vi "CPT Control 12.1.vi"() -> ()   [LabVIEW 2015]
uses:
  <vilib>/Analysis/baseanly.llb/Mean (DBL).vi
  <vilib>/Analysis/baseanly.llb/Normalize Vector.vi
  <vilib>/Utility/file.llb/Read From Spreadsheet File (string).vi
  <vilib>/Utility/file.llb/Write To Spreadsheet File (string).vi
  <vilib>/Utility/file.llb/Write To Spreadsheet File (DBL).vi
  <vilib>/Analysis/2dsp.llb/1D Cross Correlation (DBL).vi
  <vilib>/Utility/file.llb/Read Delimited Spreadsheet (DBL).vi
  <vilib>/Analysis/NI_AALBase.lvlib
  <vilib>/Analysis/NI_AALPro.lvlib
panel:
  in  "Set volume change threshold":bool
  out "size(s) 2":i32
  out "size(s)":i32
  in  "fre3":dbl
  out "Pore Offset:":dbl
  out "Side Offset:":dbl
  out "Axial Offset:":dbl
  in  "SET Pump Offsets":bool
  in  "Pore Offset SOLL":dbl
  in  "Side Offset Soll":dbl
  in  "Axial Offset Soll":dbl
  out "Stop Distance IS":dbl min=0.0 max=20.0 format="%#_f mm"
  in  "Stop Distance":dbl=20.0 min=0.0 max=20.0 format="%#_g mm"
  out "reset_flag":bool
  out "Time Loop":u32 format="%.0f ms"
  out "Pre-shearing output":dbl
  out "ms Offset":u32
  out "Test Flag":bool
  out "Date/Time:":string
  in  "Notaus":bool
  in  "Settings Tab":T1(tab)
  out "Axial Pressure":T2(graph)
  out "Side Pressure":T2(graph)
  out "Pore Pressure":T2(graph)
  in  "Visualize data":bool
  in  "SET Pump Pressures":bool
  out "Porepressure":dbl format="%#_4f kPa"
  out "Axialpressure":dbl format="%#_4f kPa"
  out "Sidepressure":dbl format="%#_4f kPa"
  in  "Soll Pore Pressure":dbl min=-200.0 max=4900.0 format="%#_3f kPa"
  in  "Soll Axial Pressure":dbl min=-200.0 max=4000.0 format="%#_3f kPa"
  in  "Soll Side Pressure":dbl min=-200.0 max=4000.0 format="%#_3f kPa"
  in  "Activate Manuel Control":bool
  in  "Schieberegler":dbl(slide) min=-1.0 max=1.0 scale=1.0..-1.0
  out "Position Piston":dbl(slide)
  in  "Move":bool
  out "Contact?":bool
  out "Force Sensor":dbl format="%#_4g N"
  in  "Go - Seitendruck":bool
  in  "Go - Axialdruck":bool
  in  "Velocity Linear":dbl=200.0 format="%#_g kPa/Min"
  in  "Up_Lower":bool
  in  "Delta Pore":dbl format="%#_g kPa"
  in  "GO All Pressure":bool
  in  "Delta Seiten":dbl format="%#_g kPa"
  in  "Delta Axial":dbl format="%#_g kPa"
  in  "Go - Porendruck":bool
  out "Velocity deviation":T3(graph)
  out "Acceleration":T3(graph)
  in  "Enable static penetration":bool
  in  "Finish test":bool
  in  "Set file":bool
  in  "Static peneration test":path
  in  "Vibro test 3":path
  in  "Vibro test 1":path
  in  "Static penetration Depth(mm) - 4":dbl
  in  "Time delay - 4":dbl
  in  "Enable Vibro Mode 2":bool
  in  "Enable Vibro Mode 3":bool
  in  "Depth(mm)3":dbl
  in  "Background velocity-3":dbl
  in  "Amplitdue-3":dbl
  in  "freq-3 ( Hz) 2":dbl
  in  "Time delay-3":dbl
  in  "Depth(mm)2":dbl
  in  "Background velocity-2":dbl
  in  "Amplitdue-2":dbl
  in  "freq-2 ( Hz)":dbl
  in  "Switch Vibro Mode":bool
  in  "Control start":bool
  in  "Control Stop":bool
  in  "Activate":bool
  out "Velocity vs Controller output":cluster{dbl[], dbl[]}[](graph)
  out "Correlation curve":dbl[](graph)
  out "time shift steps":sgl format="%.2f"
  in  "Visualize data":bool
  in  "Start Correlation":bool
  out "Intercept b":dbl
  out "Slope m":dbl
  in  "Time delay-2":dbl
  in  "Enable Vibro Mode 1":bool
  in  "Vibration frequency - 1  (Hz)":dbl
  in  "background velocity -1 (mm/s)":dbl
  in  "Amplitude - 1 (mm)":dbl
  in  "Vibro test 2":path
  in  "SET P/I Value":bool
  in  "Set auto file name":bool
  in  "SET Vibro Settings":bool
  out "Vibro Test IS":bool
  out "Frequency IS":dbl min=0.0 max=40.0 format="%#_g Hz"
  out "Amplitude IS":dbl=1.0 min=0.0 max=40.0 format="%#_g mm"
  out "Feeding IS":dbl min=0.0 max=20.0 format="%#_f mm/s"
  in  "New Path":string
  out "Path Logging":path
  in  "Set New Path":bool
  in  "VibroTest":bool=TRUE
  in  "Frequency SOLL":dbl=5.0 min=0.0 max=40.0 format="%#_g Hz"
  in  "Amplitude SOLL":dbl=3.0 min=0.0 max=40.0 format="%#_g mm"
  in  "Vorschub SOLL":dbl=20.0 min=0.0 max=20.0 format="%#_g mm/s"
  in  "Record Data":bool
  out "Record Flag":bool
  in  "start penetration":bool
  out "Boolean":bool
  in  "Soll I-Value":i32 min=-200 max=4000
  in  "Soll P-Value":i32 min=-200 max=4900
  out "IS I-Value":i32
  out "IS P-Value":i32
  out "Axial Pressure okay:":bool
  out "Side Pressure okay:":bool
  out "Pore Pressure okay:":bool
  in  "Circumference Control":bool
  in  "Turn off BC5":bool
  in  "SET Pre-Shearing":bool
  in  "Number of Cycles SOLL":dbl format="%#_f"
  in  "Duration of Cycle SOLL":i32
  in  "Amplitude Cycle SOLL":i32
  in  "Start Pre-Shearing":bool
  out "Pre-Shearing Ended Successful:":bool
  in  "Sollwert Porenwasser":dbl
  in  "Sollwert Seitendruck":dbl
  in  "Huang Su Calibration File":path
  out "IS Parameter 1":dbl=-163.9 format="%#_g x^6 +"
  out "IS Parameter 2":dbl=-163.9 format="%#_g x^5 +"
  out "IS Parameter 3":dbl=-163.9 format="%#_g x^4 +"
  out "IS Parameter 4":dbl=-163.9 format="%#_g x^3 +"
  out "IS Parameter 5":dbl=-163.9 format="%#_g x^2 +"
  out "IS Parameter 6":dbl=-163.9 format="%#_g x     +"
  out "IS Parameter 7":dbl=-163.9
  in  "SET Huang Su":bool
  in  "SOLL Parameter 1":dbl=-163.9 format="%#_g x^6 +"
  in  "SOLL Paramter 2":dbl=-163.9 format="%#_g x^5 +"
  in  "SOLL Parameter 3":dbl=-163.9 format="%#_g x^4 +"
  in  "SOLL Parameter 4":dbl=-163.9 format="%#_g x^3 +"
  in  "SOLL Parameter 5":dbl=-163.9 format="%#_g x^2 +"
  in  "SOLL Parameter 6":dbl=-163.9 format="%#_g x     +"
  in  "SOLL Parameter 7":dbl=-163.9
  out "Piston Position (mm)":dbl[](graph)
  out "Linear calibration":cluster{"array":dbl[], "array":dbl[]}(graph)
  in  "Calibration start":bool
  in  "Soll Slope-Strain":dbl
  in  "Soll Intercept-strain":dbl
  in  "Set button":bool
  out "IS-ADWIN":dbl
  out "IS- ADWIN":dbl
  in  "Initial cone position (mm)":dbl
  in  "Starting penetration depth (mm)  2":dbl
  in  "initial radius r0":dbl
  out "Timer Leackage":dbl format="%#_g s"
  out "Axial Leackage":dbl format="%.2f ml/m"
  out "Side Leackage":dbl format="%.2f ml/m"
  out "Pore Leackage":dbl format="%.2f ml/m"
  in  "Reset Leackage":bool
  out "Axial Kp:":dbl=40.0
  out "Axial Ki:":dbl format="%.2f"
  out "Side Kp:":dbl=40.0
  out "Side Ki:":dbl format="%.2f"
  out "Pore Kp:":dbl=40.0
  out "Pore Ki:":dbl format="%.2f"
  in  "SET Pump Controls":bool
  out "Modus":i32
  in  "Kpa":dbl=40.0
  in  "Kia":dbl=0.2 format="%.1f"
  in  "Kps":dbl=40.0
  in  "Kis":dbl=0.2 format="%.1f"
  in  "Kpp":dbl=40.0
  in  "Kip":dbl=0.2 format="%.1f"
  in  "Set":bool
  out "Side Offset: 2":dbl
  out "Axial Offset: 2":dbl
  out "Pore Offset: 2":dbl
  in  "Axial Offset Soll 2":dbl
  in  "Side Offset Soll 2":dbl
  in  "Pore Offset SOLL 2":dbl
  out "ms Offset Pre-Shearing":u32
  out "Seitendruck save":dbl format="%#.0f"
  out "Axialdruck save":dbl format="%#.0f"
  out "Porendruck save":dbl format="%#.0f"
  in  "View Tab":T4(tab)
  in  "Reset_left_graph":bool
  out "Recording":bool
  out "LVDT 3":dbl format="%0.3f mm"
  out "LVDT 2":dbl format="%0.3f mm"
  out "ml Pore Linear":dbl(slide) scale=0.0..1015.0
  out "ml Side Linear":dbl(slide) scale=0.0..1009.0
  out "ml Axial Linear":dbl(slide) scale=0.0..1014.5
  out "Pore":dbl format="%#_4g ml"
  out "Side":dbl format="%#_4g ml"
  out "Axial":dbl format="%#_4g ml"
  out "Addional Side Pressure":dbl format="%.2f kPa"
  out "Max Expansion":dbl format="%.2f mm"
  out "LVDT 1":dbl format="%0.3f mm"
  in  "Regelung Akiv Axial":bool
  in  "Regelung Akiv Sidepressure":bool
  in  "Regelung Akiv Porepress":bool
  out "Axial Pressure  [KPa]":dbl format="%#.2f kPa"
  out "Side Pressure  [KPa]":dbl format="%#.2f kPa"
  out "Pore Pressure [KPa]":dbl format="%#.2f kPa"
  out "ml Fontpanel":cluster{"mean":dbl, "mean":dbl, "mean":dbl}(graph)
  out "LVDT Frontpannel":cluster{"mean":dbl, "mean":dbl, "mean":dbl}(graph)
  out "Interner Kraftsensor [MPa]":cluster{"Y":dbl[], "Y":dbl[]}[](graph) caption="XY-Graph"
  out "Notaus Activ":bool
  out "Linear Control On":bool
  out "Test Started":bool
  out "Ready":bool
  out "Manuel Control":bool
  out "Pump Control On":bool
  out "Hold Position":bool
  out "Test ended":bool
  out "Penetration ongoing":bool
  out "Cone Tip Resistance":dbl format="%0.2f"
  out "Pore Pressure":dbl format="%0.2f"
  in  "Activate Pumps/Piston Controls":bool
  out "Cone Pressure":cluster{dbl, "mean":dbl}(graph)
  out "Distance Graph":T2(graph)
  out "Linear regression":cluster{dbl[], dbl[]}[](graph)
  out "Controller Output":T2(graph)
  out "Displacement control error (mm)":dbl[](graph)
  out "Regelung Out":dbl(graph)
  out "Valve Is":dbl(graph)
  out "SOLL IS Distance":cluster{dbl, dbl}(graph)
  in  "Stop/Start":bool
  out "Axialdruck [Pa] 4":dbl(graph)
  out "Seitendruck [Pa] 3":dbl(graph)
  out "Porendruck [Pa] 2":dbl(graph)
  in  "Reset Alarm":bool
  out "Side Alarm":bool
  in  "Erlaubte Max Abweichung Side":dbl
  in  "Erlaubte  Max Abweichung Pore":dbl
  in  "Erlaubte Max Abweichung Axial":dbl
  out "Sollvorgabe":T5(graph)
  out "S":u32
  out "Total Elapsed Seconds":dbl
  out "Alarm Triggered":bool
  out "Abweichung Side":dbl format="%#_4g"
  out "Pore Alarm":bool
  out "Axial Alarm":bool
  out "Abweichung Pore":dbl format="%#_4g"
  out "Abweichung Axial":dbl format="%#_5g"
  in  "volumetric strain":dbl
  in  "Display":bool
  out "Side volume - Effective lateral Stress":cluster{"Y":dbl[], "Y":dbl[]}[](graph)
  in  "LCT control finish":bool
  out "LCT test finish":bool
  out "Strain curve based on side volume change":sgl(graph)
  in  "LCT strain-based control activate":bool
  out "Change of side volume (ml)/ actual volumetric strain":sgl format="%.2f"
  in  "maximum acceptable \nside volume change (ml)":dbl
  in  "Trigger condition\n of Stop loading":T6(ring)=enum."Set volume change threshold"
  # "Activate Manuel Piston Control"
  # "Velocity Piston"
  # "Up"
  # "Down"
  # "IS-ADwin:"
  # "Set Value:"
  # "Pore Pressure:"
  # "Side Pressure"
  # "Axial Pressure"
  # "Linear Pressure Control"
  # "Decreasing"
  # "Increasing"
  # "Delta Pore"
  # "Delta Side"
  # "Delta Axial"
  # "Vibro Settings"
  # "IS-ADwin:"
  # "Set Value:"
  # "Feeding:"
  # "Vibro Test ON:"
  # "Amplitude:"
  # "Frequency:"
  # "Controller Settings"
  # "IS-ADwin:"
  # "Set Value:"
  # "Kp:"
  # "Ki:"
  # "End of Test"
  # "IS-ADwin:"
  # "Set Value:"
  # "IS-ADwin:"
  # "Set Value:"
  # "Leackage Indicator"
  # "IS-ADwin:"
  # "Set Value:"
  # "Control"
  # "Pressure"
  # "reset"
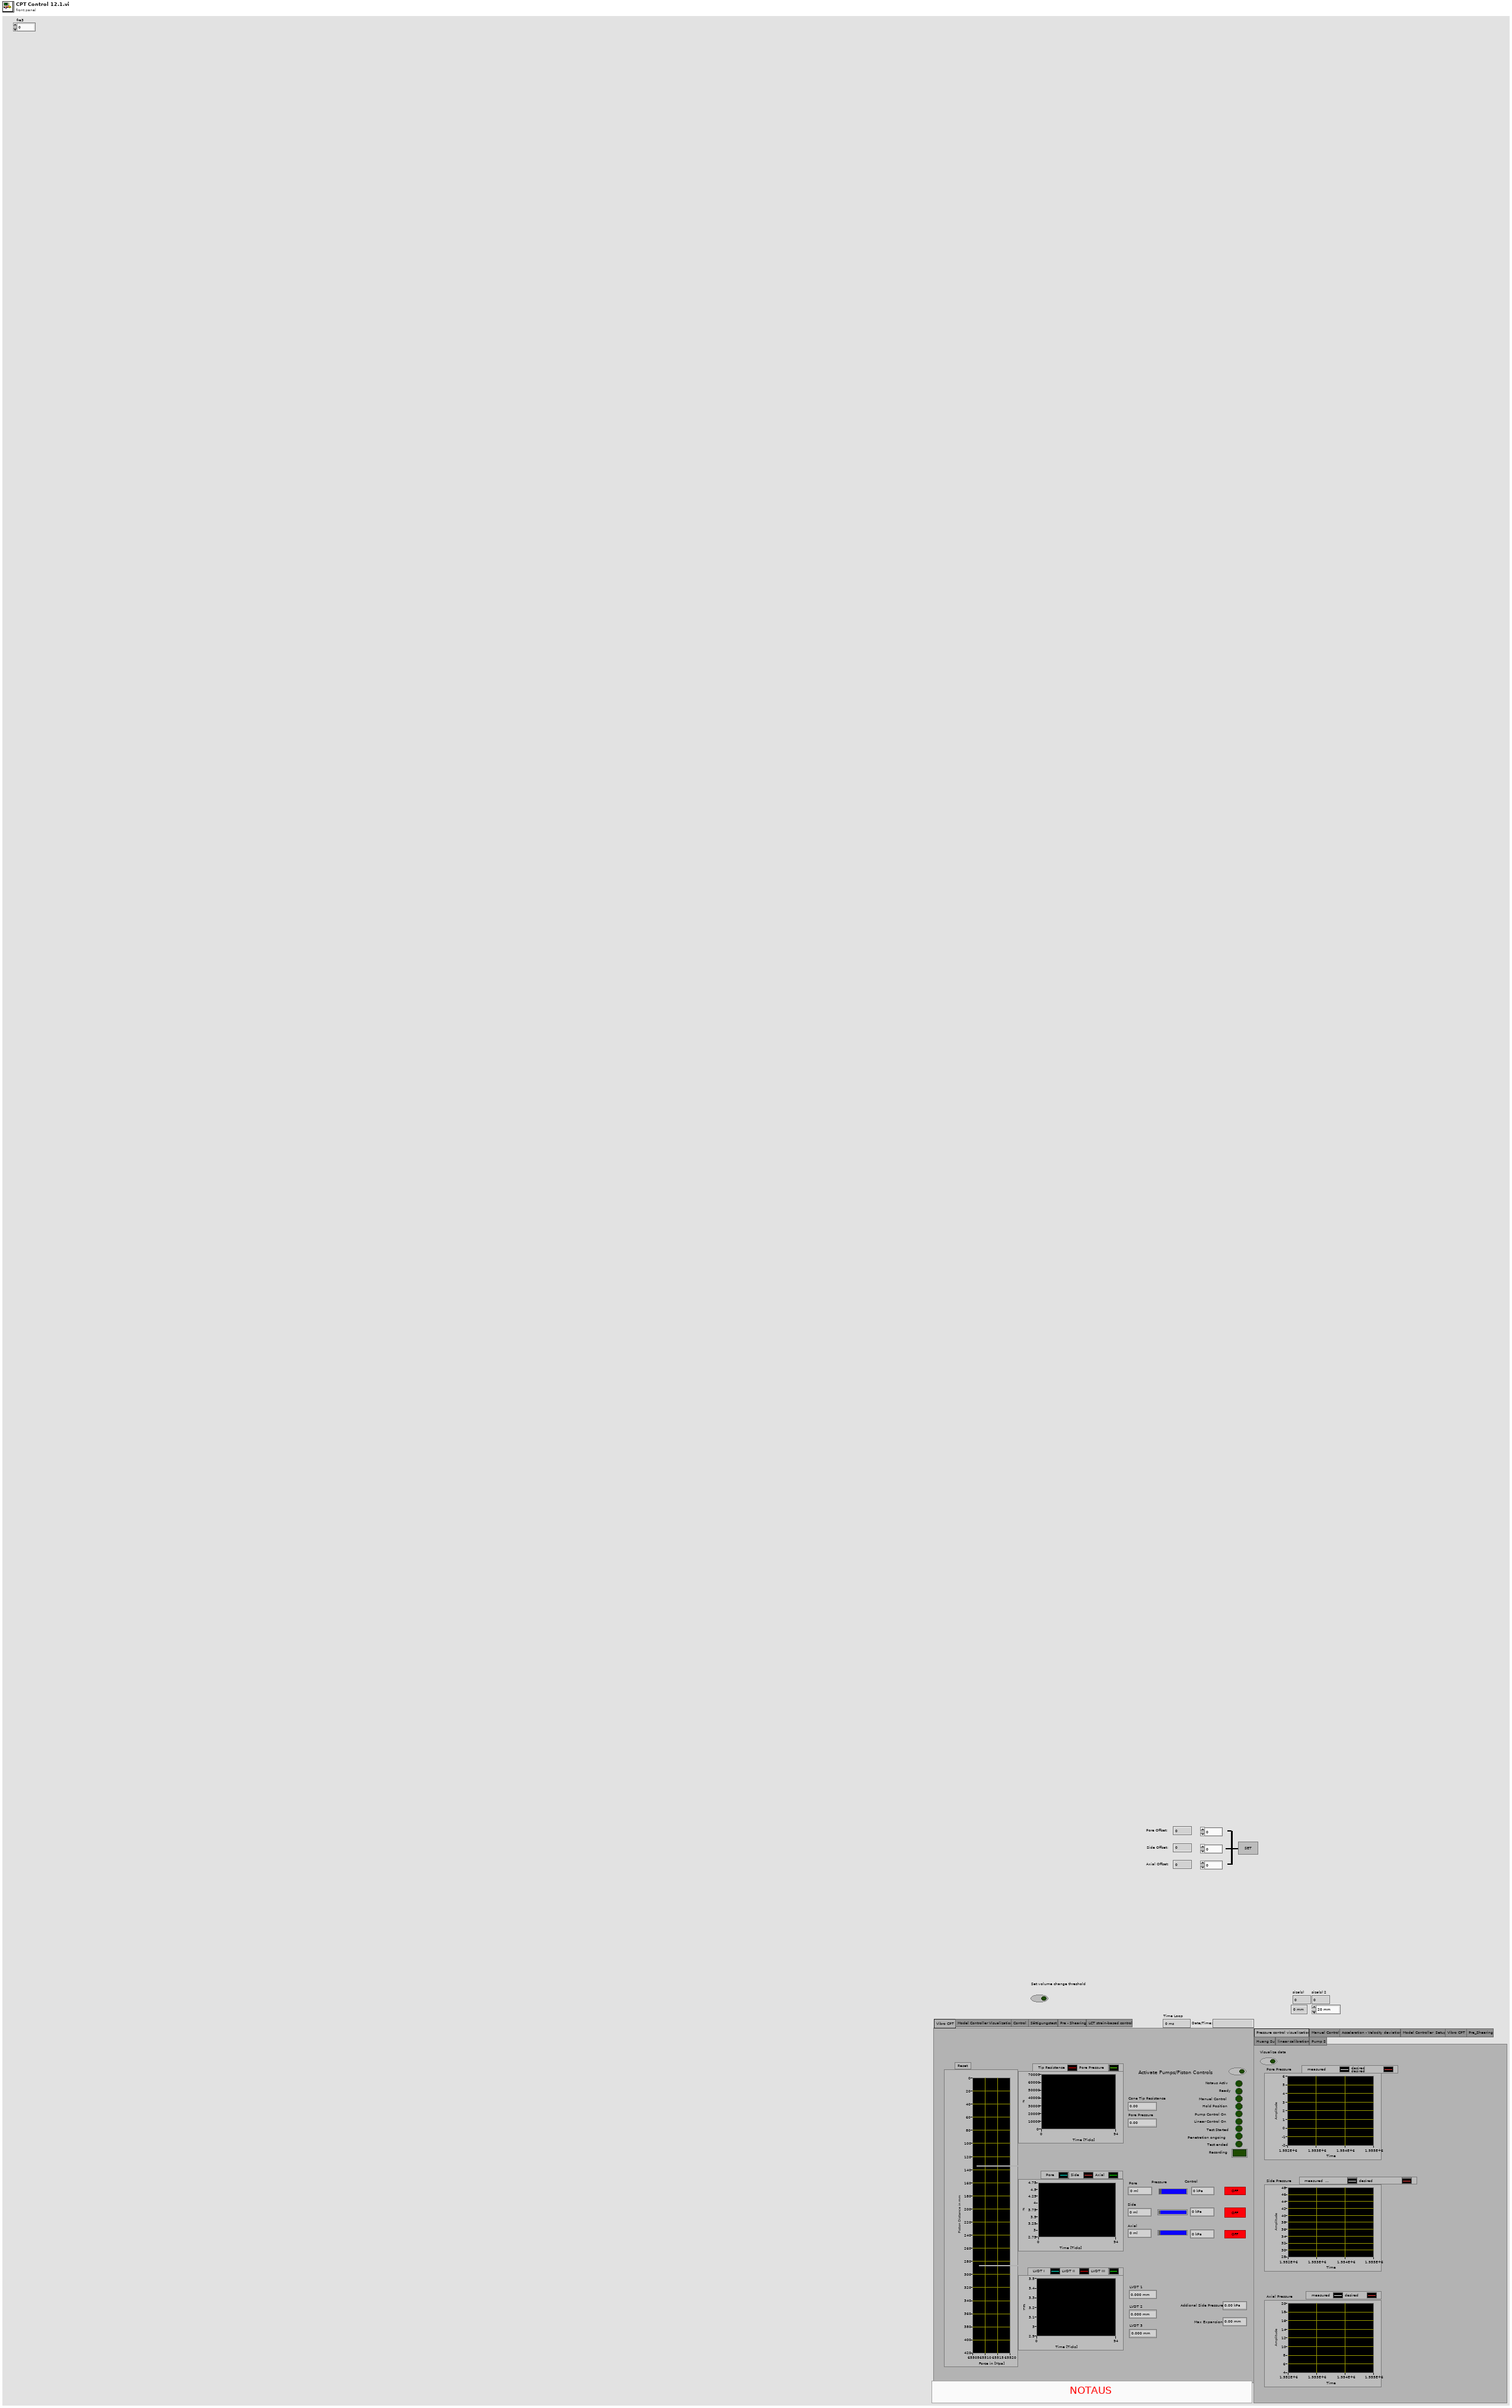
[diagram p1: front panel]
types:
  T1 = enum32{"Pressure control visualization", "Manuel Control", "Acceleration - Velocity deviation", "Model Controller  Setup", "Vibro CPT", "Pre_Shearing", "Huang Su", "linear calibration", "Pump S"}
  T2 = cluster{"Output Array":dbl[], "Output Array":dbl[]}[]
  T3 = cluster{"Output Array":dbl[], "Output Array 2":dbl[]}
  T4 = enum32{"Vibro CPT", "Model Controller Visualization", "Control", "Sättigungstest", "Pre - Shearing", "LCT strain-based control"}
  T5 = cluster{"Axial Pressure  [KPa]":dbl, "Pre-shearing output":dbl}
  T6 = enum16{"set strain for pore\n volume tric strain", "Set volume change threshold"}
  T7 = enum8{"Enabled", "Disabled", "Disabled and Grayed Out"}
  T8 = enum16{"Program Counter", "Force ", "Position Induktiv", "Position Laser", "Laser 01", "Axial Stellwert", "LVDT 1", "LVDT 2", "LVDT 3", "Pore Pressure", "Side Pressure ", "Axial Pressure", "Pore Volumen", "Side Volumen ", "Axial Volumen ", "NaN", "LVDT Max", "Side Addtional Pressure", "Stellwert Regler", "Cone  Pore Pressure ", "Cone  Side Pressure ", "Valve Kolbenposition", "Regelanweichung", "Regelabweichung Summe ", ""}
  T9 = enum16{"Program Counter", "Force ", "Position Induktiv", "PorePress_regout", "SidePress_regout", "AxialPress_regout", "LVDT 1", "LVDT 2", "LVDT 3", "Pore Pressure", "Side Pressure ", "Axial Pressure", "Pore Volumen", "Side Volumen ", "Axial Volumen ", "Soll_Porepress", "Soll_Sidepress", "Soll_axialpress", "LVDT_max", "desired distance", "predict distance", "fitted velocity", "Valve IST", "Tip resistance", "Pore pressure", "Distance_Regout", "velocity data", "estimated_Distance_Regout", "normalize vel", "normalize Distance_regout", "strain", "additional side pressure", "initial_depth", "Distance_digital", "initial volume", "actual volume", "actual side volume"}
  T10 = enum16{"NaN", "WegInd_Digits", "Valve_IST", "KraftHTM_Digits", "WegInd_Delta", "WegLaser_Digits", "Laser_O1", "Laser_M3", "LVDT_2", "LVDT_3", "LVDT_1", "PorePress_Digits", "AxialPress_Digits", "SidePress_Digits", "SpindelA_Digits", "SpindelB_Digits", "SpindelC_Digits", "FPAR_17", "Slope_calibration", "Intercept_calibration", "PorePressOffset", "AxialPressOffset", "SidePressOffset", "FPAR_23", "FPAR_24", "Vorschub", "Sinusfrequenz_Vibro", "Amplitude_Vibro", "PreShearingOutput", "FPAR_29", "FPAR_30", "FPAR_31", "FPAR_32", "FPAR_33", "FPAR_34", "FPAR_35", "FPAR_36", "FPAR_37", "FPAR_38", "FPAR_39", "Kp_Porepress", "Ki_Porepress", "Kp_Sidepress", "Ki_Sidepress", "Kp_Axialpress", "Ki_Axialpress", "FPAR_46", "FPAR_47", "FPAR_48", "FPAR_49", "FPAR_50", "PaProMin", "FPAR_52", "FPAR_53", "FPAR_54", "Huang_Su_par_1", "Huang_Su_par_2", "Huang_Su_par_3", "Huang_Su_par_4", "Huang_Su_par_5", "FPAR_60", "FPAR_61", "Huang_Su_par_6", "Huang_Su_par_7", "FPAR_64", "FPAR_65", "FPAR_66", "Model_PreShearing", "Model_Vibro", "FPAR_69", "FPAR_70", "FPAR_71", "Set_Soll_PorePressure", "Set_Soll_AxialPressure", "Set_Soll_SidePressure", "Soll_PorePressure", "Soll_AxialPressure", "Soll_SidePressure", "Taktzeit", "Abtastfrequenz", "Clock"}
  T11 = enum16{"NaN", "WegInd_Digits", "Valve_IST", "KraftHTM_Digits", "WegInd_Delta", "WegLaser_Digits", "Laser_O1", "Laser_M3", "LVDT_2", "LVDT_3", "LVDT_1", "PorePress_Digits", "AxialPress_Digits", "SidePress_Digits", "SpindelA_Digits", "SpindelB_Digits", "SpindelC_Digits", "FPAR_17", "FPAR_18", "FPAR_19", "PorePressOffset", "AxialPressOffset", "SidePressOffset", "FPAR_23", "FPAR_24", "Vorschub", "Sinusfrequenz_Vibro", "Amplitude_Vibro", "PreShearingOutput", "FPAR_29", "FPAR_30", "FPAR_31", "FPAR_32", "FPAR_33", "FPAR_34", "FPAR_35", "FPAR_36", "FPAR_37", "FPAR_38", "FPAR_39", "Kp_Porepress", "Ki_Porepress", "Kp_Sidepress", "Ki_Sidepress", "Kp_Axialpress", "Ki_Axialpress", "FPAR_46", "FPAR_47", "FPAR_48", "FPAR_49", "FPAR_50", "PaProMin", "FPAR_52", "FPAR_53", "FPAR_54", "Huang_Su_par_1", "Huang_Su_par_2", "Huang_Su_par_3", "Huang_Su_par_4", "Huang_Su_par_5", "FPAR_60", "FPAR_61", "Huang_Su_par_6", "Huang_Su_par_7", "FPAR_64", "FPAR_65", "FPAR_66", "Model_PreShearing", "Model_Vibro", "FPAR_69", "FPAR_70", "FPAR_71", "Set_Soll_PorePressure", "Set_Soll_AxialPressure", "Set_Soll_SidePressure", "Soll_PorePressure", "Soll_AxialPressure", "Soll_SidePressure", "Taktzeit", "Abtastfrequenz", "Clock"}
  T12 = enum16{"NaN", "WegInd_Digits", "Valve_IST", "KraftHTM_Digits", "WegInd_Delta", "WegLaser_Digits", "Laser_O1", "Laser_M3", "LVDT_2", "LVDT_3", "LVDT_1", "PorePress_Digits", "AxialPress_Digits", "SidePress_Digits", "SpindelA_Digits", "SpindelB_Digits", "SpindelC_Digits", "FPAR_17", "FPAR_18", "FPAR_19", "PorePressOffset", "AxialPressOffset", "SidePressOffset", "FPAR_23", "FPAR_24", "Vorschub", "Sinusfrequenz_Vibro", "Amplitude_Vibro", "PreShearingOutput", "FPAR_29", "FPAR_30", "FPAR_31", "volume change/ pore volumetric strain ", "actual side volume change / actual pore volumetric strain ", "FPAR_34", "FPAR_35", "FPAR_36", "FPAR_37", "FPAR_38", "FPAR_39", "Kp_Porepress", "Ki_Porepress", "Kp_Sidepress", "Ki_Sidepress", "Kp_Axialpress", "Ki_Axialpress", "FPAR_46", "FPAR_47", "FPAR_48", "FPAR_49", "FPAR_50", "PaProMin", "FPAR_52", "FPAR_53", "FPAR_54", "Huang_Su_par_1", "Huang_Su_par_2", "Huang_Su_par_3", "Huang_Su_par_4", "Huang_Su_par_5", "FPAR_60", "FPAR_61", "Huang_Su_par_6", "Huang_Su_par_7", "FPAR_64", "FPAR_65", "FPAR_66", "Model_PreShearing", "Model_Vibro", "FPAR_69", "FPAR_70", "FPAR_71", "Set_Soll_PorePressure", "Set_Soll_AxialPressure", "Set_Soll_SidePressure", "Soll_PorePressure", "Soll_AxialPressure", "Soll_SidePressure", "Taktzeit", "Abtastfrequenz", "Clock"}
  T13 = cluster{"Output Array":dbl[], "Output Array":dbl[]}
  T14 = cluster{"Output Array":dbl[], "normalized waveform":waveform(dbl)}
  T15 = cluster{"Output Array":dbl[], "normalized waveform":waveform(dbl)}[]
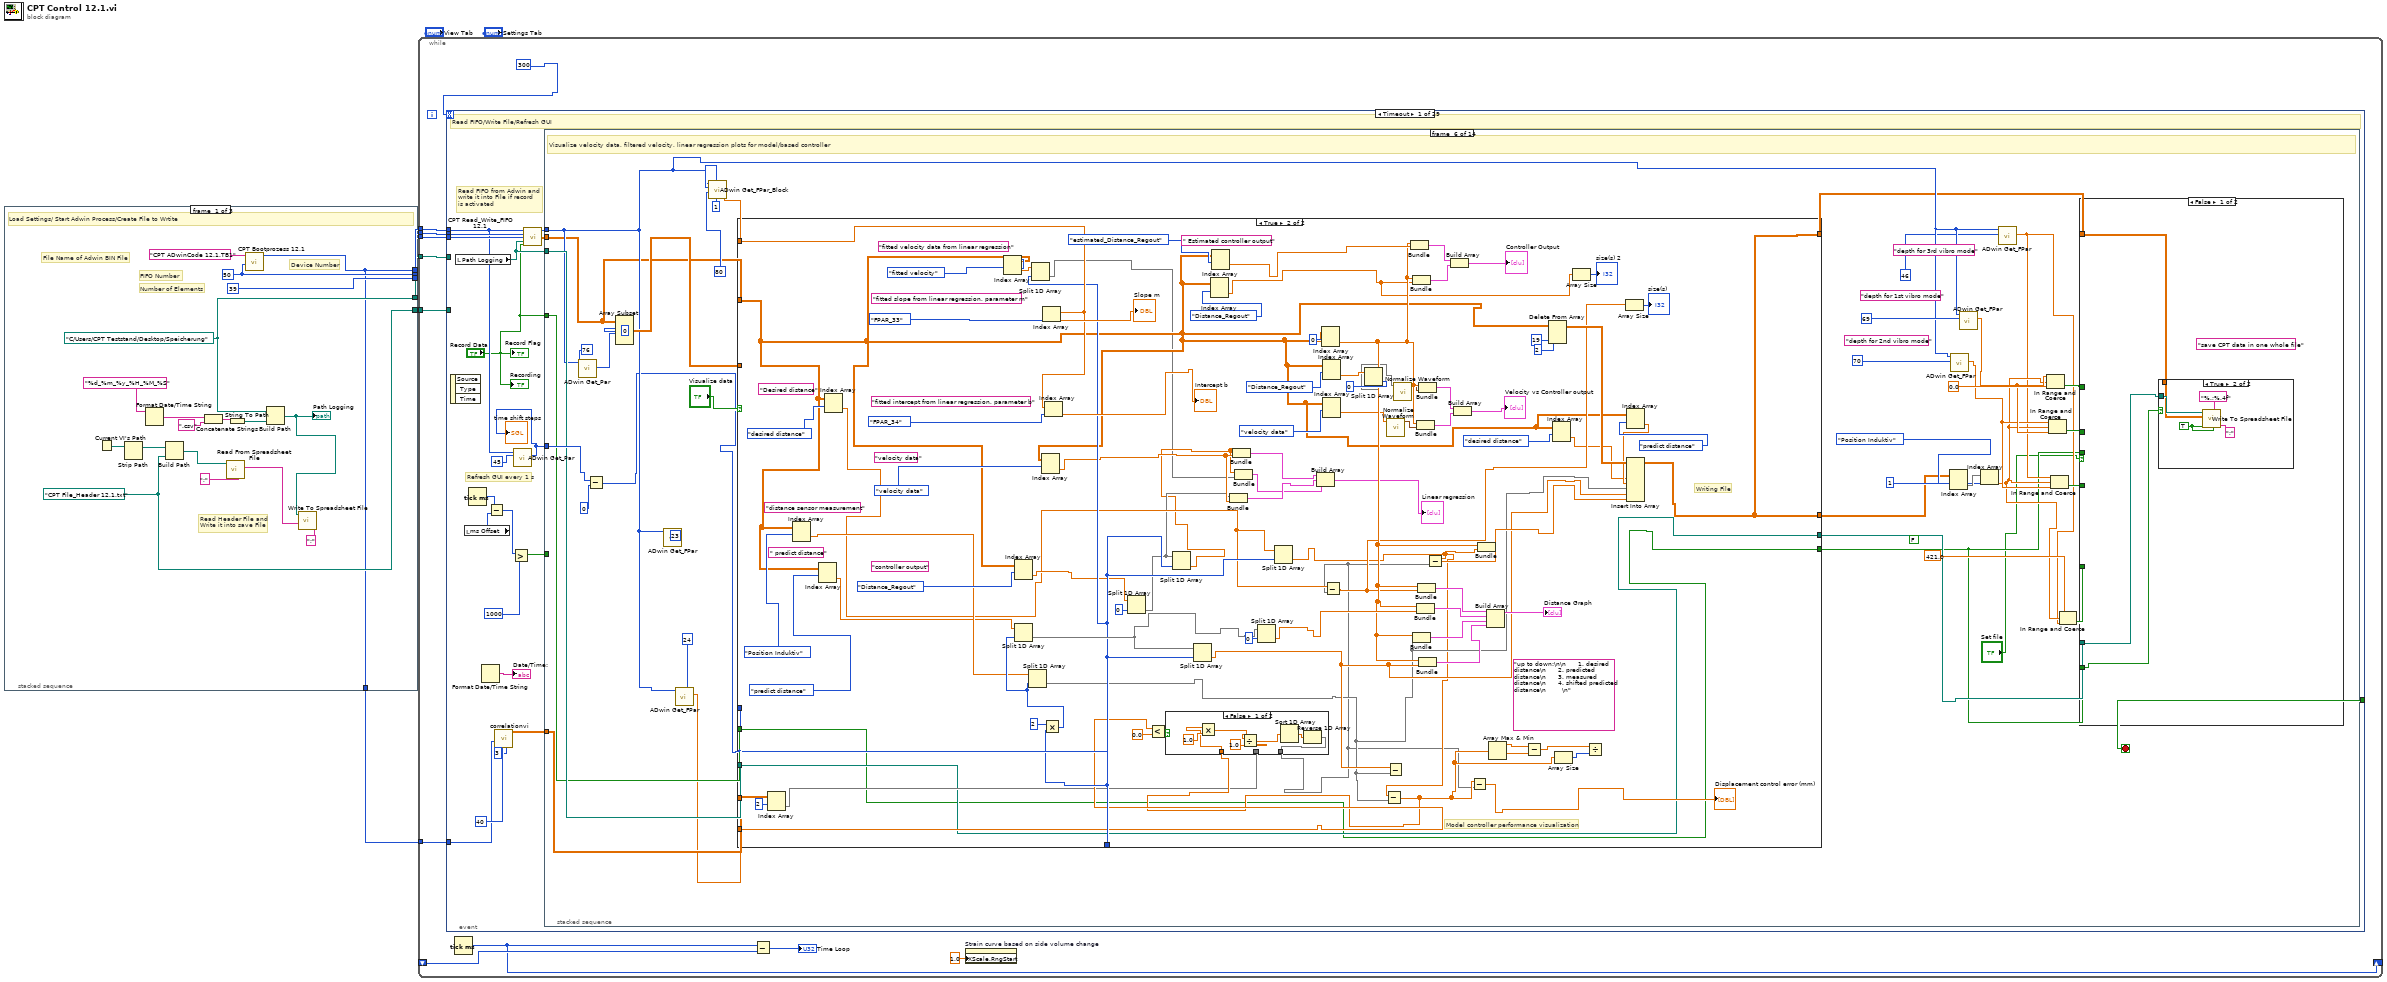
[diagram p0: block diagram]
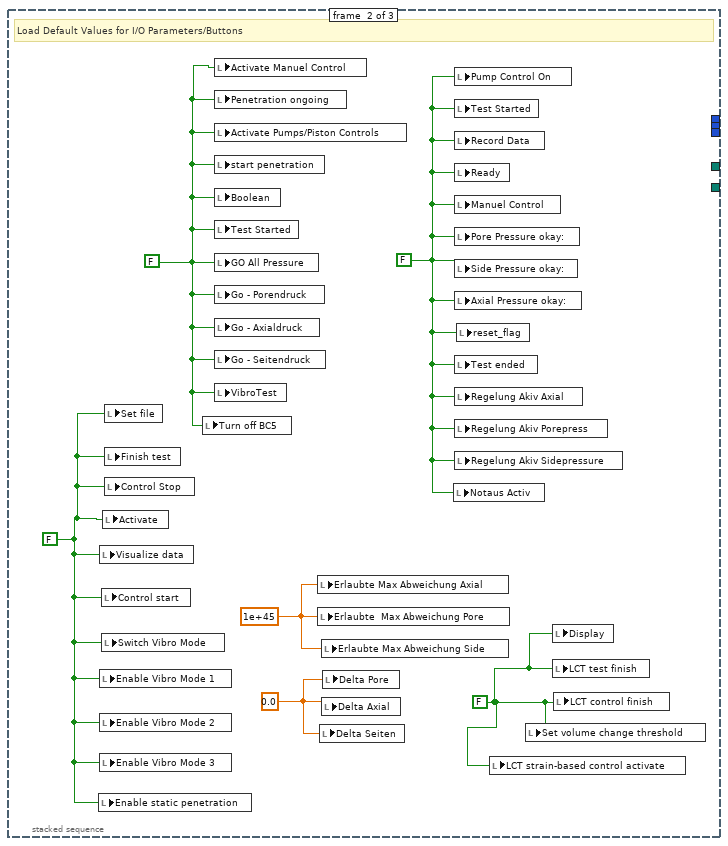
[diagram p2: hidden frame]
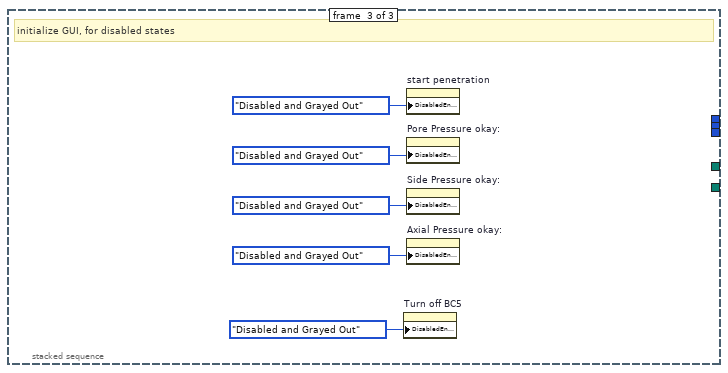
[diagram p3: hidden frame]
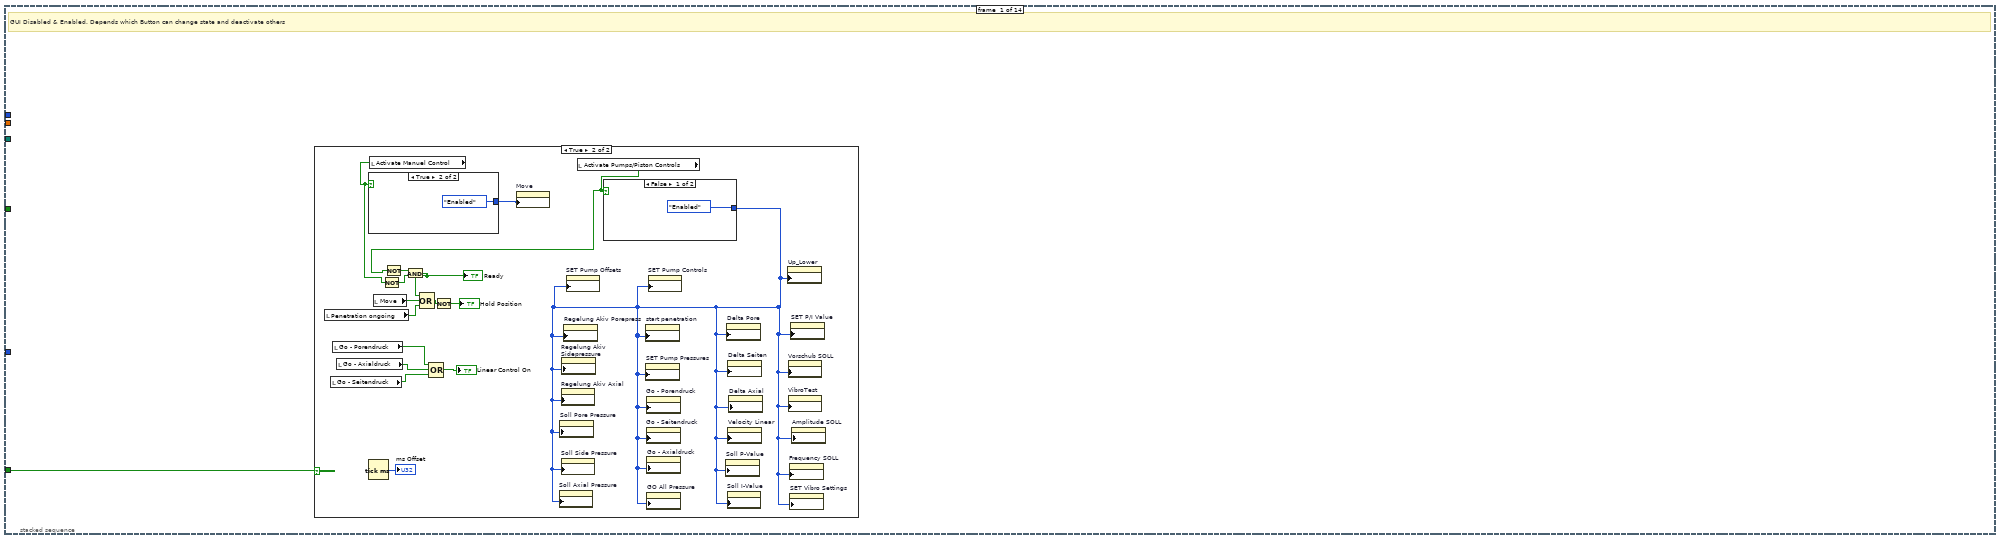
[diagram p4: hidden frame]
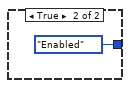
[diagram p6: hidden frame]
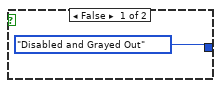
[diagram p7: hidden frame]
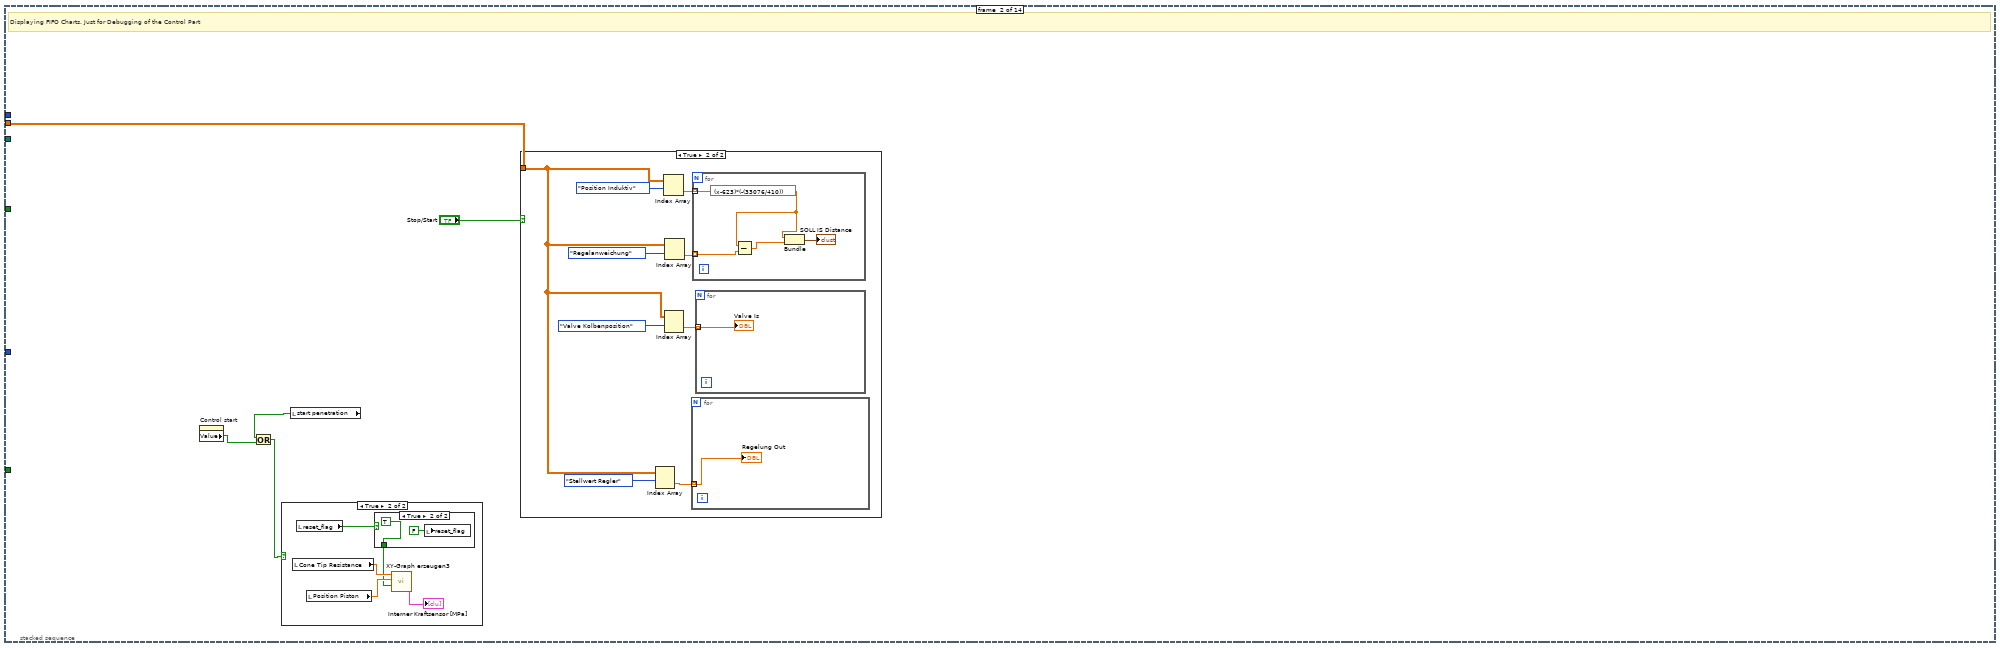
[diagram p8: hidden frame]
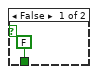
[diagram p10: hidden frame]
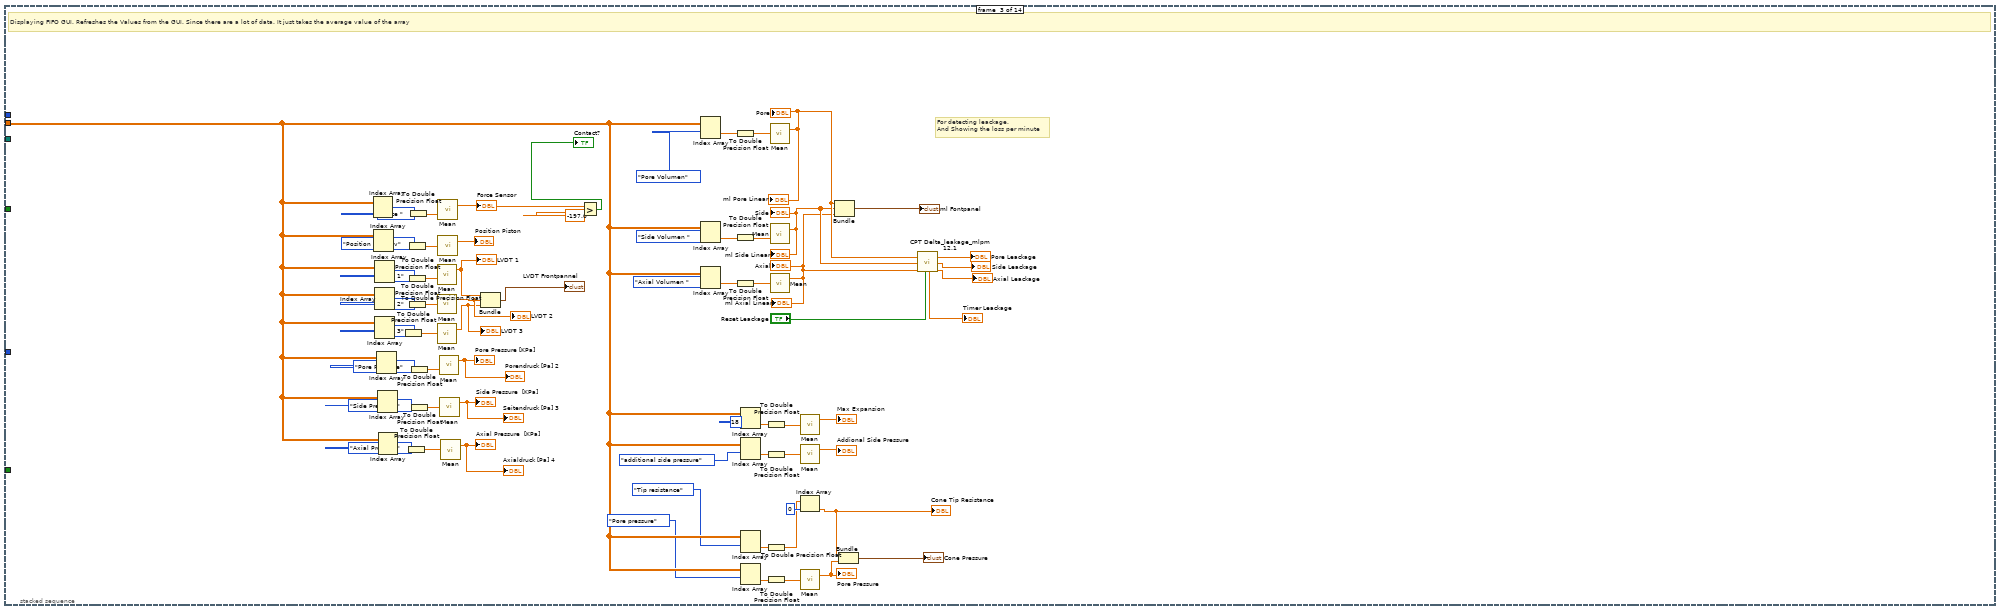
[diagram p12: hidden frame]
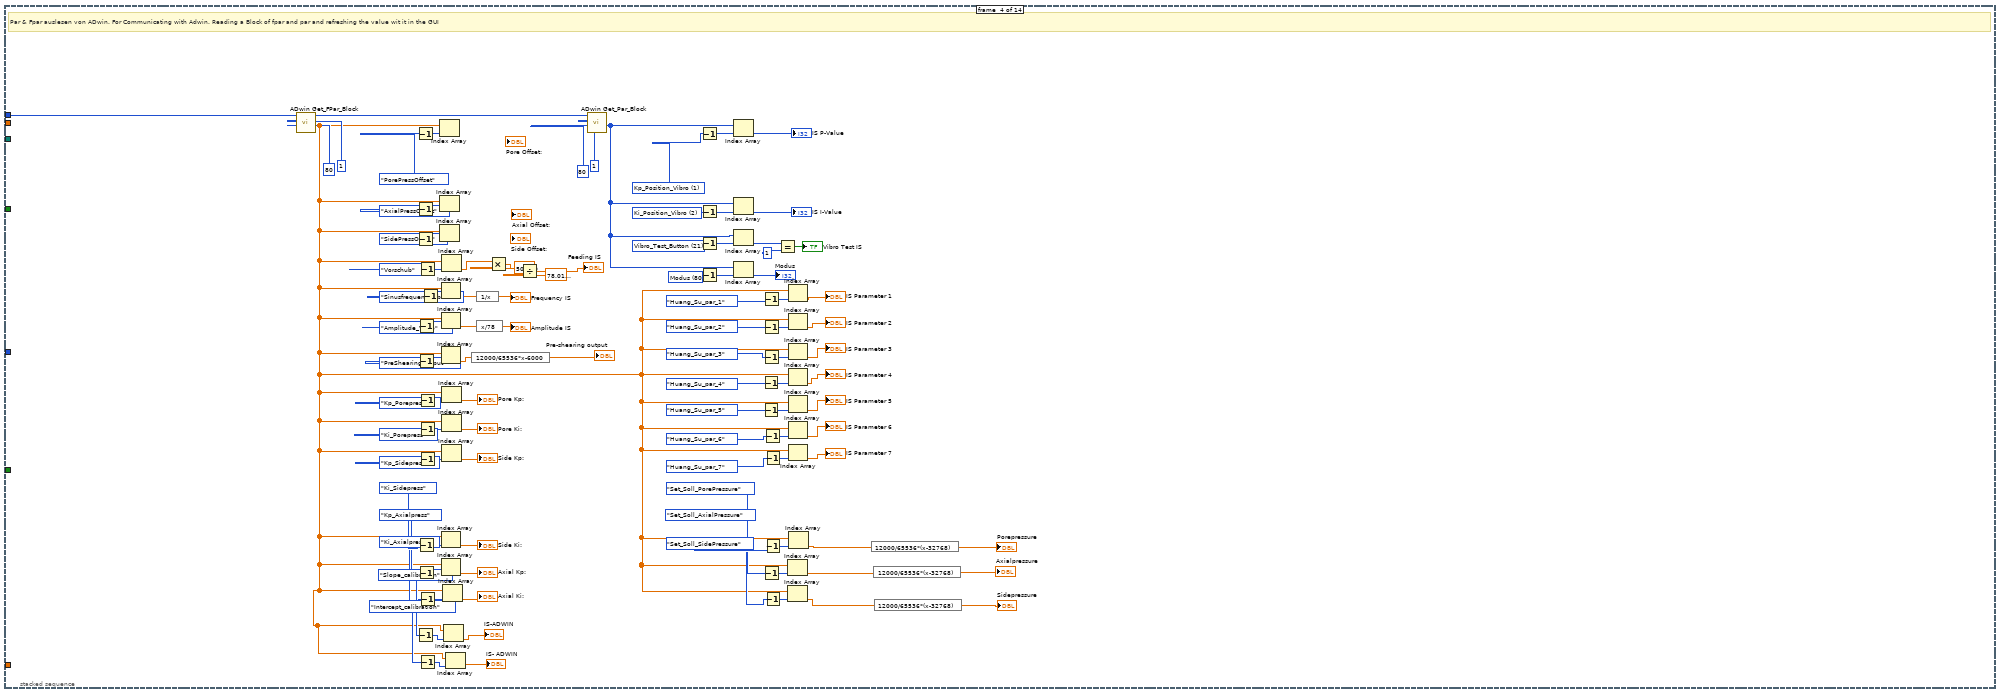
[diagram p13: hidden frame]
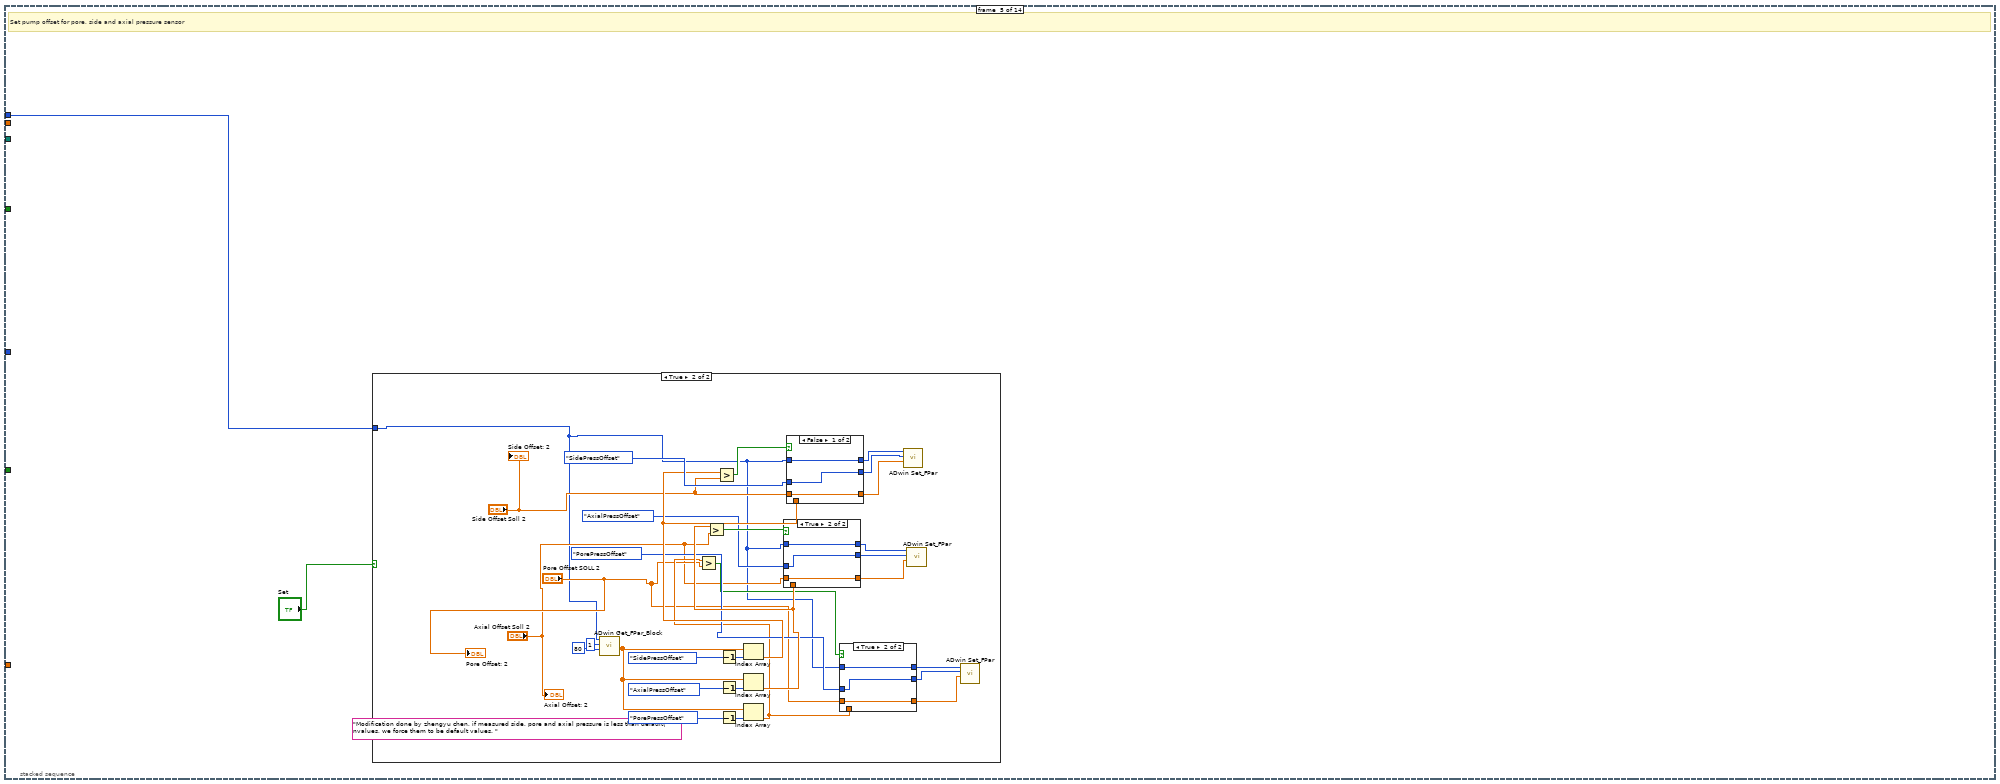
[diagram p14: hidden frame]
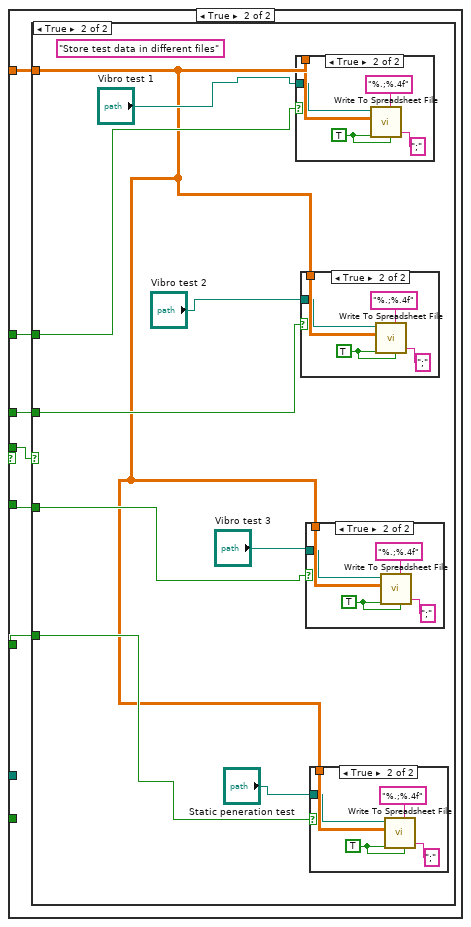
[diagram p20: hidden frame]
diagram:
  n1 = stacked-sequence {
    tunnel: [w7 _ _] -> w6
    tunnel: [w24 _ _] -> w5
    tunnel: [39 ("dimension size") _ _] -> w4
    tunnel: [w11 _ _] -> w3
    tunnel: [w9 _ _] -> w2
    tunnel: [w7 _ _] -> w1
    frame #0 {
      w9 = path "CPT File_Header 12.1.txt" ("Grundpfad")
      w24 = u16 50 ("FifoNo")
      w11 = path "C:/Users/CPT Teststand/Desktop/Speicherung" ("Grundpfad")
      # "Read Header File and \nWrite it into save File"
      # "File Name of Adwin BIN File"
      # "Device Number"
      # "Number of Elements"
      # "FIFO Number"
      # "Load Settings/ Start Adwin Process/Create File to Wrtite"
      n2 = Current VI's Path() -> (path=w14:path)
      n3 = Strip Path(path=w14) -> (stripped path=w13:path)  [unwired: 1 out]
      n4 = Format Date/Time String(time format string (%c)="%d_%m_%y_%H_%M_%S") -> (date/time string=w18:string)  [unwired: 2 in]
      n5 = Build Path(base path=w13, name or relative path=w9) -> (appended path=w15:path)
      n6 = Concatenate Strings(w18, ".csv" ("String")) -> (w21:string)
      n7 = call-poly <vilib>:"Read From Spreadsheet File.vi"("delimiter (\\t)"=";" ("delimiter (\\t)"), "file path (dialog if empty)"=w15) -> ("first row"=w16:string[])  [unwired: 5 in, 4 out]
      n8 = String To Path(string=w21) -> (path=w20:path)
      n9 = call "CPT Bootprozess 12.1.vi"("FifoNo"=w24, "Boot File Relative Referenz"="CPT ADwinCode 12.1.TB1" ("Filename")) -> ("Device No. out"=w7:u16)  [unwired: 8 in, 1 out]
      n10 = Build Path(base path=w11, name or relative path=w20) -> (appended path=w8:path)
      "Path Logging" <- w8
      n11 = call-poly <vilib>:"Write To Spreadsheet File.vi"("delimiter (\\t)"=";" ("delimiter (\\t)"), "1D data"=w16, "file path (dialog if empty)"=w8) -> ()  [unwired: 5 in, 1 out]
    }
    frame #1 {
      w26 = FALSE ("Freeze")
      w25 = FALSE ("Freeze")
      w28 = 1e+45 ("Abweichung Solll  - Ist")
      w29 = 0.0 ("Delta Pore")
      w30 = FALSE ("Boolean")
      w27 = FALSE ("Freeze")
      # "Load Default Values for I/O Parameters/Buttons"
      n12 = local write "Enable static penetration"(w25) -> ()
      n13 = local write "Visualize data"(w25) -> ()
      n14 = local write "Enable Vibro Mode 1"(w25) -> ()
      n15 = local write "Enable Vibro Mode 2"(w25) -> ()
      n16 = local write "Enable Vibro Mode 3"(w25) -> ()
      n17 = local write "Control start"(w25) -> ()
      n18 = local write "Switch Vibro Mode"(w25) -> ()
      n19 = local write "Activate"(w25) -> ()
      n20 = local write "Set file"(w25) -> ()
      n21 = local write "Finish test"(w25) -> ()
      n22 = local write "Control Stop"(w25) -> ()
      n23 = local write "Turn off BC5"(w30) -> ()
      n24 = local write "Activate Manuel Control"(w30) -> ()
      n25 = local write "Penetration ongoing"(w30) -> ()
      n26 = local write "Activate Pumps/Piston Controls"(w30) -> ()
      n27 = local write "start penetration"(w30) -> ()
      n28 = local write "Boolean"(w30) -> ()
      n29 = local write "Test Started"(w30) -> ()
      n30 = local write "GO All Pressure"(w30) -> ()
      n31 = local write "Go - Porendruck"(w30) -> ()
      n32 = local write "Go - Axialdruck"(w30) -> ()
      n33 = local write "Go - Seitendruck"(w30) -> ()
      n34 = local write "VibroTest"(w30) -> ()
      n35 = local write "Erlaubte Max Abweichung Axial"(w28) -> ()
      n36 = local write "Erlaubte  Max Abweichung Pore"(w28) -> ()
      n37 = local write "Delta Seiten"(w29) -> ()
      n38 = local write "Erlaubte Max Abweichung Side"(w28) -> ()
      n39 = local write "Delta Axial"(w29) -> ()
      n40 = local write "Delta Pore"(w29) -> ()
      n41 = local write "Notaus Activ"(w27) -> ()
      n42 = local write "Pump Control On"(w27) -> ()
      n43 = local write "Test Started"(w27) -> ()
      n44 = local write "Record Data"(w27) -> ()
      n45 = local write "Ready"(w27) -> ()
      n46 = local write "Manuel Control"(w27) -> ()
      n47 = local write "Pore Pressure okay:"(w27) -> ()
      n48 = local write "Side Pressure okay:"(w27) -> ()
      n49 = local write "Axial Pressure okay:"(w27) -> ()
      n50 = local write "Test ended"(w27) -> ()
      n51 = local write "Regelung Akiv Axial"(w27) -> ()
      n52 = local write "Regelung Akiv Porepress"(w27) -> ()
      n53 = local write "Regelung Akiv Sidepressure"(w27) -> ()
      n54 = local write "reset_flag"(w27) -> ()
      n55 = local write "LCT strain-based control activate"(w26) -> ()
      n56 = local write "Set volume change threshold"(w26) -> ()
      n57 = local write "Display"(w26) -> ()
      n58 = local write "LCT test finish"(w26) -> ()
      n59 = local write "LCT control finish"(w26) -> ()
    }
    frame #2 {
      # "initialize GUI, for disabled states"
      n60 = property on="Turn off BC5" class="Bool (strict)"("DisabledEnum"=T7."Disabled and Grayed Out" ("Disabled")) -> ()  [unwired: 2 in, 2 out]
      n61 = property on="start penetration" class="Bool (strict)"("DisabledEnum"=T7."Disabled and Grayed Out" ("Disabled")) -> ()  [unwired: 2 in, 2 out]
      n62 = property on="Pore Pressure okay:" class="Bool (strict)"("DisabledEnum"=T7."Disabled and Grayed Out" ("Disabled")) -> ()  [unwired: 2 in, 2 out]
      n63 = property on="Side Pressure okay:" class="Bool (strict)"("DisabledEnum"=T7."Disabled and Grayed Out" ("Disabled")) -> ()  [unwired: 2 in, 2 out]
      n64 = property on="Axial Pressure okay:" class="Bool (strict)"("DisabledEnum"=T7."Disabled and Grayed Out" ("Disabled")) -> ()  [unwired: 2 in, 2 out]
    }
  }
  n65 = while {
    tunnel: w6 -> [w38]
    shift-right: [w45] -> _
    shift-left: _ -> [w47]
    tunnel: w5 -> [w44]
    tunnel: w4 -> [w43]
    tunnel: w3 -> [w42]
    tunnel: w2 -> [w40]
    tunnel: w1 -> [w39]
    stop <- w41 stop-if-true
    n66 = event shown="[0] Timeout" {
      selector: _ -> [_ _ _ _ _ _ _ _ _ _ _ _ _ _ _ _ _ _ _ _ _ _ _ _ _ _ _ _ _]
      dyn-events: _ -> [_ _ _ _ _ _ _ _ _ _ _ _ _ _ _ _ _ _ _ _ _ _ _ _ _ _ _ _ _]
      timeout: 300 -> [_ _ _ _ _ _ _ _ _ _ _ _ _ _ _ _ _ _ _ _ _ _ _ _ _ _ _ _ _]
      tunnel: w38 -> [w55 _ _ w1003 w1009 w1061 w1074 w1079 w1088 w1095 _ w1148 w1184 w1195 _ w1269 _ w1296 w1304 w1318 w1322 w1332 w1342 w1350 w1367 w1407 w1430 w1440 w1485]
      tunnel: w44 -> [w66 _ _ _ _ _ _ _ _ _ _ _ _ _ _ _ _ _ _ _ _ _ _ _ _ _ _ _ _]
      tunnel: w43 -> [w65 _ _ _ _ _ _ _ _ _ _ _ _ _ _ _ _ _ _ _ _ _ _ _ _ _ _ _ _]
      tunnel: w42 -> [_ _ _ _ _ _ _ _ _ _ _ _ _ _ w1239 _ w1278 _ _ _ _ _ _ _ _ _ _ _ _]
      tunnel: [_ _ _ w1005 _ _ _ _ _ _ _ _ _ _ _ _ _ _ _ _ _ _ _ _ _ _ _ _ _] -> w41
      tunnel: w40 -> [_ _ _ _ _ _ _ _ _ _ _ _ _ _ w1231 _ w1271 _ _ _ _ _ _ _ _ _ _ _ _]
      tunnel: w39 -> [w50 _ _ _ _ _ _ _ _ _ _ _ _ _ _ _ _ _ _ _ _ _ _ _ _ _ _ _ _]
      event Timeout {
        # "Read FIFO from Adwin and \nwrite it into File if record \nis activated"
        # "Refresh GUI every 1 s"
        # "Read FIFO/Write File/Refresh GUI"
        n67 = event-data() -> ()  [unwired: 1 in, 3 out]
        n68 = local read "Path Logging"() -> (w49:path)
        n69 = local read "ms Offset"() -> (w62:u32)
        n70 = Tick Count (ms)() -> (millisecond timer value=w61:u32)
        n71 = Format Date/Time String() -> (date/time string=→"Date/Time:":string)  [unwired: 3 in]
        n72 = Subtract(x=w61, y=w62) -> (x-y=w59:u32)
        n73 = call "correlationvi.vi"("Number of Elements"=3, "FifoNo"=i16 40, "Device No."=w50) -> ("Output Array 2"=w51:dbl[][])  [unwired: 6 in, 2 out]
        n74 = Greater?(x=w59, y=u32 1000) -> (0:w60:bool)
        n75 = call "ADwin Get_Par.vi"("index"=u16 45 ("Device No. out"), "Device No. (1)"=w55) -> ("ParameterValue"=w54:i32)  [unwired: 7 in, 2 out]
        "time shift steps" <- w54
        n76 = call "CPT Read_Write_FIFO 12.1.vi"("Device No."=w55, "FifoNo"=w66, "Number of Elements"=w65, "Path Logging"=w49, "Record"="Record Data") -> ("Device No. out"=w63:u16, "Output Array"=w64:dbl[][])  [unwired: 9 in]
        n77 = stacked-sequence {
          tunnel: w64 -> [_ w92 w137 _ _ w346 w533 w586 w626 _ w809 _ _ _]
          tunnel: w63 -> [_ _ _ w279 w293 w360 w531 _ w619 w761 w812 w836 _ w971]
          tunnel: w60 -> [w67 _ _ _ _ _ _ _ _ _ _ _ _ _]
          tunnel: w54 -> [_ _ _ _ _ w375 _ _ w625 _ _ _ _ _]
          tunnel: w51 -> [_ _ _ _ _ w370 w537 _ _ _ _ _ _ _]
          tunnel: w49 -> [_ _ _ _ _ w373 _ _ _ _ _ _ _ _]
          tunnel: "Record Data" -> [_ _ _ _ _ w372 _ _ _ _ _ _ _ _]
          frame #0 {
            # "GUI Disabled & Enabled. Depends which Button can change state and deactivate others"
            n78 = case shown="True" w67 {
              frame False {
              }
              frame True {
                n79 = local read "Penetration ongoing"() -> (w80:bool)
                n80 = local read "Go - Seitendruck"() -> (w76:bool)
                n81 = local read "Go - Porendruck"() -> (w74:bool)
                n82 = local read "Go - Axialdruck"() -> (w75:bool)
                n83 = Tick Count (ms)() -> (millisecond timer value=→"ms Offset":u32)
                n84 = local read "Activate Manuel Control"() -> (w72:bool)
                n85 = case shown="True" w72 {
                  tunnel: [T7."Disabled and Grayed Out" ("Disabled") T7."Enabled" ("Disabled")] -> w83
                  frame False {
                  }
                  frame True {
                  }
                }
                n86 = local read "Move"() -> (w81:bool)
                n87 = Not(x=w72) -> (.not. x?=w70:bool)
                n88 = Compound Arithmetic op=OR(w74, w75, w76) -> (→"Linear Control On":bool)
                n89 = property on="Move" class="Bool (strict)"("DisabledEnum"=w83) -> ()  [unwired: 2 in, 2 out]
                n90 = local read "Activate Pumps/Piston Controls"() -> (w73:bool)
                n91 = Not(x=w73) -> (.not. x?=w71:bool)
                n92 = And(x=w71, y=w70) -> (x .and. y?=w69:bool)
                "Ready" <- w69
                n93 = Compound Arithmetic op=OR(w69, w81, w80) -> (w79:bool)
                n94 = Not(x=w79) -> (.not. x?=→"Hold Position":bool)
                n95 = case shown="False" w73 {
                  tunnel: [T7."Enabled" ("Disabled") T7."Enabled" ("Disabled")] -> w68
                  frame False {
                  }
                  frame True {
                  }
                }
                n96 = property on="Soll Axial Pressure" class="DigNum (strict)"("DisabledEnum"=w68) -> ()  [unwired: 2 in, 2 out]
                n97 = property on="Soll Pore Pressure" class="DigNum (strict)"("DisabledEnum"=w68) -> ()  [unwired: 2 in, 2 out]
                n98 = property on="Regelung Akiv Axial" class="Bool (strict)"("DisabledEnum"=w68) -> ()  [unwired: 2 in, 2 out]
                n99 = property on="Soll Side Pressure" class="DigNum (strict)"("DisabledEnum"=w68) -> ()  [unwired: 2 in, 2 out]
                n100 = property on="Regelung Akiv Sidepressure" class="Bool (strict)"("DisabledEnum"=w68) -> ()  [unwired: 2 in, 2 out]
                n101 = property on="Regelung Akiv Porepress" class="Bool (strict)"("DisabledEnum"=w68) -> ()  [unwired: 2 in, 2 out]
                n102 = property on="SET Pump Offsets" class="Bool"("DisabledEnum"=w68) -> ()  [unwired: 2 in, 2 out]
                n103 = property on="start penetration" class="Bool (strict)"("DisabledEnum"=w68) -> ()  [unwired: 2 in, 2 out]
                n104 = property on="SET Pump Pressures" class="Bool"("DisabledEnum"=w68) -> ()  [unwired: 2 in, 2 out]
                n105 = property on="Go - Porendruck" class="Bool (strict)"("DisabledEnum"=w68) -> ()  [unwired: 2 in, 2 out]
                n106 = property on="Go - Seitendruck" class="Bool (strict)"("DisabledEnum"=w68) -> ()  [unwired: 2 in, 2 out]
                n107 = property on="Go - Axialdruck" class="Bool (strict)"("DisabledEnum"=w68) -> ()  [unwired: 2 in, 2 out]
                n108 = property on="GO All Pressure" class="Bool (strict)"("DisabledEnum"=w68) -> ()  [unwired: 2 in, 2 out]
                n109 = property on="SET Pump Controls" class="Bool"("DisabledEnum"=w68) -> ()  [unwired: 2 in, 2 out]
                n110 = property on="Soll P-Value" class="DigNum (strict)"("DisabledEnum"=w68) -> ()  [unwired: 2 in, 2 out]
                n111 = property on="Delta Pore" class="DigNum (strict)"("DisabledEnum"=w68) -> ()  [unwired: 2 in, 2 out]
                n112 = property on="Soll I-Value" class="DigNum (strict)"("DisabledEnum"=w68) -> ()  [unwired: 2 in, 2 out]
                n113 = property on="Delta Seiten" class="DigNum (strict)"("DisabledEnum"=w68) -> ()  [unwired: 2 in, 2 out]
                n114 = property on="Velocity Linear" class="DigNum (strict)"("DisabledEnum"=w68) -> ()  [unwired: 2 in, 2 out]
                n115 = property on="Delta Axial" class="DigNum (strict)"("DisabledEnum"=w68) -> ()  [unwired: 2 in, 2 out]
                n116 = property on="Up_Lower" class="Bool (strict)"("DisabledEnum"=w68) -> ()  [unwired: 2 in, 2 out]
                n117 = property on="Vorschub SOLL" class="DigNum (strict)"("DisabledEnum"=w68) -> ()  [unwired: 2 in, 2 out]
                n118 = property on="VibroTest" class="Bool (strict)"("DisabledEnum"=w68) -> ()  [unwired: 2 in, 2 out]
                n119 = property on="Frequency SOLL" class="DigNum (strict)"("DisabledEnum"=w68) -> ()  [unwired: 2 in, 2 out]
                n120 = property on="SET Vibro Settings" class="Bool"("DisabledEnum"=w68) -> ()  [unwired: 2 in, 2 out]
                n121 = property on="SET P/I Value" class="Bool"("DisabledEnum"=w68) -> ()  [unwired: 2 in, 2 out]
                n122 = property on="Amplitude SOLL" class="DigNum (strict)"("DisabledEnum"=w68) -> ()  [unwired: 2 in, 2 out]
              }
            }
          }
          frame #1 {
            # "Displaying FIFO Charts. Just for Debugging of the Control Part"
            n123 = property on="Control start" class="Bool (strict)"() -> ("Value"=w90:bool)  [unwired: 2 in, 2 out]
            n124 = local read "start penetration"() -> (w89:bool)
            n125 = Or(x=w89, y=w90) -> (x .or. y?=w88:bool)
            n126 = case shown="True" w88 {
              frame False {
              }
              frame True {
                n127 = local read "Cone Tip Resistance"() -> (w95:dbl)
                n128 = local read "reset_flag"() -> (w94:bool)
                n129 = local read "Position Piston"() -> (w96:dbl)
                n130 = case shown="True" w94 {
                  tunnel: [FALSE ("Reset") TRUE ("Reset")] -> w93
                  frame False {
                  }
                  frame True {
                    n131 = local write "reset_flag"(FALSE ("reset_flag")) -> ()
                  }
                }
                n132 = call "XY-Graph erzeugen3"("Reset"=w93, "Y Input"=w96, "X Input"=w95) -> ("XY Graph"=→"Interner Kraftsensor [MPa]":cluster{"Y":dbl[], "Y":dbl[]}[])  [unwired: 7 in, 1 out]
              }
            }
            n133 = case shown="True" "Stop/Start" {
              tunnel: w92 -> [_ w106]
              frame False {
              }
              frame True {
                n134 = Index Array(array=w106, index (row)=T8."Stellwert Regler" ("Enum")) -> (element=w101:dbl[])  [unwired: 1 in]
                n135 = Index Array(array=w106, index (row)=T8."Position Induktiv" ("Enum")) -> (element=w109:dbl[])  [unwired: 1 in]
                n136 = Index Array(array=w106, index (row)=T8."Valve Kolbenposition" ("Enum")) -> (element=w107:dbl[])  [unwired: 1 in]
                n137 = Index Array(array=w106, index (row)=T8."Regelanweichung" ("Enum")) -> (element=w108:dbl[])  [unwired: 1 in]
                n138 = for {
                  tunnel: w101 -> [w110] mode=indexing
                  "Regelung Out" <- w110
                }
                n139 = for {
                  tunnel: w109 -> [w115] mode=indexing
                  tunnel: w108 -> [w112] mode=indexing
                  n140 = expression code="(x-623)*(-(33076/410))"(w115) -> (w114:dbl)
                  n141 = Subtract(x=w114, y=w112) -> (x-y=w113:dbl)
                  n142 = Bundle(w114, w113) -> (→"SOLL IS Distance":cluster{dbl, dbl})  [unwired: 1 in]
                }
                n143 = for {
                  tunnel: w107 -> [w111] mode=indexing
                  "Valve Is" <- w111
                }
              }
            }
          }
          frame #2 {
            # "For detecting leackage. \nAnd Showing the loss per minute"
            # "Displaying FIFO GUI. Refreshes the Values from the GUI. Since there are a lot of data. It just takes the average value of the array"
            n144 = Index Array(array=w137, index (row)=T8."Force " ("Enum")) -> (element=w179:dbl[])  [unwired: 1 in]
            n145 = Index Array(array=w137, index (row)=T8."Position Induktiv" ("Enum")) -> (element=w180:dbl[])  [unwired: 1 in]
            n146 = Index Array(array=w137, index (row)=T8."LVDT 1" ("Enum")) -> (element=w185:dbl[])  [unwired: 1 in]
            n147 = Index Array(array=w137, index (row)=T8."LVDT 2" ("Enum")) -> (element=w186:dbl[])  [unwired: 1 in]
            n148 = Index Array(array=w137, index (row)=T8."LVDT 3" ("Enum")) -> (element=w187:dbl[])  [unwired: 1 in]
            n149 = Index Array(array=w137, index (row)=T8."Pore Pressure" ("Enum")) -> (element=w170:dbl[])  [unwired: 1 in]
            n150 = Index Array(array=w137, index (row)=T8."Side Pressure " ("Enum")) -> (element=w171:dbl[])  [unwired: 1 in]
            n151 = Index Array(array=w137, index (row)=T8."Axial Pressure" ("Enum")) -> (element=w172:dbl[])  [unwired: 1 in]
            n152 = To Double Precision Float(number=w187) -> (double precision float=w184:dbl[])
            n153 = To Double Precision Float(number=w172) -> (double precision float=w169:dbl[])
            n154 = To Double Precision Float(number=w186) -> (double precision float=w182:dbl[])
            n155 = To Double Precision Float(number=w180) -> (double precision float=w175:dbl[])
            n156 = To Double Precision Float(number=w185) -> (double precision float=w183:dbl[])
            n157 = To Double Precision Float(number=w179) -> (double precision float=w176:dbl[])
            n158 = To Double Precision Float(number=w170) -> (double precision float=w168:dbl[])
            n159 = To Double Precision Float(number=w171) -> (double precision float=w167:dbl[])
            n160 = call-poly <vilib>:"Mean.vi"("X"=w183) -> ("mean"=w188:dbl)  [unwired: 1 out]
            "LVDT 1" <- w188
            n161 = call-poly <vilib>:"Mean.vi"("X"=w182) -> ("mean"=w151:dbl)  [unwired: 1 out]
            "LVDT 2" <- w151
            n162 = call-poly <vilib>:"Mean.vi"("X"=w184) -> ("mean"=w150:dbl)  [unwired: 1 out]
            "LVDT 3" <- w150
            n163 = call-poly <vilib>:"Mean.vi"("X"=w176) -> ("mean"=w177:dbl)  [unwired: 1 out]
            "Force Sensor" <- w177
            n164 = call-poly <vilib>:"Mean.vi"("X"=w175) -> ("mean"=→"Position Piston":dbl)  [unwired: 1 out]
            n165 = call-poly <vilib>:"Mean.vi"("X"=w168) -> ("mean"=→"Pore Pressure [KPa]" →"Porendruck [Pa] 2":dbl)  [unwired: 1 out]
            n166 = call-poly <vilib>:"Mean.vi"("X"=w167) -> ("mean"=→"Side Pressure  [KPa]" →"Seitendruck [Pa] 3":dbl)  [unwired: 1 out]
            n167 = call-poly <vilib>:"Mean.vi"("X"=w169) -> ("mean"=→"Axial Pressure  [KPa]" →"Axialdruck [Pa] 4":dbl)  [unwired: 1 out]
            n168 = Bundle("mean"=w188, "mean"=w151, "mean"=w150) -> (→"LVDT Frontpannel":cluster{"mean":dbl, "mean":dbl, "mean":dbl})  [unwired: 1 in]
            n169 = Greater?(x=w177, y=-197.0) -> (0:→"Contact?":bool)
            n170 = Index Array(array=w137, index (row)=T8."Pore Volumen" ("Enum")) -> (element=w156:dbl[])  [unwired: 1 in]
            n171 = Index Array(array=w137, index (row)=T8."Side Volumen " ("Enum")) -> (element=w157:dbl[])  [unwired: 1 in]
            n172 = Index Array(array=w137, index (row)=T8."Axial Volumen " ("Enum")) -> (element=w158:dbl[])  [unwired: 1 in]
            n173 = To Double Precision Float(number=w156) -> (double precision float=w153:dbl[])
            n174 = To Double Precision Float(number=w157) -> (double precision float=w154:dbl[])
            n175 = To Double Precision Float(number=w158) -> (double precision float=w155:dbl[])
            n176 = Index Array(array=w137, index (row)=18) -> (element=w161:dbl[])  [unwired: 1 in]
            n177 = Index Array(array=w137, index (row)=T9."additional side pressure" ("Enum")) -> (element=w162:dbl[])  [unwired: 1 in]
            n178 = Index Array(array=w137, index (row)=T9."Tip resistance" ("Enum")) -> (element=w165:dbl[])  [unwired: 1 in]
            n179 = Index Array(array=w137, index (row)=T9."Pore pressure" ("Enum")) -> (element=w166:dbl[])  [unwired: 1 in]
            n180 = To Double Precision Float(number=w161) -> (double precision float=w159:dbl[])
            n181 = To Double Precision Float(number=w162) -> (double precision float=w160:dbl[])
            n182 = To Double Precision Float(number=w165) -> (double precision float=w120:dbl[])
            n183 = To Double Precision Float(number=w166) -> (double precision float=w119:dbl[])
            n184 = call-poly <vilib>:"Mean.vi"("X"=w153) -> ("mean"=w133:dbl)  [unwired: 1 out]
            "ml Pore Linear" <- w133
            "Pore" <- w133
            n185 = call-poly <vilib>:"Mean.vi"("X"=w154) -> ("mean"=w132:dbl)  [unwired: 1 out]
            "ml Side Linear" <- w132
            "Side" <- w132
            n186 = call-poly <vilib>:"Mean.vi"("X"=w155) -> ("mean"=w131:dbl)  [unwired: 1 out]
            "ml Axial Linear" <- w131
            "Axial" <- w131
            n187 = call-poly <vilib>:"Mean.vi"("X"=w159) -> ("mean"=→"Max Expansion":dbl)  [unwired: 1 out]
            n188 = call-poly <vilib>:"Mean.vi"("X"=w160) -> ("mean"=→"Addional Side Pressure":dbl)  [unwired: 1 out]
            n189 = Index Array(array=w120, index=0) -> (element=w117:dbl)
            "Cone Tip Resistance" <- w117
            n190 = call-poly <vilib>:"Mean.vi"("X"=w119) -> ("mean"=w118:dbl)  [unwired: 1 out]
            "Pore Pressure" <- w118
            n191 = Bundle("mean"=w133, "mean"=w132, "mean"=w131) -> (→"ml Fontpanel":cluster{"mean":dbl, "mean":dbl, "mean":dbl})  [unwired: 1 in]
            n192 = Bundle(w117, "mean"=w118) -> (→"Cone Pressure":cluster{dbl, "mean":dbl})  [unwired: 1 in]
            n193 = call "CPT Delta_leakage_mlpm 12.1.vi"("IN Pore"=w133, "IN Side"=w132, "IN Axial"=w131, "Reset"="Reset Leackage") -> ("Time Out"=→"Timer Leackage":dbl, "OUT Pore Leakage"=→"Pore Leackage":dbl, "OUT Side Leakage"=→"Side Leackage":dbl, "OUT Axial Leakage"=→"Axial Leackage":dbl)  [unwired: 12 in]
          }
          frame #3 {
            w203 = u16 80 items=["NaN", "Kp_Position_Vibro", "Ki_Position_Vibro", "PAR_3", "Sinusfrequenz_preSh", "Zylinder_Move_Button", "PAR_6", "PAR_7", "PAR_8", "PAR_9", "PAR_10", "PAR_11", "PAR_12", "Amplitude_PreSh", "Compass_OFF", "PAR_15", "PAR_16", "SollMoog", "PAR_18", "PAR_19", "PAR_20", "Vibro_Test_Button", "PAR_22", "PAR_23", "PAR_24", "PAR_25", "PAR_26", "PAR_27", "PAR_28", "PAR_29", "PAR_30", "PAR_31", "PAR_32", "Start_Test_Button", "PAR_34", "Programm_counter", "PAR_36", "Circumference_ON_Flag", "PAR_38", "PAR_39", "Pore_Control_Button", "Side_Control_Button", "Axial_Control_Button", "PAR_43", "PAR_44", "PAR_45", "Einfahren_Piston", "PAR_47", "PAR_48", "PAR_49", "PAR_50", "PAR_51", "PAR_52", "PAR_53", "PAR_54", "PAR_55", "PAR_56", "PAR_57", "LinearUpDown_Button", "Linear_Pore_GO", "Linear_Axial_GO", "Linear_Side_GO", "PAR_62", "PAR_63", "PAR_64", "PAR_65", "PAR_66", "PAR_67", "PAR_68", "PAR_69", "Pre_Shearing_Button", "PAR_71", "PAR_72", "PAR_73", "PAR_74", "Circumf_Control_On", "PAR_76", "PAR_77", "PAR_78", "PAR_79", "Modus", "", "", "", "", "", "", "", "", "", "", "", "", "", "", "", "", "", "", "", "", "", "", "", "", "", ""] ("par_enum")
            w204 = u16 21 items=["NaN", "Kp_Position_Vibro", "Ki_Position_Vibro", "PAR_3", "Sinusfrequenz_preSh", "Zylinder_Move_Button", "PAR_6", "PAR_7", "PAR_8", "PAR_9", "PAR_10", "PAR_11", "PAR_12", "Amplitude_PreSh", "Compass_OFF", "PAR_15", "PAR_16", "SollMoog", "PAR_18", "PAR_19", "PAR_20", "Vibro_Test_Button", "PAR_22", "PAR_23", "PAR_24", "PAR_25", "PAR_26", "PAR_27", "PAR_28", "PAR_29", "PAR_30", "PAR_31", "PAR_32", "Start_Test_Button", "PAR_34", "Programm_counter", "PAR_36", "Circumference_ON_Flag", "PAR_38", "PAR_39", "Pore_Control_Button", "Side_Control_Button", "Axial_Control_Button", "PAR_43", "PAR_44", "PAR_45", "Einfahren_Piston", "PAR_47", "PAR_48", "PAR_49", "PAR_50", "PAR_51", "PAR_52", "PAR_53", "PAR_54", "PAR_55", "PAR_56", "PAR_57", "LinearUpDown_Button", "Linear_Pore_GO", "Linear_Axial_GO", "Linear_Side_GO", "PAR_62", "PAR_63", "PAR_64", "PAR_65", "PAR_66", "PAR_67", "PAR_68", "PAR_69", "Pre_Shearing_Button", "PAR_71", "PAR_72", "PAR_73", "PAR_74", "Circumf_Control_On", "PAR_76", "PAR_77", "PAR_78", "PAR_79", "Modus", "", "", "", "", "", "", "", "", "", "", "", "", "", "", "", "", "", "", "", "", "", "", "", "", "", ""] ("par_enum")
            w202 = u16 2 items=["NaN", "Kp_Position_Vibro", "Ki_Position_Vibro", "PAR_3", "Sinusfrequenz_preSh", "Zylinder_Move_Button", "PAR_6", "PAR_7", "PAR_8", "PAR_9", "PAR_10", "PAR_11", "PAR_12", "Amplitude_PreSh", "Compass_OFF", "PAR_15", "PAR_16", "SollMoog", "PAR_18", "PAR_19", "PAR_20", "Vibro_Test_Button", "PAR_22", "PAR_23", "PAR_24", "PAR_25", "PAR_26", "PAR_27", "PAR_28", "PAR_29", "PAR_30", "PAR_31", "PAR_32", "Start_Test_Button", "PAR_34", "Programm_counter", "PAR_36", "Circumference_ON_Flag", "PAR_38", "PAR_39", "Pore_Control_Button", "Side_Control_Button", "Axial_Control_Button", "PAR_43", "PAR_44", "PAR_45", "Einfahren_Piston", "PAR_47", "PAR_48", "PAR_49", "PAR_50", "PAR_51", "PAR_52", "PAR_53", "PAR_54", "PAR_55", "PAR_56", "PAR_57", "LinearUpDown_Button", "Linear_Pore_GO", "Linear_Axial_GO", "Linear_Side_GO", "PAR_62", "PAR_63", "PAR_64", "PAR_65", "PAR_66", "PAR_67", "PAR_68", "PAR_69", "Pre_Shearing_Button", "PAR_71", "PAR_72", "PAR_73", "PAR_74", "Circumf_Control_On", "PAR_76", "PAR_77", "PAR_78", "PAR_79", "Modus", "", "", "", "", "", "", "", "", "", "", "", "", "", "", "", "", "", "", "", "", "", "", "", "", "", ""] ("par_enum")
            w201 = u16 1 items=["NaN", "Kp_Position_Vibro", "Ki_Position_Vibro", "PAR_3", "Sinusfrequenz_preSh", "Zylinder_Move_Button", "PAR_6", "PAR_7", "PAR_8", "PAR_9", "PAR_10", "PAR_11", "PAR_12", "Amplitude_PreSh", "Compass_OFF", "PAR_15", "PAR_16", "SollMoog", "PAR_18", "PAR_19", "PAR_20", "Vibro_Test_Button", "PAR_22", "PAR_23", "PAR_24", "PAR_25", "PAR_26", "PAR_27", "PAR_28", "PAR_29", "PAR_30", "PAR_31", "PAR_32", "Start_Test_Button", "PAR_34", "Programm_counter", "PAR_36", "Circumference_ON_Flag", "PAR_38", "PAR_39", "Pore_Control_Button", "Side_Control_Button", "Axial_Control_Button", "PAR_43", "PAR_44", "PAR_45", "Einfahren_Piston", "PAR_47", "PAR_48", "PAR_49", "PAR_50", "PAR_51", "PAR_52", "PAR_53", "PAR_54", "PAR_55", "PAR_56", "PAR_57", "LinearUpDown_Button", "Linear_Pore_GO", "Linear_Axial_GO", "Linear_Side_GO", "PAR_62", "PAR_63", "PAR_64", "PAR_65", "PAR_66", "PAR_67", "PAR_68", "PAR_69", "Pre_Shearing_Button", "PAR_71", "PAR_72", "PAR_73", "PAR_74", "Circumf_Control_On", "PAR_76", "PAR_77", "PAR_78", "PAR_79", "Modus", "", "", "", "", "", "", "", "", "", "", "", "", "", "", "", "", "", "", "", "", "", "", "", "", "", ""] ("par_enum")
            # "Par & Fpar auslesen von ADwin. For Communicating with Adwin. Reading a Block of fpar and par and refreshing the value wit it in the GUI"
            n194 = call "ADwin Get_FPar_Block.vi"("count"=i16 80, "startindex"=i16 1, "Device No."=w279) -> ("Data"=w189:sgl[], "Device No. out"=w270:u16)  [unwired: 2 in, 2 out]
            n195 = Decrement(x=T11."PorePressOffset" ("Enum")) -> (x-1=w276:T11)
            n196 = Decrement(x=T11."AxialPressOffset" ("Enum")) -> (x-1=w275:T11)
            n197 = Decrement(x=T11."SidePressOffset" ("Enum")) -> (x-1=w274:T11)
            n198 = Decrement(x=T10."Slope_calibration" ("Enum")) -> (x-1=w194:T10)
            n199 = Decrement(x=T11."Amplitude_Vibro" ("Enum")) -> (x-1=w271:T11)
            n200 = Decrement(x=T11."PreShearingOutput" ("Enum")) -> (x-1=w232:T11)
            n201 = Decrement(x=T11."Ki_Sidepress" ("Enum")) -> (x-1=w264:T11)
            n202 = Decrement(x=T11."Kp_Axialpress" ("Enum")) -> (x-1=w263:T11)
            n203 = Decrement(x=T11."Vorschub" ("Enum")) -> (x-1=w273:T11)
            n204 = Decrement(x=T11."Kp_Porepress" ("Enum")) -> (x-1=w267:T11)
            n205 = Decrement(x=T11."Ki_Porepress" ("Enum")) -> (x-1=w266:T11)
            n206 = Decrement(x=T11."Kp_Sidepress" ("Enum")) -> (x-1=w265:T11)
            n207 = Decrement(x=T10."Intercept_calibration" ("Enum")) -> (x-1=w191:T10)
            n208 = Decrement(x=T11."Ki_Axialpress" ("Enum")) -> (x-1=w262:T11)
            n209 = Decrement(x=T11."Sinusfrequenz_Vibro" ("Enum")) -> (x-1=w272:T11)
            n210 = Index Array(array=w189, index=w276) -> ()  [unwired: 1 out]
            n211 = Index Array(array=w189, index=w275) -> ()  [unwired: 1 out]
            n212 = Index Array(array=w189, index=w274) -> ()  [unwired: 1 out]
            n213 = Index Array(array=w189, index=w272) -> (element=w269:sgl)
            n214 = Index Array(array=w189, index=w271) -> (element=w268:sgl)
            n215 = Index Array(array=w189, index=w232) -> (element=w231:sgl)
            n216 = Index Array(array=w189, index=w264) -> (element=→"Side Ki:":sgl)
            n217 = Index Array(array=w189, index=w263) -> (element=→"Axial Kp:":sgl)
            n218 = Index Array(array=w189, index=w273) -> (element=w200:sgl)
            n219 = Index Array(array=w189, index=w267) -> (element=→"Pore Kp:":sgl)
            n220 = Index Array(array=w189, index=w266) -> (element=→"Pore Ki:":sgl)
            n221 = Index Array(array=w189, index=w265) -> (element=→"Side Kp:":sgl)
            n222 = Index Array(array=w189, index=w262) -> (element=→"Axial Ki:":sgl)
            n223 = Index Array(array=w189, index=w194) -> (element=→"IS-ADWIN":sgl)
            n224 = Index Array(array=w189, index=w191) -> (element=→"IS- ADWIN":sgl)
            n225 = expression code="12000/65536*x-6000"(w231) -> (→"Pre-shearing output":sgl)
            n226 = expression code="1/x"(w269) -> (→"Frequency IS":sgl)
            n227 = expression code="x/78"(w268) -> (→"Amplitude IS":sgl)
            n228 = Multiply(x=w200, y=sgl 5000.0) -> (x*y=w197:sgl)
            n229 = Divide(x=w197, y=sgl 78.01) -> (x/y=→"Feeding IS":sgl)
            n230 = call "ADwin Get_Par_Block.vi"("count"=i16 80, "startindex"=i16 1, "Device No."=w270) -> ("Data"=w282:i32[])  [unwired: 1 in, 3 out]
            n231 = Decrement(x=w201) -> (x-1=w286:u16)
            n232 = Decrement(x=w202) -> (x-1=w285:u16)
            n233 = Decrement(x=w204) -> (x-1=w284:u16)
            n234 = Decrement(x=w203) -> (x-1=w283:u16)
            n235 = Index Array(array=w282, index=w286) -> (element=→"IS P-Value":i32)
            n236 = Index Array(array=w282, index=w285) -> (element=→"IS I-Value":i32)
            n237 = Index Array(array=w282, index=w284) -> (element=w281:i32)
            n238 = Index Array(array=w282, index=w283) -> (element=→"Modus":i32)
            n239 = Decrement(x=T11."Huang_Su_par_4" ("Enum")) -> (x-1=w252:T11)
            n240 = Decrement(x=T11."Huang_Su_par_5" ("Enum")) -> (x-1=w251:T11)
            n241 = Decrement(x=T11."Huang_Su_par_1" ("Enum")) -> (x-1=w255:T11)
            n242 = Decrement(x=T11."Huang_Su_par_2" ("Enum")) -> (x-1=w254:T11)
            n243 = Decrement(x=T11."Huang_Su_par_3" ("Enum")) -> (x-1=w253:T11)
            n244 = Decrement(x=T11."Set_Soll_AxialPressure" ("Enum")) -> (x-1=w247:T11)
            n245 = Decrement(x=T11."Huang_Su_par_6" ("Enum")) -> (x-1=w250:T11)
            n246 = Decrement(x=T11."Huang_Su_par_7" ("Enum")) -> (x-1=w249:T11)
            n247 = Decrement(x=T11."Set_Soll_PorePressure" ("Enum")) -> (x-1=w248:T11)
            n248 = Decrement(x=T11."Set_Soll_SidePressure" ("Enum")) -> (x-1=w246:T11)
            n249 = Equal?(x=w281, y=1) -> (x = y?=→"Vibro Test IS":bool)
            n250 = Index Array(array=w189, index=w247) -> (element=w241:sgl)
            n251 = Index Array(array=w189, index=w246) -> (element=w240:sgl)
            n252 = Index Array(array=w189, index=w255) -> (element=→"IS Parameter 1":sgl)
            n253 = Index Array(array=w189, index=w254) -> (element=→"IS Parameter 2":sgl)
            n254 = Index Array(array=w189, index=w253) -> (element=→"IS Parameter 3":sgl)
            n255 = Index Array(array=w189, index=w252) -> (element=→"IS Parameter 4":sgl)
            n256 = Index Array(array=w189, index=w251) -> (element=→"IS Parameter 5":sgl)
            n257 = Index Array(array=w189, index=w250) -> (element=→"IS Parameter 6":sgl)
            n258 = Index Array(array=w189, index=w249) -> (element=→"IS Parameter 7":sgl)
            n259 = Index Array(array=w189, index=w248) -> (element=w242:sgl)
            n260 = expression code="12000/65536*(x-32768)"(w242) -> (→"Porepressure":sgl)
            n261 = expression code="12000/65536*(x-32768)"(w241) -> (→"Axialpressure":sgl)
            n262 = expression code="12000/65536*(x-32768)"(w240) -> (→"Sidepressure":sgl)
          }
          frame #4 {
            (unwired) "Modification done by zhengyu chen, if measured side, pore and axial pressure is less than default\nvalues, we force them to be default values. "
            # "Set pump offset for pore, side and axial pressure sensor"
            n263 = case shown="True" "Set" {
              tunnel: w293 -> [_ w295]
              frame False {
              }
              frame True {
                n264 = call "ADwin Get_FPar_Block.vi"("count"=i16 80, "startindex"=i16 1, "Device No."=w295) -> ("Data"=w317:sgl[])  [unwired: 2 in, 3 out]
                n265 = Decrement(x=T11."SidePressOffset" ("Enum")) -> (x-1=w320:T11)
                n266 = Decrement(x=T11."AxialPressOffset" ("Enum")) -> (x-1=w319:T11)
                n267 = Decrement(x=T11."PorePressOffset" ("Enum")) -> (x-1=w318:T11)
                n268 = Index Array(array=w317, index=w320) -> (element=w313:sgl)
                n269 = Greater?(x=w313, y="Side Offset Soll 2") -> (0:w324:bool)
                n270 = Index Array(array=w317, index=w319) -> (element=w305:sgl)
                n271 = Greater?(x=w305, y="Axial Offset Soll 2") -> (0:w310:bool)
                n272 = Index Array(array=w317, index=w318) -> (element=w302:sgl)
                n273 = Greater?(x=w302, y="Pore Offset SOLL 2") -> (0:w303:bool)
                n274 = case shown="True" w310 {
                  tunnel: w295 -> [w333 w337]
                  tunnel: [w333 w337] -> w308
                  tunnel: "Axial Offset Soll 2" -> [w334 w335]
                  tunnel: [w334 w335] -> w306
                  tunnel: T11."AxialPressOffset" ("Enum") -> [w332 w336]
                  tunnel: [w332 w336] -> w307
                  tunnel: w305 -> [_ _]
                  frame False {
                  }
                  frame True {
                  }
                }
                n275 = case shown="False" w324 {
                  tunnel: w295 -> [w339 w343]
                  tunnel: [w339 w343] -> w325
                  tunnel: "Side Offset Soll 2" -> [w340 w341]
                  tunnel: [w340 w341] -> w311
                  tunnel: T11."SidePressOffset" ("Enum") -> [w338 w342]
                  tunnel: [w338 w342] -> w312
                  tunnel: w313 -> [_ _]
                  frame False {
                  }
                  frame True {
                  }
                }
                n276 = case shown="True" w303 {
                  tunnel: w295 -> [w327 w331]
                  tunnel: [w327 w331] -> w301
                  tunnel: "Pore Offset SOLL 2" -> [w328 w329]
                  tunnel: [w328 w329] -> w299
                  tunnel: T11."PorePressOffset" ("Enum") -> [w326 w330]
                  tunnel: [w326 w330] -> w300
                  tunnel: w302 -> [_ _]
                  frame False {
                  }
                  frame True {
                  }
                }
                n277 = call "ADwin Set_FPar.vi"("Value"=w311, "Index"=w312, "Device No."=w325) -> ()  [unwired: 6 in, 3 out]
                n278 = call "ADwin Set_FPar.vi"("Value"=w306, "Index"=w307, "Device No."=w308) -> ()  [unwired: 6 in, 3 out]
                n279 = call "ADwin Set_FPar.vi"("Value"=w299, "Index"=w300, "Device No."=w301) -> ()  [unwired: 6 in, 3 out]
                "Pore Offset: 2" <- "Pore Offset SOLL 2"
                "Axial Offset: 2" <- "Axial Offset Soll 2"
                "Side Offset: 2" <- "Side Offset Soll 2"
              }
            }
          }
          frame #5 {
            (unwired) FALSE
            (unwired) "depth for 3rd vibro mode"
            (unwired) "depth for 2nd vibro mode"
            (unwired) "depth for 1st vibro mode"
            # "Visualize velocity data, filtered velocity, linear regression plots for model/based controller"
            n280 = call "ADwin Get_Par.vi"("index"=i16 76, "Device No. (1)"=w360) -> ("ParameterValue"=w377:i32)  [unwired: 7 in, 2 out]
            n281 = Subtract(x=w375, y=0) -> (x-y=w344:i32)
            n282 = Array Subset(array=w346, index (row)=0 ("index"), length (row)=w377) -> (w376:dbl[][])  [unwired: 2 in]
            n283 = call "ADwin Get_FPar.vi"("Index"=u16 23, "Device No. (1)"=w360) -> ()  [unwired: 7 in, 3 out]
            n284 = call "ADwin Get_FPar.vi"("Index"=u16 24, "Device No. (1)"=w360) -> ("ParameterValue"=w368:sgl)  [unwired: 7 in, 2 out]
            n285 = call "ADwin Get_FPar_Block.vi"("count"=i16 80, "startindex"=i16 1, "Device No."=w360) -> ("Data"=w383:sgl[])  [unwired: 2 in, 3 out]
            n286 = case shown="True" "Visualize data" {
              tunnel: w383 -> [_ w514]
              tunnel: w376 -> [_ _]
              tunnel: w344 -> [_ w483]
              tunnel: w344 -> [_ _]
              tunnel: w373 -> [w430 w461]
              tunnel: w372 -> [w429 w460]
              tunnel: w370 -> [_ w479]
              tunnel: w368 -> [_ w466]
              tunnel: [w427 w448] -> w355
              tunnel: [w430 w461] -> w348
              tunnel: [w429 w460] -> w347
              tunnel: [w427 w448] -> w357
              tunnel: w346 -> [w428 w442]
              frame False {
                n287 = Delete From Array(array=w428, length=2, index (row)=19) -> (array with subset deleted=w427:dbl[][])  [unwired: 1 in, 1 out]
              }
              frame True {
                (unwired) "up to down:\n\n      1. desired  distance\n      2. predicted distance\n      3. measured distance\n      4. shifted predicted distance\n        \n"
                (unwired) " Estimated controller output"
                (unwired) " predict distance"
                (unwired) "Desired distance"
                (unwired) "fitted velocity data from linear regression"
                (unwired) "controller output"
                (unwired) "distance sensor measurement"
                (unwired) "velocity data"
                (unwired) "fitted intercept from linear regression, parameter b"
                (unwired) "fitted slope from linear regression, parameter m"
                # "Writing File"
                # "Model controller performance visualization"
                n288 = Index Array(array=w479, index (row)=2) -> (element=w463:dbl[])  [unwired: 1 in]
                n289 = Index Array(array=w442, index (row)=T9."Position Induktiv" ("Enum")) -> (element=w484:dbl[])  [unwired: 1 in]
                n290 = Index Array(array=w442, index (row)=T9."predict distance" ("Enum")) -> (element=w477:dbl[])  [unwired: 1 in]
                n291 = Index Array(array=w442, index (row)=T9."desired distance" ("Enum")) -> (element=w474:dbl[])  [unwired: 1 in]
                n292 = Index Array(array=w442, index (row)=T9."fitted velocity" ("Enum")) -> (element=w435:dbl[])  [unwired: 1 in]
                n293 = Index Array(array=w442, index (row)=T9."Distance_Regout" ("Enum")) -> (element=w476:dbl[])  [unwired: 1 in]
                n294 = Split 1D Array(array=w435, index=w483) -> (second subarray=w434:dbl[])  [unwired: 1 out]
                n295 = Index Array(array=w442, index (row)=T9."velocity data" ("Enum")) -> (element=w454:dbl[])  [unwired: 1 in]
                n296 = Index Array(array=w514, index=T11."FPAR_33" ("Enum")) -> (element=→"Slope m":sgl)
                n297 = Multiply(x=2, y=w483) -> (x*y=w485:i32)
                n298 = Split 1D Array(array=w477, index=w485) -> (second subarray=w487:dbl[])  [unwired: 1 out]
                n299 = Split 1D Array(array=w484, index=w485) -> (second subarray=w455:dbl[])  [unwired: 1 out]
                n300 = Index Array(array=w514, index=T11."FPAR_34" ("Enum")) -> (element=→"Intercept b":sgl)
                n301 = Split 1D Array(array=w476, index=0) -> (second subarray=w453:dbl[])  [unwired: 1 out]
                n302 = Less?(x=w466, y=sgl 0.0) -> (x < y?=w465:bool)
                n303 = Split 1D Array(array=w453, index=w483) -> (second subarray=w437:dbl[])  [unwired: 1 out]
                n304 = Split 1D Array(array=w487, index=w483) -> (second subarray=w468:dbl[])  [unwired: 1 out]
                n305 = Index Array(array=w442, index (row)=T9."Distance_Regout" ("Enum")) -> (element=w447:dbl[])  [unwired: 1 in]
                n306 = Index Array(array=w442, index (row)=T9."estimated_Distance_Regout" ("Enum")) -> (element=w510:dbl[])  [unwired: 1 in]
                n307 = Bundle(w453, "Output Array"=w454) -> (w451:cluster{dbl[], "Output Array":dbl[]})  [unwired: 1 in]
                n308 = Bundle(w437, "Output Array"=w454) -> (w452:cluster{dbl[], "Output Array":dbl[]})  [unwired: 1 in]
                n309 = Bundle(w437, w434) -> (w436:cluster{dbl[], dbl[]})  [unwired: 1 in]
                n310 = Split 1D Array(array=w487, index=0) -> (second subarray=w482:dbl[])  [unwired: 1 out]
                n311 = Split 1D Array(array=w474, index=w483) -> (second subarray=w438:dbl[])  [unwired: 1 out]
                n312 = Build Array(w452, w451, w436) -> (→"Linear regression":cluster{dbl[], "Output Array":dbl[]}[])
                n313 = Index Array(array=w442, index (row)=0) -> (element=w473:dbl[])  [unwired: 1 in]
                n314 = Index Array(array=w442, index (row)=T9."Distance_Regout" ("Enum")) -> (element=w489:dbl[])  [unwired: 1 in]
                n315 = Index Array(array=w442, index (row)=T9."velocity data" ("Enum")) -> (element=w457:dbl[])  [unwired: 1 in]
                n316 = Split 1D Array(array=w489, index=0) -> (second subarray=w459:dbl[])  [unwired: 1 out]
                n317 = Subtract(x=w438, y=w455) -> (x-y=w464:dbl[])
                n318 = case shown="False" w465 {
                  tunnel: w464 -> [w524 w530]
                  tunnel: [w520 w527] -> w433
                  tunnel: w463 -> [_ w528]
                  frame False {
                    n319 = Multiply(x=w524, y=1.0) -> (x*y=w522:dbl[])
                    n320 = Divide(x=w522, y=1.0) -> (x/y=w523:dbl[])
                    n321 = Sort 1D Array(array=w523) -> (sorted array=w521:dbl[])
                    n322 = Reverse 1D Array(array=w521) -> (reversed array=w520:dbl[])
                  }
                  frame True {
                    n323 = call-poly <vilib>:"Mean.vi"("X"=w530) -> ("mean"=w529:dbl)  [unwired: 1 out]
                    n324 = Multiply(x=w529, y=w528) -> (x*y=w527:dbl[])
                  }
                }
                n325 = Subtract(x=w474, y=w433) -> (x-y=w446:dbl[])
                n326 = call <vilib>:"Normalize Waveform.vi"("waveform in"=w457) -> ("normalized waveform"=w456:waveform(dbl))  [unwired: 7 in, 3 out]
                n327 = Subtract(x=w468, y=w455) -> ()  [unwired: 1 out]
                n328 = call <vilib>:"Normalize Waveform.vi"("waveform in"=w459) -> ("normalized waveform"=w458:waveform(dbl))  [unwired: 7 in, 3 out]
                n329 = Bundle("Output Array"=w473, "Output Array"=w510) -> (w509:T13)  [unwired: 1 in]
                n330 = Bundle("Output Array"=w473, "Output Array"=w447) -> (w508:T13)  [unwired: 1 in]
                n331 = Bundle("Output Array"=w473, w455) -> (w504:cluster{"Output Array":dbl[], dbl[]})  [unwired: 1 in]
                n332 = Bundle("Output Array"=w473, w482) -> (w505:cluster{"Output Array":dbl[], dbl[]})  [unwired: 1 in]
                n333 = Bundle("Output Array"=w473, "normalized waveform"=w456) -> (w512:T14)  [unwired: 1 in]
                n334 = Bundle("Output Array"=w473, w446) -> (w506:cluster{"Output Array":dbl[], dbl[]})  [unwired: 1 in]
                n335 = Bundle("Output Array"=w473, "normalized waveform"=w458) -> (w502:T14)  [unwired: 1 in]
                n336 = Bundle("Output Array"=w473, w468) -> (w501:cluster{"Output Array":dbl[], dbl[]})  [unwired: 1 in]
                n337 = Subtract(x=w438, y=w433) -> (x-y=w475:dbl[])
                n338 = Build Array(w509, w508) -> (→"Controller Output":T2)
                n339 = Build Array(w502, w512) -> (→"Velocity vs Controller output":T15)
                n340 = Subtract(x=w464, y=w433) -> (x-y=→"Displacement control error (mm)":dbl[])
                n341 = Bundle("Output Array"=w473, w438) -> ()  [unwired: 1 in, 1 out]
                n342 = Build Array(w506, w505, w504, w501) -> (→"Distance Graph":cluster{"Output Array":dbl[], dbl[]}[])
                n343 = Array Max & Min(array=w464) -> (max value=w472:dbl, min value=w471:dbl)  [unwired: 2 out]
                n344 = Subtract(x=w472, y=w471) -> (x-y=w470:dbl)
                n345 = Delete From Array(array=w442, length=2, index (row)=19) -> (array with subset deleted=w449:dbl[][])  [unwired: 1 in, 1 out]
                n346 = Index Array(array=w442, index (row)=T9."desired distance" ("Enum")) -> (element=w439:dbl[])  [unwired: 1 in]
                n347 = Array Size(array=w464) -> (size(s)=w469:i32)
                n348 = Array Size(array=w447) -> (size(s)=→"size(s) 2":i32)
                n349 = Divide(x=w470, y=w469) -> ()  [unwired: 1 out]
                n350 = Array Size(array=w446) -> (size(s)=→"size(s)":i32)
                n351 = Index Array(array=w442, index (row)=T9."predict distance" ("Enum")) -> (element=w440:dbl[])  [unwired: 1 in]
                n352 = Insert Into Array(array=w449, new element #1=w439, new element #2=w440, new element #3=w455, new element #4=w468, new element #5=w475) -> (w448:dbl[][])  [unwired: 2 in]
              }
            }
            n353 = Index Array(array=w355, index (row)=T9."Position Induktiv" ("Enum")) -> (element=w366:dbl[])  [unwired: 1 in]
            n354 = call "ADwin Get_FPar.vi"("Index"=u16 70, "Device No. (1)"=w360) -> ("ParameterValue"=w354:sgl)  [unwired: 7 in, 2 out]
            n355 = call "ADwin Get_FPar.vi"("Index"=u16 69, "Device No. (1)"=w360) -> ("ParameterValue"=w358:sgl)  [unwired: 7 in, 2 out]
            n356 = Index Array(array=w366, index=1) -> (element=w351:dbl)
            n357 = call "ADwin Get_FPar.vi"("Index"=u16 46, "Device No. (1)"=w360) -> ("ParameterValue"=w350:sgl)  [unwired: 7 in, 2 out]
            n358 = In Range and Coerce(upper limit=w358, x=w351, lower limit=0.0) -> (In Range?=w362:bool)  [unwired: 1 out]
            n359 = In Range and Coerce(upper limit=w354, x=w351, lower limit=w358) -> (In Range?=w356:bool)  [unwired: 1 out]
            n360 = In Range and Coerce(upper limit=w350, x=w351, lower limit=w354) -> (In Range?=w353:bool)  [unwired: 1 out]
            n361 = In Range and Coerce(upper limit=421.0, x=w351, lower limit=w350) -> (In Range?=w349:bool)  [unwired: 1 out]
            n362 = case shown="False" "Set file" {
              tunnel: w362 -> [_ w397]
              tunnel: w357 -> [w386 w396]
              tunnel: w356 -> [_ w395]
              tunnel: w353 -> [_ w394]
              tunnel: w347 -> [_ w393]
              tunnel: w349 -> [_ w392]
              tunnel: w348 -> [w385 _]
              tunnel: w347 -> [w384 _]
              frame False {
                (unwired) "save CPT data in one whole file"
                n363 = case shown="True" w384 {
                  tunnel: w386 -> [_ w387]
                  tunnel: w385 -> [_ w389]
                  frame False {
                  }
                  frame True {
                    w391 = TRUE ("append to file? (new file:F)")
                    n364 = call-poly <vilib>:"Write To Spreadsheet File.vi"("delimiter (\\t)"=";" ("delimiter (\\t)"), "transpose? (no:F)"=w391, "format (%.3f)"="%.;%.4f", "append to file? (new file:F)"=w391, "2D data"=w387, "file path (dialog if empty)"=w389) -> ()  [unwired: 2 in, 1 out]
                  }
                }
              }
              frame True {
                n365 = case shown="True" w393 {
                  tunnel: w397 -> [_ w406]
                  tunnel: w396 -> [_ w398]
                  tunnel: w395 -> [_ w405]
                  tunnel: w394 -> [_ w404]
                  tunnel: w392 -> [_ w403]
                  frame False {
                  }
                  frame True {
                    (unwired) "Store test data in different files"
                    n366 = case shown="True" w406 {
                      tunnel: w398 -> [_ w419]
                      tunnel: "Vibro test 1" -> [_ w418]
                      frame False {
                      }
                      frame True {
                        w421 = TRUE ("append to file? (new file:F)")
                        n367 = call-poly <vilib>:"Write To Spreadsheet File.vi"("delimiter (\\t)"=";" ("delimiter (\\t)"), "transpose? (no:F)"=w421, "format (%.3f)"="%.;%.4f", "append to file? (new file:F)"=w421, "2D data"=w419, "file path (dialog if empty)"=w418) -> ()  [unwired: 2 in, 1 out]
                      }
                    }
                    n368 = case shown="True" w405 {
                      tunnel: w398 -> [_ w414]
                      tunnel: "Vibro test 2" -> [_ w413]
                      frame False {
                      }
                      frame True {
                        w416 = TRUE ("append to file? (new file:F)")
                        n369 = call-poly <vilib>:"Write To Spreadsheet File.vi"("delimiter (\\t)"=";" ("delimiter (\\t)"), "transpose? (no:F)"=w416, "format (%.3f)"="%.;%.4f", "append to file? (new file:F)"=w416, "2D data"=w414, "file path (dialog if empty)"=w413) -> ()  [unwired: 2 in, 1 out]
                      }
                    }
                    n370 = case shown="True" w404 {
                      tunnel: w398 -> [_ w409]
                      tunnel: "Vibro test 3" -> [_ w408]
                      frame False {
                      }
                      frame True {
                        w411 = TRUE ("append to file? (new file:F)")
                        n371 = call-poly <vilib>:"Write To Spreadsheet File.vi"("delimiter (\\t)"=";" ("delimiter (\\t)"), "transpose? (no:F)"=w411, "format (%.3f)"="%.;%.4f", "append to file? (new file:F)"=w411, "2D data"=w409, "file path (dialog if empty)"=w408) -> ()  [unwired: 2 in, 1 out]
                      }
                    }
                    n372 = case shown="True" w403 {
                      tunnel: w398 -> [_ w424]
                      tunnel: "Static peneration test" -> [_ w423]
                      frame False {
                      }
                      frame True {
                        w426 = TRUE ("append to file? (new file:F)")
                        n373 = call-poly <vilib>:"Write To Spreadsheet File.vi"("delimiter (\\t)"=";" ("delimiter (\\t)"), "transpose? (no:F)"=w426, "format (%.3f)"="%.;%.4f", "append to file? (new file:F)"=w426, "2D data"=w424, "file path (dialog if empty)"=w423) -> ()  [unwired: 2 in, 1 out]
                      }
                    }
                  }
                }
              }
            }
          }
          frame #6 {
            (unwired) "Only use one period of data"
            (unwired) "Velocity deviation"
            (unwired) "acceleration"
            # "Perform correlation to get time delay"
            n374 = call "ADwin Get_Par.vi"("index"=i16 76, "Device No. (1)"=w531) -> ("ParameterValue"=w534:i32)  [unwired: 7 in, 2 out]
            n375 = Array Subset(array=w533, index (row)=0 ("index"), length (row)=w534) -> (w532:dbl[][])  [unwired: 2 in]
            n376 = Index Array(array=w537, index (row)=0) -> (element=w543:dbl[])  [unwired: 1 in]
            n377 = Index Array(array=w537, index (row)=1) -> (element=w540:dbl[])  [unwired: 1 in]
            n378 = Index Array(array=w532, index (row)=0) -> (element=w538:dbl[])  [unwired: 1 in]
            n379 = Bundle(w538, "Output Array 2"=w543) -> (→"Acceleration":cluster{dbl[], "Output Array 2":dbl[]})  [unwired: 1 in]
            n380 = Bundle(w538, "Output Array 2"=w540) -> (→"Velocity deviation":cluster{dbl[], "Output Array 2":dbl[]})  [unwired: 1 in]
            n381 = case shown="True" "Start Correlation" {
              tunnel: w532 -> [w547 w573]
              tunnel: w531 -> [_ w550]
              frame False {
                (unwired) "normalized velocity"
                n382 = Index Array(array=w547, index (row)=25) -> ()  [unwired: 1 in, 1 out]
                n383 = Index Array(array=w547, index (row)=26) -> ()  [unwired: 1 in, 1 out]
              }
              frame True {
                (unwired) "correlation between distance measurement and controller output"
                (unwired) 1 ("index (row)")
                (unwired) "normalized controller output"
                (unwired) "normalized velocity"
                n384 = call "ADwin Set_Par.vi"("Value"=0, "Index"=i16 9, "Device No."=w550) -> ()  [unwired: 6 in, 3 out]
                n385 = Index Array(array=w573, index (row)=T9."velocity data" ("Enum")) -> (element=w556:dbl[])  [unwired: 1 in]
                n386 = Index Array(array=w573, index (row)=T9."Distance_Regout" ("Enum")) -> (element=w555:dbl[])  [unwired: 1 in]
                n387 = Index Array(array=w573, index (row)=T9."Position Induktiv" ("Enum")) -> (element=w568:dbl[])  [unwired: 1 in]
                n388 = call-poly <vilib>:"Normalize.vi"("Vector"=w555) -> ("Normalized Vector"=w554:dbl[])  [unwired: 1 in, 3 out]
                n389 = Index Array(array=w573, index (row)=T9."Distance_Regout" ("Enum")) -> (element=w570:dbl[])  [unwired: 1 in]
                n390 = call-poly <vilib>:"Normalize.vi"("Vector"=w556) -> ("Normalized Vector"=w553:dbl[])  [unwired: 1 in, 3 out]
                n391 = Array Size(array=w553) -> (size(s)=w574:i32)
                n392 = call <vilib>:"Normalize Waveform.vi"("waveform in"=w568) -> ("normalized waveform"=w571:waveform(dbl))  [unwired: 7 in, 3 out]
                n393 = call <vilib>:"Normalize Waveform.vi"("waveform in"=w570) -> ("normalized waveform"=w569:waveform(dbl))  [unwired: 7 in, 3 out]
                n394 = Split 1D Array(array=w554, index=0) -> (second subarray=w552:dbl[])  [unwired: 1 out]
                n395 = Array Size(array=w568) -> (size(s)=w567:i32)
                n396 = call-poly <vilib>:"CrossCorrelation.vi"("Y"=w569, "X"=w571) -> ("Rxy"=w572:dbl[])  [unwired: 8 in, 1 out]
                n397 = Array Max & Min(array=w572) -> (max index (indices)=w575:i32)  [unwired: 3 out]
                n398 = call-poly <vilib>:"CrossCorrelation.vi"("normalization"=enum32{"none", "unbiased", "biased"}."none", "algorithm"=enum32{"direct", "frequency domain"}."direct", "Y"=w553, "X"=w552) -> ("Rxy"=w551:dbl[])  [unwired: 6 in, 1 out]
                "Correlation curve" <- w551
                n399 = Array Max & Min(array=w551) -> (max index (indices)=w583:i32)  [unwired: 3 out]
                n400 = Subtract(x=w583, y=w574) -> (x-y=w582:i32)
                n401 = Absolute Value(x=w582) -> (abs(x)=w559:i32)
                n402 = Subtract(x=w575, y=w567) -> (x-y=w576:i32)
                n403 = Absolute Value(x=w576) -> (abs(x)=w579:i32)
                n404 = Round To Nearest(number=w559) -> (nearest integer value=w561:i32)
                n405 = Divide(x=w579, y=1) -> (x/y=w577:dbl)
                n406 = Round To Nearest(number=w577) -> ()  [unwired: 1 out]
                n407 = Subtract(x=w561, y=0 ("index")) -> (x-y=w557:i32)
                n408 = Divide(x=w557, y=1) -> ()  [unwired: 1 out]
              }
            }
          }
          frame #7 {
            # "Visualize pressure control data"
            n409 = case shown="False" "Visualize data" {
              tunnel: w586 -> [_ w590]
              frame False {
              }
              frame True {
                n410 = Index Array(array=w590, index (row)=T9."Soll_Porepress" ("Enum")) -> (element=w614:dbl[])  [unwired: 1 in]
                n411 = expression code="12000/65536*x-6000"(w614) -> (w612:dbl[])
                n412 = Index Array(array=w590, index (row)=T9."Soll_Sidepress" ("Enum")) -> (element=w604:dbl[])  [unwired: 1 in]
                n413 = Index Array(array=w590, index (row)=T9."Program Counter" ("Enum")) -> (element=w613:dbl[])  [unwired: 1 in]
                n414 = Index Array(array=w590, index (row)=T9."Pore Pressure" ("Enum")) -> (element=w616:dbl[])  [unwired: 1 in]
                n415 = Index Array(array=w590, index (row)=T9."Soll_axialpress" ("Enum")) -> (element=w595:dbl[])  [unwired: 1 in]
                n416 = expression code="12000/65536*x-6000"(w604) -> (w602:dbl[])
                n417 = expression code="12000/65536*x -6000"(w595) -> (w593:dbl[])
                n418 = Index Array(array=w590, index (row)=T9."Program Counter" ("Enum")) -> (element=w603:dbl[])  [unwired: 1 in]
                n419 = Index Array(array=w590, index (row)=T9."Side Pressure " ("Enum")) -> (element=w606:dbl[])  [unwired: 1 in]
                n420 = Index Array(array=w590, index (row)=T9."Program Counter" ("Enum")) -> (element=w594:dbl[])  [unwired: 1 in]
                n421 = Index Array(array=w590, index (row)=T9."Axial Pressure" ("Enum")) -> (element=w597:dbl[])  [unwired: 1 in]
                n422 = Bundle("Output Array"=w613, "Output Array"=w616) -> (w611:T13)  [unwired: 1 in]
                n423 = Bundle("Output Array"=w613, "Output Array"=w612) -> (w610:T13)  [unwired: 1 in]
                n424 = Bundle("Output Array"=w603, "Output Array"=w606) -> (w601:T13)  [unwired: 1 in]
                n425 = Bundle("Output Array"=w594, "Output Array"=w597) -> (w592:T13)  [unwired: 1 in]
                n426 = Bundle("Output Array"=w603, "Output Array"=w602) -> (w600:T13)  [unwired: 1 in]
                n427 = Build Array(w611, w610) -> (→"Pore Pressure":T2)
                n428 = Bundle("Output Array"=w594, "Output Array"=w593) -> (w591:T13)  [unwired: 1 in]
                n429 = Build Array(w601, w600) -> (→"Side Pressure":T2)
                n430 = Build Array(w592, w591) -> (→"Axial Pressure":T2)
              }
            }
          }
          frame #8 {
            (unwired) "vibro paras for 1st test"
            # "Control parameters setup and activation, Switch frequency mode Setup"
            n431 = case shown="True" "Control start" {
              tunnel: w619 -> [w636 w640]
              frame False {
                n432 = call "ADwin Set_Par.vi"("Value"=sgl 0.0, "Index"=i16 39, "Device No."=w636) -> ()  [unwired: 6 in, 3 out]
              }
              frame True {
                n433 = property on="Record Data" class="Bool (strict)"("Value"=TRUE ("Record Data")) -> ()  [unwired: 2 in, 2 out]
                n434 = call "ADwin Set_Par.vi"("Value"=sgl 1.0, "Index"=i16 39, "Device No."=w640) -> ()  [unwired: 6 in, 3 out]
              }
            }
            n435 = case shown="True" TRUE {
              tunnel: w626 -> [_ _]
              tunnel: w619 -> [_ _]
              tunnel: w619 -> [_ w673]
              tunnel: w625 -> [_ _]
              tunnel: w619 -> [_ w679]
              tunnel: [w671 w677] -> w624
              tunnel: "Switch Vibro Mode" -> [w671 w677]
              frame False {
              }
              frame True {
                n436 = case shown="True" w677 {
                  tunnel: w679 -> [_ w749]
                  frame False {
                  }
                  frame True {
                    n437 = call "ADwin Set_FPar.vi"("Value"="Time delay-3", "Index"=i16 66, "Device No."=w749) -> ()  [unwired: 6 in, 3 out]
                  }
                }
                n438 = case shown="True" w677 {
                  tunnel: w679 -> [_ w746]
                  frame False {
                  }
                  frame True {
                    n439 = call "ADwin Set_FPar.vi"("Value"="Depth(mm)3", "Index"=i16 70, "Device No."=w746) -> ()  [unwired: 6 in, 3 out]
                  }
                }
                n440 = case shown="True" w677 {
                  tunnel: w673 -> [_ w751]
                  frame False {
                  }
                  frame True {
                    n441 = call "ADwin Set_Par.vi"("Value"=sgl 1.0, "Index"=i16 6, "Device No."=w751) -> ()  [unwired: 6 in, 3 out]
                  }
                }
                n442 = call "ADwin Get_Par.vi"("index"=i16 10, "Device No. (1)"=w673) -> ("ParameterValue"=w674:i32)  [unwired: 7 in, 2 out]
                n443 = call "ADwin Get_Par.vi"("index"=i16 11, "Device No. (1)"=w673) -> ("ParameterValue"=w678:i32)  [unwired: 7 in, 2 out]
                n444 = case shown="True" "Enable Vibro Mode 3" {
                  selector: "Enable Vibro Mode 3" -> [_ w715]
                  tunnel: w679 -> [_ w720]
                  tunnel: w678 -> [_ _]
                  tunnel: w677 -> [_ w719]
                  tunnel: w673 -> [_ w716]
                  frame False {
                  }
                  frame True {
                    n445 = call "ADwin Set_Par.vi"("Value"=1, "Index"=i16 35, "Device No."=w716) -> ()  [unwired: 6 in, 3 out]
                    n446 = case shown="True" w715 {
                      tunnel: w720 -> [_ w727]
                      tunnel: w719 -> [_ w733]
                      tunnel: w720 -> [_ w732]
                      tunnel: w720 -> [_ w731]
                      tunnel: w716 -> [w721 w724]
                      frame False {
                        n447 = call "ADwin Set_Par.vi"("Value"=0, "Index"=i16 36, "Device No."=w721) -> ()  [unwired: 6 in, 3 out]
                      }
                      frame True {
                        n448 = call "ADwin Set_Par.vi"("Value"=1, "Index"=i16 36, "Device No."=w724) -> ()  [unwired: 6 in, 3 out]
                        n449 = case shown="True" w733 {
                          tunnel: w727 -> [_ w743]
                          tunnel: "freq-3 ( Hz) 2" -> [_ w742]
                          frame False {
                          }
                          frame True {
                            n450 = call "ADwin Set_FPar.vi"("Value"=w742, "Index"=i16 49, "Device No."=w743) -> ()  [unwired: 6 in, 3 out]
                          }
                        }
                        n451 = case shown="True" w733 {
                          tunnel: w732 -> [_ w734]
                          tunnel: "Background velocity-3" -> [_ w735]
                          frame False {
                          }
                          frame True {
                            n452 = call "ADwin Set_FPar.vi"("Value"=w735, "Index"=i16 64, "Device No."=w734) -> ()  [unwired: 6 in, 3 out]
                          }
                        }
                        n453 = case shown="True" w733 {
                          tunnel: w731 -> [_ w740]
                          tunnel: "Amplitdue-3" -> [_ w739]
                          frame False {
                          }
                          frame True {
                            n454 = Multiply(x=w739, y=2.0) -> (x*y=w737:dbl)
                            n455 = call "ADwin Set_FPar.vi"("Value"=w737, "Index"=i16 48, "Device No."=w740) -> ()  [unwired: 6 in, 3 out]
                          }
                        }
                      }
                    }
                  }
                }
                n456 = case shown="True" "Enable static penetration" {
                  tunnel: w673 -> [_ w684]
                  frame False {
                  }
                  frame True {
                    n457 = call "ADwin Set_FPar.vi"("Value"="Time delay - 4", "Index"=i16 47, "Device No."=w684) -> ()  [unwired: 6 in, 3 out]
                    n458 = call "ADwin Set_FPar.vi"("Value"="Static penetration Depth(mm) - 4", "Index"=i16 46, "Device No."=w684) -> ()  [unwired: 6 in, 3 out]
                  }
                }
                n459 = case shown="True" w677 {
                  tunnel: w679 -> [_ w757]
                  frame False {
                  }
                  frame True {
                    n460 = call "ADwin Set_FPar.vi"("Value"="Time delay-2", "Index"=i16 65, "Device No."=w757) -> ()  [unwired: 6 in, 3 out]
                  }
                }
                n461 = case shown="True" w677 {
                  tunnel: w679 -> [_ w755]
                  frame False {
                  }
                  frame True {
                    n462 = call "ADwin Set_FPar.vi"("Value"="Depth(mm)2", "Index"=i16 69, "Device No."=w755) -> ()  [unwired: 6 in, 3 out]
                  }
                }
                n463 = case shown="True" "Enable Vibro Mode 2" {
                  selector: "Enable Vibro Mode 2" -> [_ w687]
                  tunnel: w674 -> [_ _]
                  tunnel: w679 -> [_ w692]
                  tunnel: w677 -> [_ w691]
                  tunnel: w673 -> [_ w688]
                  frame False {
                  }
                  frame True {
                    n464 = call "ADwin Set_Par.vi"("Value"=1, "Index"=i16 34, "Device No."=w688) -> ()  [unwired: 6 in, 3 out]
                    n465 = case shown="True" w687 {
                      tunnel: w692 -> [_ w700]
                      tunnel: w691 -> [_ w699]
                      tunnel: w688 -> [w693 w696]
                      frame False {
                        n466 = call "ADwin Set_Par.vi"("Value"=0, "Index"=i16 36, "Device No."=w693) -> ()  [unwired: 6 in, 3 out]
                      }
                      frame True {
                        n467 = call "ADwin Set_Par.vi"("Value"=1, "Index"=i16 36, "Device No."=w696) -> ()  [unwired: 6 in, 3 out]
                        n468 = case shown="True" w699 {
                          tunnel: w700 -> [_ w713]
                          tunnel: "freq-2 ( Hz)" -> [_ w712]
                          frame False {
                          }
                          frame True {
                            n469 = call "ADwin Set_FPar.vi"("Value"=w712, "Index"=i16 38, "Device No."=w713) -> ()  [unwired: 6 in, 3 out]
                          }
                        }
                        n470 = case shown="True" w699 {
                          tunnel: w700 -> [_ w710]
                          tunnel: "Amplitdue-2" -> [_ w709]
                          frame False {
                          }
                          frame True {
                            n471 = Multiply(x=w709, y=2.0) -> (x*y=w707:dbl)
                            n472 = call "ADwin Set_FPar.vi"("Value"=w707, "Index"=i16 37, "Device No."=w710) -> ()  [unwired: 6 in, 3 out]
                          }
                        }
                        n473 = case shown="True" w699 {
                          tunnel: w700 -> [_ w705]
                          tunnel: "Background velocity-2" -> [_ w704]
                          frame False {
                          }
                          frame True {
                            n474 = call "ADwin Set_FPar.vi"("Value"=w704, "Index"=i16 39, "Device No."=w705) -> ()  [unwired: 6 in, 3 out]
                          }
                        }
                      }
                    }
                  }
                }
              }
            }
            n475 = case shown="True" "Control Stop" {
              tunnel: w619 -> [w664 w668]
              frame False {
                n476 = call "ADwin Set_FPar.vi"("Value"=sgl 0.0, "Index"=i16 71, "Device No."=w664) -> ()  [unwired: 6 in, 3 out]
              }
              frame True {
                w667 = FALSE ("Record Data")
                n477 = call "ADwin Set_FPar.vi"("Value"=sgl 1.0, "Index"=i16 71, "Device No."=w668) -> ()  [unwired: 6 in, 3 out]
                n478 = property on="Record Data" class="Bool (strict)"("Value"=w667) -> ()  [unwired: 2 in, 2 out]
                n479 = property on="Control start" class="Bool (strict)"("Value"=w667) -> ()  [unwired: 2 in, 2 out]
              }
            }
            n480 = case shown="False" "Finish test" {
              tunnel: w619 -> [_ w633]
              tunnel: w619 -> [w628 _]
              frame False {
                n481 = case shown="False" "Activate" {
                  tunnel: w628 -> [_ w630]
                  frame False {
                  }
                  frame True {
                    n482 = call "ADwin Set_Par.vi"("Value"=sgl 12.0, "Index"=i16 80, "Device No."=w630) -> ()  [unwired: 6 in, 3 out]
                  }
                }
              }
              frame True {
                n483 = call "ADwin Set_Par.vi"("Value"=sgl 1.0, "Index"=i16 15, "Device No."=w633) -> ()  [unwired: 6 in, 3 out]
              }
            }
            n484 = case shown="False" w624 {
              tunnel: w619 -> [w643 _]
              frame False {
                n485 = case shown="True" "Enable Vibro Mode 1" {
                  tunnel: w643 -> [_ w651]
                  frame False {
                  }
                  frame True {
                    w645 = 0.5 ("y")
                    n486 = Multiply(x="Amplitude - 1 (mm)", y=2.0) -> (x*y=w648:dbl)
                    n487 = case shown="True" TRUE {
                      tunnel: w651 -> [_ _]
                      tunnel: "Vibration frequency - 1  (Hz)" -> [_ w662]
                      tunnel: w651 -> [_ w661]
                      frame False {
                      }
                      frame True {
                        n488 = call "ADwin Set_FPar.vi"("Value"=w662, "Index"=i16 26, "Device No."=w661) -> ()  [unwired: 6 in, 3 out]
                      }
                    }
                    n489 = Less?(x="background velocity -1 (mm/s)", y=w645) -> (x < y?=w647:bool)
                    n490 = call "ADwin Set_FPar.vi"("Value"=w648, "Index"=i16 23, "Device No."=w651) -> ()  [unwired: 6 in, 3 out]
                    n491 = case shown="True" w647 {
                      tunnel: w651 -> [w656 w659]
                      tunnel: "background velocity -1 (mm/s)" -> [w655 w658]
                      tunnel: w645 -> [_ _]
                      frame False {
                        n492 = call "ADwin Set_FPar.vi"("Value"=w655, "Index"=i16 24, "Device No."=w656) -> ()  [unwired: 6 in, 3 out]
                      }
                      frame True {
                        n493 = call "ADwin Set_FPar.vi"("Value"=w658, "Index"=i16 24, "Device No."=w659) -> ()  [unwired: 6 in, 3 out]
                      }
                    }
                  }
                }
              }
              frame True {
              }
            }
          }
          frame #9 {
            # "LCT_strain_based_control"
            n494 = property on="LCT strain-based \ncontrol activate" class="Bool (strict)"() -> ("Value"=w762:bool)  [unwired: 2 in, 2 out]
            n495 = Boolean To (0,1)(Boolean=w762) -> (0, 1=w760:i16)
            n496 = case shown="True" w762 {
              tunnel: w761 -> [_ w772]
              tunnel: w761 -> [_ w768]
              tunnel: w760 -> [_ w769]
              frame False {
              }
              frame True {
                (unwired) "disable LCT strain based onctrol, when LCT testing is finished"
                n497 = property on="LCT test finish" class="Bool (strict)"() -> ("Value"=w770:bool)  [unwired: 2 in, 2 out]
                n498 = Not(x=w770) -> (.not. x?=w771:bool)
                n499 = case shown="False" w771 {
                  tunnel: w769 -> [_ w779]
                  tunnel: w768 -> [_ w778]
                  frame False {
                    n500 = Not(x="LCT control finish") -> (.not. x?=w775:bool)
                    n501 = property on="LCT strain-based control activate" class="Bool (strict)"("Value"=w775) -> ()  [unwired: 2 in, 2 out]
                    n502 = property on="Go - Seitendruck" class="Bool (strict)"("Value"=w775) -> ()  [unwired: 2 in, 2 out]
                  }
                  frame True {
                    n503 = call "ADwin Set_Par.vi"("Value"=w779, "Index"=i16 66, "Device No."=w778) -> ()  [unwired: 6 in, 3 out]
                  }
                }
                n504 = case shown="\"set strain for pore\\n volume tric strain\"" "Trigger condition\n of Stop loading" {
                  tunnel: w772 -> [w783 w806]
                  tunnel: [w787 w805] -> w765
                  tunnel: [w787 w805] -> w764
                  frame "Set volume change threshold", Default {
                    w785 = u16 67 items=["NaN", "Kp_Position_Vibro", "Ki_Position_Vibro", "PAR_3", "Sinusfrequenz_preSh", "Zylinder_Move_Button", "PAR_6", "PAR_7", "PAR_8", "PAR_9", "PAR_10", "PAR_11", "PAR_12", "Amplitude_PreSh", "Compass_OFF", "PAR_15", "PAR_16", "SollMoog", "PAR_18", "PAR_19", "PAR_20", "Vibro_Test_Button", "PAR_22", "PAR_23", "PAR_24", "PAR_25", "PAR_26", "PAR_27", "PAR_28", "PAR_29", "PAR_30", "PAR_31", "PAR_32", "Start_Test_Button", "PAR_34", "Programm_counter", "PAR_36", "Circumference_ON_Flag", "PAR_38", "PAR_39", "Pore_Control_Button", "Side_Control_Button", "Axial_Control_Button", "PAR_43", "PAR_44", "PAR_45", "Einfahren_Piston", "PAR_47", "PAR_48", "PAR_49", "PAR_50", "PAR_51", "PAR_52", "PAR_53", "PAR_54", "PAR_55", "PAR_56", "PAR_57", "LinearUpDown_Button", "Linear_Pore_GO", "Linear_Axial_GO", "Linear_Side_GO", "PAR_62", "PAR_63", "PAR_64", "PAR_65", "LCT_strain_based_control_activate", "LCT_strain_based_trigger_condition", "PAR_68", "PAR_69", "Pre_Shearing_Button", "PAR_71", "PAR_72", "PAR_73", "PAR_74", "Circumf_Control_On", "PAR_76", "PAR_77", "PAR_78", "PAR_79", "Modus", "", "", "", "", "", "", "", "", "", "", "", "", "", "", "", "", "", "", "", "", "", "", "", "", "", ""] ("par_enum")
                    n505 = call "ADwin Get_FPar.vi"("Index"=u16 33, "Device No. (1)"=w783) -> ("ParameterValue"=w787:sgl)  [unwired: 7 in, 2 out]
                    n506 = call "ADwin Set_FPar.vi"("Value"="maximum acceptable \nside volume change (ml)", "Index"=i16 32, "Device No."=w783) -> ()  [unwired: 6 in, 3 out]
                    n507 = case shown="True" "Display" {
                      frame False {
                      }
                      frame True {
                        n508 = local read "Pore Pressure [KPa]"() -> (w799:dbl)
                        n509 = local read "Side Pressure  [KPa]"() -> (w800:dbl)
                        n510 = local read "Side"() -> (w798:dbl)
                        n511 = Subtract(x=w800, y=w799) -> (x-y=w796:dbl)
                        n512 = feedback #1() -> (w797:dbl[])  [unwired: 1 in]
                        n513 = Insert Into Array(array=w797, new element=w798) -> (w794:dbl[])  [unwired: 1 in]
                        n514 = feedback-in #1(w794) -> ()
                        n515 = feedback #2() -> (w795:dbl[])  [unwired: 1 in]
                        n516 = Insert Into Array(array=w795, new element=w796) -> (w792:dbl[])  [unwired: 1 in]
                        n517 = feedback-in #2(w792) -> ()
                        n518 = call "Convert to Dynamic Data2"("Array"=w792) -> ("Dynamic Data Type"=w791:dynamicdata)  [unwired: 3 in]
                        n519 = call "Convert to Dynamic Data"("Array"=w794) -> ("Dynamic Data Type"=w793:dynamicdata)  [unwired: 3 in]
                        n520 = call "Build XY Graph"("Y Input"=w793, "X Input"=w791) -> ("XY Graph"=→"Side volume - Effective lateral Stress":cluster{"X":dbl[], "Y":dbl[]}[])  [unwired: 8 in, 1 out]
                      }
                    }
                    n521 = call "ADwin Set_Par.vi"("Value"=1, "Index"=w785, "Device No."=w783) -> ()  [unwired: 6 in, 3 out]
                  }
                  frame "set strain for pore\n volume tric strain" {
                    w808 = u16 67 items=["NaN", "Kp_Position_Vibro", "Ki_Position_Vibro", "PAR_3", "Sinusfrequenz_preSh", "Zylinder_Move_Button", "PAR_6", "PAR_7", "PAR_8", "PAR_9", "PAR_10", "PAR_11", "PAR_12", "Amplitude_PreSh", "Compass_OFF", "PAR_15", "PAR_16", "SollMoog", "PAR_18", "PAR_19", "PAR_20", "Vibro_Test_Button", "PAR_22", "PAR_23", "PAR_24", "PAR_25", "PAR_26", "PAR_27", "PAR_28", "PAR_29", "PAR_30", "PAR_31", "PAR_32", "Start_Test_Button", "PAR_34", "Programm_counter", "PAR_36", "Circumference_ON_Flag", "PAR_38", "PAR_39", "Pore_Control_Button", "Side_Control_Button", "Axial_Control_Button", "PAR_43", "PAR_44", "PAR_45", "Einfahren_Piston", "PAR_47", "PAR_48", "PAR_49", "PAR_50", "PAR_51", "PAR_52", "PAR_53", "PAR_54", "PAR_55", "PAR_56", "PAR_57", "LinearUpDown_Button", "Linear_Pore_GO", "Linear_Axial_GO", "Linear_Side_GO", "PAR_62", "PAR_63", "PAR_64", "PAR_65", "LCT_strain_based_control_activate", "LCT_strain_based_trigger_condition", "PAR_68", "PAR_69", "Pre_Shearing_Button", "PAR_71", "PAR_72", "PAR_73", "PAR_74", "Circumf_Control_On", "PAR_76", "PAR_77", "PAR_78", "PAR_79", "Modus", "", "", "", "", "", "", "", "", "", "", "", "", "", "", "", "", "", "", "", "", "", "", "", "", "", ""] ("par_enum")
                    n522 = call "ADwin Get_FPar.vi"("Index"=T12."actual side volume change / actual pore volumetric strain " ("Enum"), "Device No. (1)"=w806) -> ("ParameterValue"=w805:sgl)  [unwired: 7 in, 2 out]
                    n523 = call "ADwin Set_Par.vi"("Value"=2, "Index"=w808, "Device No."=w806) -> ()  [unwired: 6 in, 3 out]
                    n524 = call "ADwin Set_FPar.vi"("Value"="volumetric strain", "Index"=T12."volume change/ pore volumetric strain " ("Enum"), "Device No."=w806) -> ()  [unwired: 6 in, 3 out]
                  }
                }
                "Change of side volume (ml)/ actual volumetric strain" <- w765
                "Strain curve based on side volume change" <- w764
                n525 = call "ADwin Get_Par.vi"("index"=i16 66, "Device No. (1)"=w768) -> ("ParameterValue"=w774:i32)  [unwired: 7 in, 2 out]
                n526 = local read "LCT test finish"() -> (w766:bool)
                n527 = Not(x=w766) -> (.not. x?=w767:bool)
                n528 = property on="Regelung Akiv Sidepressure" class="Bool (strict)"("Value"=w767) -> ()  [unwired: 2 in, 2 out]
                n529 = case shown="1" w774 {
                  frame 0, Default {
                    n530 = property on="LCT test finish" class="Bool (strict)"("Value"=TRUE ("LCT test finish")) -> ()  [unwired: 2 in, 2 out]
                    n531 = property on="Record Data" class="Bool (strict)"("Value"=FALSE ("Record Data")) -> ()  [unwired: 2 in, 2 out]
                  }
                  frame 1 {
                    "LCT test finish" <- FALSE ("LCT test finish")
                  }
                }
              }
            }
          }
          frame #10 {
            # "Linear calibration with BC5"
            n532 = call "ADwin Get_FPar_Block.vi"("count"=i16 80, "startindex"=i16 1, "Device No."=w812) -> ("Data"=w811:sgl[], "Device No. out"=w810:u16)  [unwired: 2 in, 2 out]
            n533 = case shown="True" "Calibration start" {
              tunnel: w811 -> [_ _]
              tunnel: w810 -> [w816 w824]
              tunnel: w809 -> [_ w821]
              frame False {
                n534 = call "ADwin Set_Par.vi"("Value"=sgl 0.0, "Index"=i16 72, "Device No."=w816) -> ()  [unwired: 6 in, 3 out]
              }
              frame True {
                (unwired) " Position of Piston"
                (unwired) "Strain"
                (unwired) "Additional Side Pressure"
                n535 = call "ADwin Set_Par.vi"("Value"=sgl 1.0, "Index"=i16 72, "Device No."=w824) -> ()  [unwired: 6 in, 3 out]
                n536 = Index Array(array=w821, index (row)=2) -> (element=→"Piston Position (mm)":dbl[])  [unwired: 1 in]
                n537 = Index Array(array=w821, index (row)=30) -> (element=w835:dbl[])  [unwired: 1 in]
                n538 = Index Array(array=w821, index (row)=31) -> (element=w834:dbl[])  [unwired: 1 in]
                n539 = Bundle("Output Array"=w835, "Output Array"=w834) -> (→"Linear calibration":T13)  [unwired: 1 in]
                n540 = call "ADwin Set_FPar.vi"("Value"="Starting penetration depth (mm)  2", "Index"=i16 29, "Device No."=w824) -> ()  [unwired: 6 in, 3 out]
                n541 = call "ADwin Set_FPar.vi"("Value"="initial radius r0", "Index"=i16 30) -> ()  [unwired: 7 in, 3 out]
                n542 = call "ADwin Set_FPar.vi"("Value"="Initial cone position (mm)", "Index"=i16 31, "Device No."=w824) -> ()  [unwired: 6 in, 3 out]
              }
            }
          }
          frame #11 {
            # "Linear Pressure Control"
            n543 = local read "Delta Seiten"() -> (w843:dbl)
            n544 = local read "Delta Axial"() -> (w838:dbl)
            n545 = local read "Go - Porendruck"() -> (w850:bool)
            n546 = local read "Go - Seitendruck"() -> (w845:bool)
            n547 = local read "Go - Axialdruck"() -> (w840:bool)
            n548 = local read "Delta Pore"() -> (w848:dbl)
            n549 = Greater?(x=w838, y=0.0) -> (0:w841:bool)
            n550 = Greater?(x=w843, y=0.0) -> (0:w846:bool)
            n551 = Greater?(x=w848, y=0.0) -> (0:w851:bool)
            n552 = And(x=w840, y=w841) -> (x .and. y?=w839:bool)
            n553 = And(x=w845, y=w846) -> (x .and. y?=w844:bool)
            n554 = And(x=w850, y=w851) -> (x .and. y?=w849:bool)
            n555 = local read "Up_Lower"() -> (w854:bool)
            n556 = case shown="True" w849 {
              tunnel: w854 -> [w902 w910]
              tunnel: [w902 w910] -> w853
              tunnel: w836 -> [_ w905]
              frame False {
                n557 = local read "Pore Pressure [KPa]"() -> (→"Porendruck save":dbl)
              }
              frame True {
                n558 = local read "Porendruck save"() -> (w908:dbl)
                n559 = local read "Porepressure"() -> (w904:dbl)
                n560 = case shown="True" w910 {
                  tunnel: "Delta Pore" -> [w920 w924]
                  tunnel: w908 -> [w919 w925]
                  tunnel: [w918 w923] -> w907
                  tunnel: w904 -> [w917 w922]
                  tunnel: [w916 w921] -> w906
                  frame False {
                    n561 = Subtract(x=w919, y=w920) -> (x-y=w918:dbl)
                    n562 = Greater?(x=w918, y=w917) -> (0:w916:bool)
                  }
                  frame True {
                    n563 = Add(x=w925, y=w924) -> (x+y=w923:dbl)
                    n564 = Greater?(x=w922, y=w923) -> (0:w921:bool)
                  }
                }
                n565 = case shown="True" w906 {
                  tunnel: w905 -> [_ w912]
                  frame False {
                  }
                  frame True {
                    w913 = u16 59 items=["NaN", "Kp_Position_Vibro", "Ki_Position_Vibro", "PAR_3", "Sinusfrequenz_preSh", "Zylinder_Move_Button", "PAR_6", "PAR_7", "PAR_8", "PAR_9", "PAR_10", "PAR_11", "PAR_12", "Amplitude_PreSh", "Compass_OFF", "PAR_15", "PAR_16", "SollMoog", "PAR_18", "PAR_19", "PAR_20", "Vibro_Test_Button", "PAR_22", "PAR_23", "PAR_24", "PAR_25", "PAR_26", "PAR_27", "PAR_28", "PAR_29", "PAR_30", "PAR_31", "PAR_32", "Start_Test_Button", "PAR_34", "Programm_counter", "PAR_36", "Circumference_ON_Flag", "PAR_38", "PAR_39", "Pore_Control_Button", "Side_Control_Button", "Axial_Control_Button", "PAR_43", "PAR_44", "PAR_45", "Einfahren_Piston", "PAR_47", "PAR_48", "PAR_49", "PAR_50", "PAR_51", "PAR_52", "PAR_53", "PAR_54", "PAR_55", "PAR_56", "PAR_57", "LinearUpDown_Button", "Linear_Pore_GO", "Linear_Axial_GO", "Linear_Side_GO", "PAR_62", "PAR_63", "PAR_64", "PAR_65", "PAR_66", "PAR_67", "PAR_68", "PAR_69", "Pre_Shearing_Button", "PAR_71", "PAR_72", "PAR_73", "PAR_74", "Circumf_Control_On", "PAR_76", "PAR_77", "PAR_78", "PAR_79", "Modus", "", "", "", "", "", "", "", "", "", "", "", "", "", "", "", "", "", "", "", "", "", "", "", "", "", ""] ("par_enum")
                    n566 = local write "Go - Porendruck"(FALSE ("Go - Porendruck")) -> ()
                    n567 = local write "Delta Pore"(0.0 ("Delta Pore")) -> ()
                    n568 = call "ADwin Set_Par.vi"("Value"=0, "Index"=w913, "Device No."=w912) -> ()  [unwired: 6 in, 3 out]
                  }
                }
                n569 = local write "Soll Pore Pressure"(w907) -> ()
              }
            }
            n570 = case shown="True" w844 {
              tunnel: w853 -> [w879 w886]
              tunnel: [w879 w886] -> w852
              tunnel: w836 -> [_ w881]
              frame False {
                n571 = local read "Side Pressure  [KPa]"() -> (→"Seitendruck save":dbl)
              }
              frame True {
                n572 = local read "Seitendruck save"() -> (w884:dbl)
                n573 = local read "Sidepressure"() -> (w880:dbl)
                n574 = case shown="True" w886 {
                  tunnel: "Delta Seiten" -> [w896 w900]
                  tunnel: w884 -> [w895 w901]
                  tunnel: [w894 w899] -> w882
                  tunnel: w880 -> [w893 w898]
                  tunnel: [w892 w897] -> w883
                  frame False {
                    n575 = Subtract(x=w895, y=w896) -> (x-y=w894:dbl)
                    n576 = Greater?(x=w894, y=w893) -> (0:w892:bool)
                  }
                  frame True {
                    n577 = Add(x=w901, y=w900) -> (x+y=w899:dbl)
                    n578 = Greater?(x=w898, y=w899) -> (0:w897:bool)
                  }
                }
                n579 = local write "Soll Side Pressure"(w882) -> ()
                n580 = case shown="True" w883 {
                  tunnel: w881 -> [_ w888]
                  frame False {
                  }
                  frame True {
                    w889 = u16 61 items=["NaN", "Kp_Position_Vibro", "Ki_Position_Vibro", "PAR_3", "Sinusfrequenz_preSh", "Zylinder_Move_Button", "PAR_6", "PAR_7", "PAR_8", "PAR_9", "PAR_10", "PAR_11", "PAR_12", "Amplitude_PreSh", "Compass_OFF", "PAR_15", "PAR_16", "SollMoog", "PAR_18", "PAR_19", "PAR_20", "Vibro_Test_Button", "PAR_22", "PAR_23", "PAR_24", "PAR_25", "PAR_26", "PAR_27", "PAR_28", "PAR_29", "PAR_30", "PAR_31", "PAR_32", "Start_Test_Button", "PAR_34", "Programm_counter", "PAR_36", "Circumference_ON_Flag", "PAR_38", "PAR_39", "Pore_Control_Button", "Side_Control_Button", "Axial_Control_Button", "PAR_43", "PAR_44", "PAR_45", "Einfahren_Piston", "PAR_47", "PAR_48", "PAR_49", "PAR_50", "PAR_51", "PAR_52", "PAR_53", "PAR_54", "PAR_55", "PAR_56", "PAR_57", "LinearUpDown_Button", "Linear_Pore_GO", "Linear_Axial_GO", "Linear_Side_GO", "PAR_62", "PAR_63", "PAR_64", "PAR_65", "PAR_66", "PAR_67", "PAR_68", "PAR_69", "Pre_Shearing_Button", "PAR_71", "PAR_72", "PAR_73", "PAR_74", "Circumf_Control_On", "PAR_76", "PAR_77", "PAR_78", "PAR_79", "Modus", "", "", "", "", "", "", "", "", "", "", "", "", "", "", "", "", "", "", "", "", "", "", "", "", "", ""] ("par_enum")
                    n581 = local write "Go - Seitendruck"(FALSE ("Go - Seitendruck")) -> ()
                    n582 = local write "Delta Seiten"(0.0 ("Delta Seiten")) -> ()
                    n583 = call "ADwin Set_Par.vi"("Value"=0, "Index"=w889, "Device No."=w888) -> ()  [unwired: 6 in, 3 out]
                  }
                }
              }
            }
            n584 = case shown="True" w839 {
              tunnel: w852 -> [_ w862]
              tunnel: w836 -> [_ w857]
              frame False {
                n585 = local read "Axial Pressure  [KPa]"() -> (→"Axialdruck save":dbl)
              }
              frame True {
                n586 = local read "Axialdruck save"() -> (w860:dbl)
                n587 = local read "Axialpressure"() -> (w856:dbl)
                n588 = case shown="True" w862 {
                  tunnel: "Delta Axial" -> [w872 w876]
                  tunnel: w860 -> [w871 w877]
                  tunnel: [w870 w875] -> w858
                  tunnel: w856 -> [w869 w874]
                  tunnel: [w868 w873] -> w859
                  frame False {
                    n589 = Subtract(x=w871, y=w872) -> (x-y=w870:dbl)
                    n590 = Greater?(x=w870, y=w869) -> (0:w868:bool)
                  }
                  frame True {
                    n591 = Add(x=w877, y=w876) -> (x+y=w875:dbl)
                    n592 = Greater?(x=w874, y=w875) -> (0:w873:bool)
                  }
                }
                n593 = case shown="True" w859 {
                  tunnel: w857 -> [_ w864]
                  frame False {
                  }
                  frame True {
                    w865 = u16 60 items=["NaN", "Kp_Position_Vibro", "Ki_Position_Vibro", "PAR_3", "Sinusfrequenz_preSh", "Zylinder_Move_Button", "PAR_6", "PAR_7", "PAR_8", "PAR_9", "PAR_10", "PAR_11", "PAR_12", "Amplitude_PreSh", "Compass_OFF", "PAR_15", "PAR_16", "SollMoog", "PAR_18", "PAR_19", "PAR_20", "Vibro_Test_Button", "PAR_22", "PAR_23", "PAR_24", "PAR_25", "PAR_26", "PAR_27", "PAR_28", "PAR_29", "PAR_30", "PAR_31", "PAR_32", "Start_Test_Button", "PAR_34", "Programm_counter", "PAR_36", "Circumference_ON_Flag", "PAR_38", "PAR_39", "Pore_Control_Button", "Side_Control_Button", "Axial_Control_Button", "PAR_43", "PAR_44", "PAR_45", "Einfahren_Piston", "PAR_47", "PAR_48", "PAR_49", "PAR_50", "PAR_51", "PAR_52", "PAR_53", "PAR_54", "PAR_55", "PAR_56", "PAR_57", "LinearUpDown_Button", "Linear_Pore_GO", "Linear_Axial_GO", "Linear_Side_GO", "PAR_62", "PAR_63", "PAR_64", "PAR_65", "PAR_66", "PAR_67", "PAR_68", "PAR_69", "Pre_Shearing_Button", "PAR_71", "PAR_72", "PAR_73", "PAR_74", "Circumf_Control_On", "PAR_76", "PAR_77", "PAR_78", "PAR_79", "Modus", "", "", "", "", "", "", "", "", "", "", "", "", "", "", "", "", "", "", "", "", "", "", "", "", "", ""] ("par_enum")
                    n594 = local write "Go - Axialdruck"(FALSE ("Go - Axialdruck")) -> ()
                    n595 = local write "Delta Axial"(0.0 ("Delta Axial")) -> ()
                    n596 = call "ADwin Set_Par.vi"("Value"=0, "Index"=w865, "Device No."=w864) -> ()  [unwired: 6 in, 3 out]
                  }
                }
                n597 = local write "Soll Axial Pressure"(w858) -> ()
              }
            }
          }
          frame #12 {
            # "Pre-Shearing"
            n598 = case shown="True" TRUE {
              frame False {
              }
              frame True {
                n599 = local read "Duration of Cycle SOLL"() -> (w930:i32)
                n600 = local read "Pre-shearing output"() -> (w932:dbl)
                n601 = local read "Start Pre-Shearing"() -> (w931:bool)
                n602 = local read "Axial Pressure  [KPa]"() -> (w953:dbl)
                n603 = Multiply(x=w930, y="Number of Cycles SOLL") -> (x*y=w929:dbl)
                n604 = local read "Pore Pressure [KPa]"() -> (w950:dbl)
                "Abweichung Pore" <- w950
                n605 = local read "Side Pressure  [KPa]"() -> (w937:dbl)
                "Abweichung Side" <- w937
                n606 = Bundle("Axial Pressure  [KPa]"=w953, "Pre-shearing output"=w932) -> (→"Sollvorgabe":T5)  [unwired: 1 in]
                n607 = Subtract(x="Sollwert Porenwasser", y="Erlaubte  Max Abweichung Pore") -> (x-y=w947:dbl)
                n608 = Add(x="Sollwert Seitendruck", y="Erlaubte Max Abweichung Side") -> (x+y=w940:dbl)
                n609 = Subtract(x="Sollwert Seitendruck", y="Erlaubte Max Abweichung Side") -> (x-y=w941:dbl)
                n610 = Add(x="Sollwert Porenwasser", y="Erlaubte  Max Abweichung Pore") -> (x+y=w946:dbl)
                n611 = case shown="False" w931 {
                  tunnel: w929 -> [_ w964]
                  frame False {
                    n612 = Tick Count (ms)() -> (millisecond timer value=w957:u32)
                    n613 = Divide(x=w957, y=u32 1000) -> (x/y=→"ms Offset Pre-Shearing":dbl)
                  }
                  frame True {
                    n614 = Tick Count (ms)() -> (millisecond timer value=w963:u32)
                    n615 = local read "ms Offset Pre-Shearing"() -> (w965:u32)
                    n616 = Divide(x=w963, y=u32 1000) -> (x/y=w961:dbl)
                    n617 = Subtract(x=w961, y=w965) -> (x-y=w960:dbl)
                    "S" <- w960
                    n618 = Greater?(x=w960, y=w964) -> (0:w959:bool)
                    "Pre-Shearing Ended Successful:" <- w959
                    n619 = case shown="True" w959 {
                      frame False {
                      }
                      frame True {
                        n620 = local write "Start Pre-Shearing"(FALSE ("Par_70")) -> ()
                      }
                    }
                    "Total Elapsed Seconds" <- w964
                  }
                }
                n621 = Greater?(x=w937, y=w940) -> (0:w942:bool)
                n622 = Less?(x=w937, y=w941) -> (x < y?=w943:bool)
                n623 = Greater?(x=w950, y=w946) -> (0:w948:bool)
                n624 = Less?(x=w950, y=w947) -> (x < y?=w949:bool)
                n625 = Subtract(x=w932, y=w953) -> (x-y=w955:dbl)
                "Abweichung Axial" <- w955
                n626 = Absolute Value(x=w955) -> (abs(x)=w954:dbl)
                n627 = Or(x=w942, y=w943) -> (x .or. y?=w933:bool)
                "Side Alarm" <- w933
                n628 = Greater?(x=w954, y="Erlaubte Max Abweichung Axial") -> (0:w935:bool)
                "Axial Alarm" <- w935
                n629 = Or(x=w948, y=w949) -> (x .or. y?=w934:bool)
                "Pore Alarm" <- w934
                n630 = Compound Arithmetic op=OR(w935, w934, w933) -> (w936:bool)
                n631 = case shown="True" w936 {
                  frame False {
                  }
                  frame True {
                    "Alarm Triggered" <- FALSE ("result")
                  }
                }
              }
            }
            n632 = case shown="True" "Reset Alarm" {
              frame False {
              }
              frame True {
                n633 = local write "Alarm Triggered"(FALSE ("result")) -> ()
              }
            }
          }
          frame #13 {
            # "End of Test Check"
            n634 = local read "Axial Pressure  [KPa]"() -> (w984:dbl)
            n635 = local read "Side Pressure  [KPa]"() -> (w985:dbl)
            n636 = local read "Pore Pressure [KPa]"() -> (w987:dbl)
            n637 = local read "start penetration"() -> (w970:bool)
            n638 = local read "Position Piston"() -> (w977:dbl)
            n639 = local read "Test Flag"() -> (w978:bool)
            n640 = local read "Turn off BC5"() -> (w975:bool)
            n641 = Less?(x=w984, y=70.0) -> (x < y?=w981:bool)
            "Axial Pressure okay:" <- w981
            n642 = Less?(x=w985, y=70.0) -> (x < y?=w982:bool)
            "Side Pressure okay:" <- w982
            n643 = Less?(x=w987, y=70.0) -> (x < y?=w983:bool)
            "Pore Pressure okay:" <- w983
            n644 = Greater?(x=w977, y=419.0) -> (0:w972:bool)
            n645 = Not(x=w970) -> (.not. x?=w969:bool)
            n646 = Not(x=w975) -> (.not. x?=w973:bool)
            n647 = And(x=w973, y=w972) -> (x .and. y?=w974:bool)
            n648 = Compound Arithmetic op=AND(w969, w978, w983, w982, w981) -> (w979:bool)
            n649 = case shown="False" w974 {
              tunnel: w971 -> [_ w993]
              frame False {
                n650 = property on="Turn off BC5" class="Bool (strict)"("DisabledEnum"=T7."Disabled and Grayed Out" ("Disabled")) -> ()  [unwired: 2 in, 2 out]
              }
              frame True {
                w990 = u16 14 items=["NaN", "Kp_Position_Vibro", "Ki_Position_Vibro", "PAR_3", "Sinusfrequenz_preSh", "Zylinder_Move_Button", "PAR_6", "PAR_7", "PAR_8", "PAR_9", "PAR_10", "PAR_11", "PAR_12", "Amplitude_PreSh", "Compass_OFF", "PAR_15", "PAR_16", "SollMoog", "PAR_18", "PAR_19", "PAR_20", "Vibro_Test_Button", "PAR_22", "PAR_23", "PAR_24", "PAR_25", "PAR_26", "PAR_27", "PAR_28", "PAR_29", "PAR_30", "PAR_31", "PAR_32", "Start_Test_Button", "PAR_34", "Programm_counter", "PAR_36", "Circumference_ON_Flag", "PAR_38", "PAR_39", "Pore_Control_Button", "Side_Control_Button", "Axial_Control_Button", "PAR_43", "PAR_44", "PAR_45", "Einfahren_Piston", "PAR_47", "PAR_48", "PAR_49", "PAR_50", "PAR_51", "PAR_52", "PAR_53", "PAR_54", "PAR_55", "PAR_56", "PAR_57", "LinearUpDown_Button", "Linear_Pore_GO", "Linear_Axial_GO", "Linear_Side_GO", "PAR_62", "PAR_63", "PAR_64", "PAR_65", "PAR_66", "PAR_67", "PAR_68", "PAR_69", "Pre_Shearing_Button", "PAR_71", "PAR_72", "PAR_73", "PAR_74", "Circumf_Control_On", "PAR_76", "PAR_77", "PAR_78", "PAR_79", "Modus", "", "", "", "", "", "", "", "", "", "", "", "", "", "", "", "", "", "", "", "", "", "", "", "", "", ""] ("par_enum")
                n651 = local write "Circumference Control"(FALSE ("Umfangsregelung")) -> ()
                n652 = property on="Turn off BC5" class="Bool (strict)"("DisabledEnum"=T7."Enabled" ("Disabled")) -> ()  [unwired: 2 in, 2 out]
                n653 = call "ADwin Set_Par.vi"("Value"=1, "Index"=w990, "Device No."=w993) -> ()  [unwired: 6 in, 3 out]
              }
            }
            n654 = case shown="True" w979 {
              frame False {
              }
              frame True {
                # "not used at the moment"
              }
            }
          }
        }
        "Record Flag" <- "Record Data"
        "Recording" <- "Record Data"
      }
      event "LCT control finish": Value Change {
        (unwired) "Stop control of side pressue, data recording and deactivate LCT-strain-based mode, when LCT control finish \nbutton is pressed "
        n655 = event-data() -> ()  [unwired: 1 in, 6 out]
        n656 = property on="LCT control finish" class="Bool (strict)"() -> ("Value"=w995:bool)  [unwired: 2 in, 2 out]
        n657 = case shown="True" w995 {
          frame False {
          }
          frame True {
            n658 = property on="Regelung Akiv Sidepressure" class="Bool (strict)"("Value"=FALSE ("Regelung Akiv Sidepressure")) -> ()  [unwired: 2 in, 2 out]
            n659 = property on="LCT strain-based control activate" class="Bool (strict)"("Value"=FALSE ("LCT strain-based control activate")) -> ()  [unwired: 2 in, 2 out]
            n660 = property on="Record Data" class="Bool (strict)"("Value"=FALSE ("Record Data")) -> ()  [unwired: 2 in, 2 out]
          }
        }
      }
      event "Reset_left_graph": Value Change {
        n661 = event-data() -> ("NewVal"=w1000:bool)  [unwired: 1 in, 5 out]
        n662 = case shown="True" w1000 {
          selector: w1000 -> [_ w1001]
          frame False {
          }
          frame True {
            "reset_flag" <- w1001
          }
        }
        n663 = property on="Interner Kraftsensor [MPa]" class="XYGraph (strict)"("Value"=cluster{"Y":dbl[], "Y":dbl[]}[] [{"Y"=[0.0], "Y"=[0.0]}] ("Interner Kraftsensor [MPa]")) -> ()  [unwired: 2 in, 2 out]
      }
      event "Notaus": Value Change {
        w1002 = u16 80 items=["NaN", "Kp_Position_Vibro", "Ki_Position_Vibro", "PAR_3", "Sinusfrequenz_preSh", "Zylinder_Move_Button", "PAR_6", "PAR_7", "PAR_8", "PAR_9", "PAR_10", "PAR_11", "PAR_12", "Amplitude_PreSh", "Compass_OFF", "PAR_15", "PAR_16", "SollMoog", "PAR_18", "PAR_19", "PAR_20", "Vibro_Test_Button", "PAR_22", "PAR_23", "PAR_24", "PAR_25", "PAR_26", "PAR_27", "PAR_28", "PAR_29", "PAR_30", "PAR_31", "PAR_32", "Start_Test_Button", "PAR_34", "Programm_counter", "PAR_36", "Circumference_ON_Flag", "PAR_38", "PAR_39", "Pore_Control_Button", "Side_Control_Button", "Axial_Control_Button", "PAR_43", "PAR_44", "PAR_45", "Einfahren_Piston", "PAR_47", "PAR_48", "PAR_49", "PAR_50", "PAR_51", "PAR_52", "PAR_53", "PAR_54", "PAR_55", "PAR_56", "PAR_57", "LinearUpDown_Button", "Linear_Pore_GO", "Linear_Axial_GO", "Linear_Side_GO", "PAR_62", "PAR_63", "PAR_64", "PAR_65", "PAR_66", "PAR_67", "PAR_68", "PAR_69", "Pre_Shearing_Button", "PAR_71", "PAR_72", "PAR_73", "PAR_74", "Circumf_Control_On", "PAR_76", "PAR_77", "PAR_78", "PAR_79", "Modus", "", "", "", "", "", "", "", "", "", "", "", "", "", "", "", "", "", "", "", "", "", "", "", "", "", ""] ("par_enum")
        # "Sets Adiwn State to Cancel all ongoing tasks and quit program"
        n664 = event-data() -> ("NewVal"=w1005:bool)  [unwired: 1 in, 5 out]
        "Notaus Activ" <- w1005
        n665 = call "ADwin Set_Par.vi"("Value"=10, "Index"=w1002, "Device No."=w1003) -> ()  [unwired: 6 in, 3 out]
      }
      event "SET Pump Offsets": Value Change {
        (unwired) "Modification done by zhengyu chen, if measured side, pore and axial pressure is less than default\nvalues, we force them to be default values. "
        n666 = event-data() -> ()  [unwired: 1 in, 6 out]
        n667 = call "ADwin Get_FPar_Block.vi"("count"=i16 80, "startindex"=i16 1, "Device No."=w1009) -> ("Data"=w1028:sgl[])  [unwired: 2 in, 3 out]
        n668 = Decrement(x=T11."SidePressOffset" ("Enum")) -> (x-1=w1031:T11)
        n669 = Decrement(x=T11."AxialPressOffset" ("Enum")) -> (x-1=w1030:T11)
        n670 = Decrement(x=T11."PorePressOffset" ("Enum")) -> (x-1=w1029:T11)
        n671 = Index Array(array=w1028, index=w1031) -> (element=w1024:sgl)
        n672 = Greater?(x=w1024, y="Side Offset Soll") -> (0:w1035:bool)
        n673 = Index Array(array=w1028, index=w1030) -> (element=w1016:sgl)
        n674 = Greater?(x=w1016, y="Axial Offset Soll") -> (0:w1021:bool)
        n675 = Index Array(array=w1028, index=w1029) -> (element=w1013:sgl)
        n676 = Greater?(x=w1013, y="Pore Offset SOLL") -> (0:w1014:bool)
        n677 = case shown="False" w1021 {
          tunnel: w1009 -> [w1044 w1048]
          tunnel: [w1044 w1048] -> w1019
          tunnel: "Axial Offset Soll" -> [w1045 _]
          tunnel: [w1045 w1046] -> w1017
          tunnel: T11."AxialPressOffset" ("Enum") -> [w1043 w1047]
          tunnel: [w1043 w1047] -> w1018
          tunnel: w1016 -> [_ w1046]
          frame False {
          }
          frame True {
          }
        }
        n678 = case shown="False" w1035 {
          tunnel: w1009 -> [w1050 w1054]
          tunnel: [w1050 w1054] -> w1036
          tunnel: "Side Offset Soll" -> [w1051 _]
          tunnel: [w1051 w1052] -> w1022
          tunnel: T11."SidePressOffset" ("Enum") -> [w1049 w1053]
          tunnel: [w1049 w1053] -> w1023
          tunnel: w1024 -> [_ w1052]
          frame False {
          }
          frame True {
          }
        }
        n679 = case shown="False" w1014 {
          tunnel: w1009 -> [w1038 w1042]
          tunnel: [w1038 w1042] -> w1012
          tunnel: "Pore Offset SOLL" -> [w1039 _]
          tunnel: [w1039 w1040] -> w1010
          tunnel: T11."PorePressOffset" ("Enum") -> [w1037 w1041]
          tunnel: [w1037 w1041] -> w1011
          tunnel: w1013 -> [_ w1040]
          frame False {
          }
          frame True {
          }
        }
        n680 = call "ADwin Set_FPar.vi"("Value"=w1022, "Index"=w1023, "Device No."=w1036) -> ()  [unwired: 6 in, 3 out]
        n681 = call "ADwin Set_FPar.vi"("Value"=w1017, "Index"=w1018, "Device No."=w1019) -> ()  [unwired: 6 in, 3 out]
        n682 = call "ADwin Set_FPar.vi"("Value"=w1010, "Index"=w1011, "Device No."=w1012) -> ()  [unwired: 6 in, 3 out]
      }
      event "SET Pump Controls": Value Change {
        n683 = event-data() -> ()  [unwired: 1 in, 6 out]
        n684 = call "ADwin Set_FPar.vi"("Value"="Kpp", "Index"=T11."Kp_Porepress" ("Enum"), "Device No."=w1061) -> ("Device No. out"=w1072:u16)  [unwired: 6 in, 2 out]
        n685 = call "ADwin Set_FPar.vi"("Value"="Kip", "Index"=T11."Ki_Porepress" ("Enum"), "Device No."=w1072) -> ("Device No. out"=w1068:u16)  [unwired: 6 in, 2 out]
        n686 = call "ADwin Set_FPar.vi"("Value"="Kps", "Index"=T11."Kp_Sidepress" ("Enum"), "Device No."=w1068) -> ("Device No. out"=w1069:u16)  [unwired: 6 in, 2 out]
        n687 = call "ADwin Set_FPar.vi"("Value"="Kis", "Index"=T11."Ki_Sidepress" ("Enum"), "Device No."=w1069) -> ("Device No. out"=w1070:u16)  [unwired: 6 in, 2 out]
        n688 = call "ADwin Set_FPar.vi"("Value"="Kpa", "Index"=T11."Kp_Axialpress" ("Enum"), "Device No."=w1070) -> ("Device No. out"=w1071:u16)  [unwired: 6 in, 2 out]
        n689 = call "ADwin Set_FPar.vi"("Value"="Kia", "Index"=T11."Ki_Axialpress" ("Enum"), "Device No."=w1071) -> ()  [unwired: 6 in, 3 out]
      }
      event "Turn off BC5": Value Change {
        n690 = event-data() -> ("NewVal"=w1073:bool)  [unwired: 1 in, 5 out]
        n691 = case shown="True" w1073 {
          tunnel: w1074 -> [_ w1076]
          frame False {
          }
          frame True {
            w1075 = u16 14 items=["NaN", "Kp_Position_Vibro", "Ki_Position_Vibro", "PAR_3", "Sinusfrequenz_preSh", "Zylinder_Move_Button", "PAR_6", "PAR_7", "PAR_8", "PAR_9", "PAR_10", "PAR_11", "PAR_12", "Amplitude_PreSh", "Compass_OFF", "PAR_15", "PAR_16", "SollMoog", "PAR_18", "PAR_19", "PAR_20", "Vibro_Test_Button", "PAR_22", "PAR_23", "PAR_24", "PAR_25", "PAR_26", "PAR_27", "PAR_28", "PAR_29", "PAR_30", "PAR_31", "PAR_32", "Start_Test_Button", "PAR_34", "Programm_counter", "PAR_36", "Circumference_ON_Flag", "PAR_38", "PAR_39", "Pore_Control_Button", "Side_Control_Button", "Axial_Control_Button", "PAR_43", "PAR_44", "PAR_45", "Einfahren_Piston", "PAR_47", "PAR_48", "PAR_49", "PAR_50", "PAR_51", "PAR_52", "PAR_53", "PAR_54", "PAR_55", "PAR_56", "PAR_57", "LinearUpDown_Button", "Linear_Pore_GO", "Linear_Axial_GO", "Linear_Side_GO", "PAR_62", "PAR_63", "PAR_64", "PAR_65", "PAR_66", "PAR_67", "PAR_68", "PAR_69", "Pre_Shearing_Button", "PAR_71", "PAR_72", "PAR_73", "PAR_74", "Circumf_Control_On", "PAR_76", "PAR_77", "PAR_78", "PAR_79", "Modus", "", "", "", "", "", "", "", "", "", "", "", "", "", "", "", "", "", "", "", "", "", "", "", "", "", ""] ("par_enum")
            n692 = call "ADwin Set_Par.vi"("Value"=0, "Index"=w1075, "Device No."=w1076) -> ()  [unwired: 6 in, 3 out]
          }
        }
      }
      event "Circumference Control": Value Change {
        w1078 = u16 75 items=["NaN", "Kp_Position_Vibro", "Ki_Position_Vibro", "PAR_3", "Sinusfrequenz_preSh", "Zylinder_Move_Button", "PAR_6", "PAR_7", "PAR_8", "PAR_9", "PAR_10", "PAR_11", "PAR_12", "Amplitude_PreSh", "Compass_OFF", "PAR_15", "PAR_16", "SollMoog", "PAR_18", "PAR_19", "PAR_20", "Vibro_Test_Button", "PAR_22", "PAR_23", "PAR_24", "PAR_25", "PAR_26", "PAR_27", "PAR_28", "PAR_29", "PAR_30", "PAR_31", "PAR_32", "Start_Test_Button", "PAR_34", "Programm_counter", "PAR_36", "Circumference_ON_Flag", "PAR_38", "PAR_39", "Pore_Control_Button", "Side_Control_Button", "Axial_Control_Button", "PAR_43", "PAR_44", "PAR_45", "Einfahren_Piston", "PAR_47", "PAR_48", "PAR_49", "PAR_50", "PAR_51", "PAR_52", "PAR_53", "PAR_54", "PAR_55", "PAR_56", "PAR_57", "LinearUpDown_Button", "Linear_Pore_GO", "Linear_Axial_GO", "Linear_Side_GO", "PAR_62", "PAR_63", "PAR_64", "PAR_65", "PAR_66", "PAR_67", "PAR_68", "PAR_69", "Pre_Shearing_Button", "PAR_71", "PAR_72", "PAR_73", "PAR_74", "Circumf_Control_On", "PAR_76", "PAR_77", "PAR_78", "PAR_79", "Modus", "", "", "", "", "", "", "", "", "", "", "", "", "", "", "", "", "", "", "", "", "", "", "", "", "", ""] ("par_enum")
        n693 = event-data() -> ("NewVal"=w1080:bool)  [unwired: 1 in, 5 out]
        n694 = Select(t=1 ("Value"), s=w1080, f=0 ("Value")) -> (s? t:f=w1083:i32)
        n695 = case shown="True" w1080 {
          tunnel: w1079 -> [_ w1085]
          frame False {
          }
          frame True {
            w1084 = u16 37 items=["NaN", "Kp_Position_Vibro", "Ki_Position_Vibro", "PAR_3", "Sinusfrequenz_preSh", "Zylinder_Move_Button", "PAR_6", "PAR_7", "PAR_8", "PAR_9", "PAR_10", "PAR_11", "PAR_12", "Amplitude_PreSh", "Compass_OFF", "PAR_15", "PAR_16", "SollMoog", "PAR_18", "PAR_19", "PAR_20", "Vibro_Test_Button", "PAR_22", "PAR_23", "PAR_24", "PAR_25", "PAR_26", "PAR_27", "PAR_28", "PAR_29", "PAR_30", "PAR_31", "PAR_32", "Start_Test_Button", "PAR_34", "Programm_counter", "PAR_36", "Circumference_ON_Flag", "PAR_38", "PAR_39", "Pore_Control_Button", "Side_Control_Button", "Axial_Control_Button", "PAR_43", "PAR_44", "PAR_45", "Einfahren_Piston", "PAR_47", "PAR_48", "PAR_49", "PAR_50", "PAR_51", "PAR_52", "PAR_53", "PAR_54", "PAR_55", "PAR_56", "PAR_57", "LinearUpDown_Button", "Linear_Pore_GO", "Linear_Axial_GO", "Linear_Side_GO", "PAR_62", "PAR_63", "PAR_64", "PAR_65", "PAR_66", "PAR_67", "PAR_68", "PAR_69", "Pre_Shearing_Button", "PAR_71", "PAR_72", "PAR_73", "PAR_74", "Circumf_Control_On", "PAR_76", "PAR_77", "PAR_78", "PAR_79", "Modus", "", "", "", "", "", "", "", "", "", "", "", "", "", "", "", "", "", "", "", "", "", "", "", "", "", ""] ("par_enum")
            n696 = call "ADwin Set_Par.vi"("Value"=1, "Index"=w1084, "Device No."=w1085) -> ()  [unwired: 6 in, 3 out]
          }
        }
        n697 = call "ADwin Set_Par.vi"("Value"=w1083, "Index"=w1078, "Device No."=w1079) -> ()  [unwired: 6 in, 3 out]
      }
      event "Up_Lower": Value Change {
        w1087 = u16 58 items=["NaN", "Kp_Position_Vibro", "Ki_Position_Vibro", "PAR_3", "Sinusfrequenz_preSh", "Zylinder_Move_Button", "PAR_6", "PAR_7", "PAR_8", "PAR_9", "PAR_10", "PAR_11", "PAR_12", "Amplitude_PreSh", "Compass_OFF", "PAR_15", "PAR_16", "SollMoog", "PAR_18", "PAR_19", "PAR_20", "Vibro_Test_Button", "PAR_22", "PAR_23", "PAR_24", "PAR_25", "PAR_26", "PAR_27", "PAR_28", "PAR_29", "PAR_30", "PAR_31", "PAR_32", "Start_Test_Button", "PAR_34", "Programm_counter", "PAR_36", "Circumference_ON_Flag", "PAR_38", "PAR_39", "Pore_Control_Button", "Side_Control_Button", "Axial_Control_Button", "PAR_43", "PAR_44", "PAR_45", "Einfahren_Piston", "PAR_47", "PAR_48", "PAR_49", "PAR_50", "PAR_51", "PAR_52", "PAR_53", "PAR_54", "PAR_55", "PAR_56", "PAR_57", "LinearUpDown_Button", "Linear_Pore_GO", "Linear_Axial_GO", "Linear_Side_GO", "PAR_62", "PAR_63", "PAR_64", "PAR_65", "PAR_66", "PAR_67", "PAR_68", "PAR_69", "Pre_Shearing_Button", "PAR_71", "PAR_72", "PAR_73", "PAR_74", "Circumf_Control_On", "PAR_76", "PAR_77", "PAR_78", "PAR_79", "Modus", "", "", "", "", "", "", "", "", "", "", "", "", "", "", "", "", "", "", "", "", "", "", "", "", "", ""] ("par_enum")
        n698 = event-data() -> ()  [unwired: 1 in, 6 out]
        n699 = Select(t=1 ("Value"), s="Up_Lower", f=0 ("Value")) -> (s? t:f=w1089:i32)
        n700 = call "ADwin Set_Par.vi"("Value"=w1089, "Index"=w1087, "Device No."=w1088) -> ()  [unwired: 6 in, 3 out]
      }
      event "Go - Porendruck": Value Change {
        n701 = event-data() -> ()  [unwired: 1 in, 6 out]
        n702 = flat-sequence {
          tunnel: w1095 -> [w1096]
          tunnel: [w1104] -> w1094
          tunnel: [w1098] -> w1093
          tunnel: w1094 -> [w1121]
          tunnel: w1093 -> [w1126]
          frame #0 {
            w1100 = u16 58 items=["NaN", "Kp_Position_Vibro", "Ki_Position_Vibro", "PAR_3", "Sinusfrequenz_preSh", "Zylinder_Move_Button", "PAR_6", "PAR_7", "PAR_8", "PAR_9", "PAR_10", "PAR_11", "PAR_12", "Amplitude_PreSh", "Compass_OFF", "PAR_15", "PAR_16", "SollMoog", "PAR_18", "PAR_19", "PAR_20", "Vibro_Test_Button", "PAR_22", "PAR_23", "PAR_24", "PAR_25", "PAR_26", "PAR_27", "PAR_28", "PAR_29", "PAR_30", "PAR_31", "PAR_32", "Start_Test_Button", "PAR_34", "Programm_counter", "PAR_36", "Circumference_ON_Flag", "PAR_38", "PAR_39", "Pore_Control_Button", "Side_Control_Button", "Axial_Control_Button", "PAR_43", "PAR_44", "PAR_45", "Einfahren_Piston", "PAR_47", "PAR_48", "PAR_49", "PAR_50", "PAR_51", "PAR_52", "PAR_53", "PAR_54", "PAR_55", "PAR_56", "PAR_57", "LinearUpDown_Button", "Linear_Pore_GO", "Linear_Axial_GO", "Linear_Side_GO", "PAR_62", "PAR_63", "PAR_64", "PAR_65", "PAR_66", "PAR_67", "PAR_68", "PAR_69", "Pre_Shearing_Button", "PAR_71", "PAR_72", "PAR_73", "PAR_74", "Circumf_Control_On", "PAR_76", "PAR_77", "PAR_78", "PAR_79", "Modus", "", "", "", "", "", "", "", "", "", "", "", "", "", "", "", "", "", "", "", "", "", "", "", "", "", ""] ("par_enum")
            # "Pro Minute"
            n703 = local read "GO All Pressure"() -> (w1113:bool)
            n704 = local read "Velocity Linear"() -> (w1105:dbl)
            n705 = local read "Delta Pore"() -> (w1117:dbl)
            n706 = local read "Up_Lower"() -> (w1097:bool)
            n707 = Or(x="Go - Porendruck", y=w1113) -> (x .or. y?=w1114:bool)
            n708 = Multiply(x=5000.0 ("y"), y=60.0) -> (x*y=w1111:dbl)
            n709 = Greater?(x=w1117, y=0.0) -> (0:w1115:bool)
            n710 = Divide(x=5.4613, y=w1111) -> (x/y=w1112:dbl)
            n711 = And(x=w1114, y=w1115) -> (x .and. y?=w1104:bool)
            n712 = case shown="True" w1104 {
              selector: w1104 -> [_ w1119]
              frame False {
              }
              frame True {
                n713 = local write "Regelung Akiv Porepress"(w1119) -> ()
              }
            }
            n714 = Multiply(x=w1105, y=w1112) -> (x*y=w1108:dbl)
            n715 = local write "Go - Porendruck"(w1104) -> ()
            n716 = Select(t=1 ("Value"), s=w1097, f=0 ("Value")) -> (s? t:f=w1101:i32)
            n717 = call "ADwin Set_Par.vi"("Value"=w1101, "Index"=w1100, "Device No."=w1096) -> ("Device No. out"=w1099:u16)  [unwired: 6 in, 2 out]
            n718 = call "ADwin Set_FPar.vi"("Value"=w1108, "Index"=T11."PaProMin" ("Enum"), "Device No."=w1099) -> ("Device No. out"=w1098:u16)  [unwired: 6 in, 2 out]
          }
          frame #1 {
            w1125 = u16 40 items=["NaN", "Kp_Position_Vibro", "Ki_Position_Vibro", "PAR_3", "Sinusfrequenz_preSh", "Zylinder_Move_Button", "PAR_6", "PAR_7", "PAR_8", "PAR_9", "PAR_10", "PAR_11", "PAR_12", "Amplitude_PreSh", "Compass_OFF", "PAR_15", "PAR_16", "SollMoog", "PAR_18", "PAR_19", "PAR_20", "Vibro_Test_Button", "PAR_22", "PAR_23", "PAR_24", "PAR_25", "PAR_26", "PAR_27", "PAR_28", "PAR_29", "PAR_30", "PAR_31", "PAR_32", "Start_Test_Button", "PAR_34", "Programm_counter", "PAR_36", "Circumference_ON_Flag", "PAR_38", "PAR_39", "Pore_Control_Button", "Side_Control_Button", "Axial_Control_Button", "PAR_43", "PAR_44", "PAR_45", "Einfahren_Piston", "PAR_47", "PAR_48", "PAR_49", "PAR_50", "PAR_51", "PAR_52", "PAR_53", "PAR_54", "PAR_55", "PAR_56", "PAR_57", "LinearUpDown_Button", "Linear_Pore_GO", "Linear_Axial_GO", "Linear_Side_GO", "PAR_62", "PAR_63", "PAR_64", "PAR_65", "PAR_66", "PAR_67", "PAR_68", "PAR_69", "Pre_Shearing_Button", "PAR_71", "PAR_72", "PAR_73", "PAR_74", "Circumf_Control_On", "PAR_76", "PAR_77", "PAR_78", "PAR_79", "Modus", "", "", "", "", "", "", "", "", "", "", "", "", "", "", "", "", "", "", "", "", "", "", "", "", "", ""] ("par_enum")
            w1130 = u16 59 items=["NaN", "Kp_Position_Vibro", "Ki_Position_Vibro", "PAR_3", "Sinusfrequenz_preSh", "Zylinder_Move_Button", "PAR_6", "PAR_7", "PAR_8", "PAR_9", "PAR_10", "PAR_11", "PAR_12", "Amplitude_PreSh", "Compass_OFF", "PAR_15", "PAR_16", "SollMoog", "PAR_18", "PAR_19", "PAR_20", "Vibro_Test_Button", "PAR_22", "PAR_23", "PAR_24", "PAR_25", "PAR_26", "PAR_27", "PAR_28", "PAR_29", "PAR_30", "PAR_31", "PAR_32", "Start_Test_Button", "PAR_34", "Programm_counter", "PAR_36", "Circumference_ON_Flag", "PAR_38", "PAR_39", "Pore_Control_Button", "Side_Control_Button", "Axial_Control_Button", "PAR_43", "PAR_44", "PAR_45", "Einfahren_Piston", "PAR_47", "PAR_48", "PAR_49", "PAR_50", "PAR_51", "PAR_52", "PAR_53", "PAR_54", "PAR_55", "PAR_56", "PAR_57", "LinearUpDown_Button", "Linear_Pore_GO", "Linear_Axial_GO", "Linear_Side_GO", "PAR_62", "PAR_63", "PAR_64", "PAR_65", "PAR_66", "PAR_67", "PAR_68", "PAR_69", "Pre_Shearing_Button", "PAR_71", "PAR_72", "PAR_73", "PAR_74", "Circumf_Control_On", "PAR_76", "PAR_77", "PAR_78", "PAR_79", "Modus", "", "", "", "", "", "", "", "", "", "", "", "", "", "", "", "", "", "", "", "", "", "", "", "", "", ""] ("par_enum")
            n719 = Select(t=1 ("Value"), s=w1121, f=0 ("Value")) -> (s? t:f=w1129:i32)
            n720 = Select(t=1 ("Value"), s=w1121, f=0 ("Value")) -> (s? t:f=w1124:i32)
            n721 = call "ADwin Set_Par.vi"("Value"=w1129, "Index"=w1130, "Device No."=w1126) -> ("Device No. out"=w1120:u16)  [unwired: 6 in, 2 out]
            n722 = call "ADwin Set_Par.vi"("Value"=w1124, "Index"=w1125, "Device No."=w1120) -> ()  [unwired: 6 in, 3 out]
          }
        }
      }
      event "GO All Pressure": Value Change {
        n723 = event-data() -> ()  [unwired: 1 in, 6 out]
        n724 = case shown="True" "GO All Pressure" {
          selector: "GO All Pressure" -> [_ w1132]
          frame False {
          }
          frame True {
            n725 = flat-sequence {
              tunnel: w1132 -> [_]
              frame #0 {
                n726 = local read "Delta Seiten"() -> (w1138:dbl)
                n727 = local read "Delta Pore"() -> (w1141:dbl)
                n728 = local read "Delta Axial"() -> (w1135:dbl)
                n729 = Greater?(x=w1141, y=0.0) -> (0:w1140:bool)
                n730 = Greater?(x=w1138, y=0.0) -> (0:w1137:bool)
                n731 = Greater?(x=w1135, y=0.0) -> (0:w1134:bool)
                n732 = case shown="True" w1140 {
                  selector: w1140 -> [_ w1144]
                  frame False {
                  }
                  frame True {
                    n733 = property on="Go - Porendruck" class="Bool (strict)"("Val(Sgnl)"=w1144) -> ()  [unwired: 2 in, 2 out]
                  }
                }
                n734 = case shown="True" w1137 {
                  selector: w1137 -> [_ w1143]
                  frame False {
                  }
                  frame True {
                    n735 = property on="Go - Seitendruck" class="Bool (strict)"("Val(Sgnl)"=w1143) -> ()  [unwired: 2 in, 2 out]
                  }
                }
                n736 = case shown="True" w1134 {
                  selector: w1134 -> [_ w1142]
                  frame False {
                  }
                  frame True {
                    n737 = property on="Go - Axialdruck" class="Bool (strict)"("Val(Sgnl)"=w1142) -> ()  [unwired: 2 in, 2 out]
                  }
                }
              }
              frame #1 {
                n738 = local write "GO All Pressure"(FALSE ("GO All Pressure")) -> ()
              }
            }
          }
        }
      }
      event "Go - Axialdruck": Value Change {
        n739 = event-data() -> ()  [unwired: 1 in, 6 out]
        n740 = flat-sequence {
          tunnel: w1148 -> [w1149]
          tunnel: [w1157] -> w1147
          tunnel: [w1150] -> w1146
          tunnel: w1147 -> [w1174]
          tunnel: w1146 -> [w1179]
          frame #0 {
            w1153 = u16 58 items=["NaN", "Kp_Position_Vibro", "Ki_Position_Vibro", "PAR_3", "Sinusfrequenz_preSh", "Zylinder_Move_Button", "PAR_6", "PAR_7", "PAR_8", "PAR_9", "PAR_10", "PAR_11", "PAR_12", "Amplitude_PreSh", "Compass_OFF", "PAR_15", "PAR_16", "SollMoog", "PAR_18", "PAR_19", "PAR_20", "Vibro_Test_Button", "PAR_22", "PAR_23", "PAR_24", "PAR_25", "PAR_26", "PAR_27", "PAR_28", "PAR_29", "PAR_30", "PAR_31", "PAR_32", "Start_Test_Button", "PAR_34", "Programm_counter", "PAR_36", "Circumference_ON_Flag", "PAR_38", "PAR_39", "Pore_Control_Button", "Side_Control_Button", "Axial_Control_Button", "PAR_43", "PAR_44", "PAR_45", "Einfahren_Piston", "PAR_47", "PAR_48", "PAR_49", "PAR_50", "PAR_51", "PAR_52", "PAR_53", "PAR_54", "PAR_55", "PAR_56", "PAR_57", "LinearUpDown_Button", "Linear_Pore_GO", "Linear_Axial_GO", "Linear_Side_GO", "PAR_62", "PAR_63", "PAR_64", "PAR_65", "PAR_66", "PAR_67", "PAR_68", "PAR_69", "Pre_Shearing_Button", "PAR_71", "PAR_72", "PAR_73", "PAR_74", "Circumf_Control_On", "PAR_76", "PAR_77", "PAR_78", "PAR_79", "Modus", "", "", "", "", "", "", "", "", "", "", "", "", "", "", "", "", "", "", "", "", "", "", "", "", "", ""] ("par_enum")
            # "Entspricht 1 kPa"
            # "5000 Hz Programm"
            # "Pro Minute"
            n741 = local read "GO All Pressure"() -> (w1171:bool)
            n742 = local read "Delta Axial"() -> (w1168:dbl)
            n743 = Or(x="Go - Axialdruck", y=w1171) -> (x .or. y?=w1166:bool)
            n744 = Greater?(x=w1168, y=0.0) -> (0:w1167:bool)
            n745 = And(x=w1166, y=w1167) -> (x .and. y?=w1157:bool)
            n746 = local write "Go - Axialdruck"(w1157) -> ()
            n747 = Multiply(x=5000.0 ("y"), y=60.0) -> (x*y=w1164:dbl)
            n748 = case shown="True" w1157 {
              selector: w1157 -> [_ w1172]
              frame False {
              }
              frame True {
                n749 = local write "Regelung Akiv Axial"(w1172) -> ()
              }
            }
            n750 = Divide(x=5.4613, y=w1164) -> (x/y=w1165:dbl)
            n751 = local read "Up_Lower"() -> (w1151:bool)
            n752 = Multiply(x="Velocity Linear", y=w1165) -> (x*y=w1160:dbl)
            n753 = Select(t=1 ("Value"), s=w1151, f=0 ("Value")) -> (s? t:f=w1154:i32)
            n754 = call "ADwin Set_Par.vi"("Value"=w1154, "Index"=w1153, "Device No."=w1149) -> ("Device No. out"=w1152:u16)  [unwired: 6 in, 2 out]
            n755 = call "ADwin Set_FPar.vi"("Value"=w1160, "Index"=T11."PaProMin" ("Enum"), "Device No."=w1152) -> ("Device No. out"=w1150:u16)  [unwired: 6 in, 2 out]
          }
          frame #1 {
            w1178 = u16 42 items=["NaN", "Kp_Position_Vibro", "Ki_Position_Vibro", "PAR_3", "Sinusfrequenz_preSh", "Zylinder_Move_Button", "PAR_6", "PAR_7", "PAR_8", "PAR_9", "PAR_10", "PAR_11", "PAR_12", "Amplitude_PreSh", "Compass_OFF", "PAR_15", "PAR_16", "SollMoog", "PAR_18", "PAR_19", "PAR_20", "Vibro_Test_Button", "PAR_22", "PAR_23", "PAR_24", "PAR_25", "PAR_26", "PAR_27", "PAR_28", "PAR_29", "PAR_30", "PAR_31", "PAR_32", "Start_Test_Button", "PAR_34", "Programm_counter", "PAR_36", "Circumference_ON_Flag", "PAR_38", "PAR_39", "Pore_Control_Button", "Side_Control_Button", "Axial_Control_Button", "PAR_43", "PAR_44", "PAR_45", "Einfahren_Piston", "PAR_47", "PAR_48", "PAR_49", "PAR_50", "PAR_51", "PAR_52", "PAR_53", "PAR_54", "PAR_55", "PAR_56", "PAR_57", "LinearUpDown_Button", "Linear_Pore_GO", "Linear_Axial_GO", "Linear_Side_GO", "PAR_62", "PAR_63", "PAR_64", "PAR_65", "PAR_66", "PAR_67", "PAR_68", "PAR_69", "Pre_Shearing_Button", "PAR_71", "PAR_72", "PAR_73", "PAR_74", "Circumf_Control_On", "PAR_76", "PAR_77", "PAR_78", "PAR_79", "Modus", "", "", "", "", "", "", "", "", "", "", "", "", "", "", "", "", "", "", "", "", "", "", "", "", "", ""] ("par_enum")
            w1183 = u16 60 items=["NaN", "Kp_Position_Vibro", "Ki_Position_Vibro", "PAR_3", "Sinusfrequenz_preSh", "Zylinder_Move_Button", "PAR_6", "PAR_7", "PAR_8", "PAR_9", "PAR_10", "PAR_11", "PAR_12", "Amplitude_PreSh", "Compass_OFF", "PAR_15", "PAR_16", "SollMoog", "PAR_18", "PAR_19", "PAR_20", "Vibro_Test_Button", "PAR_22", "PAR_23", "PAR_24", "PAR_25", "PAR_26", "PAR_27", "PAR_28", "PAR_29", "PAR_30", "PAR_31", "PAR_32", "Start_Test_Button", "PAR_34", "Programm_counter", "PAR_36", "Circumference_ON_Flag", "PAR_38", "PAR_39", "Pore_Control_Button", "Side_Control_Button", "Axial_Control_Button", "PAR_43", "PAR_44", "PAR_45", "Einfahren_Piston", "PAR_47", "PAR_48", "PAR_49", "PAR_50", "PAR_51", "PAR_52", "PAR_53", "PAR_54", "PAR_55", "PAR_56", "PAR_57", "LinearUpDown_Button", "Linear_Pore_GO", "Linear_Axial_GO", "Linear_Side_GO", "PAR_62", "PAR_63", "PAR_64", "PAR_65", "PAR_66", "PAR_67", "PAR_68", "PAR_69", "Pre_Shearing_Button", "PAR_71", "PAR_72", "PAR_73", "PAR_74", "Circumf_Control_On", "PAR_76", "PAR_77", "PAR_78", "PAR_79", "Modus", "", "", "", "", "", "", "", "", "", "", "", "", "", "", "", "", "", "", "", "", "", "", "", "", "", ""] ("par_enum")
            n756 = Select(t=1 ("Value"), s=w1174, f=0 ("Value")) -> (s? t:f=w1182:i32)
            n757 = Select(t=1 ("Value"), s=w1174, f=0 ("Value")) -> (s? t:f=w1177:i32)
            n758 = call "ADwin Set_Par.vi"("Value"=w1182, "Index"=w1183, "Device No."=w1179) -> ("Device No. out"=w1175:u16)  [unwired: 6 in, 2 out]
            n759 = call "ADwin Set_Par.vi"("Value"=w1177, "Index"=w1178, "Device No."=w1175) -> ()  [unwired: 6 in, 3 out]
          }
        }
      }
      event "Velocity Linear": Value Change {
        # "5000 Hz Programm"
        # "Pro Minute"
        n760 = event-data() -> ("NewVal"=w1185:dbl)  [unwired: 1 in, 5 out]
        n761 = Multiply(x=5000.0 ("y"), y=60.0) -> (x*y=w1191:dbl)
        n762 = Divide(x=5.4613, y=w1191) -> (x/y=w1192:dbl)
        n763 = Multiply(x=w1185, y=w1192) -> (x*y=w1188:dbl)
        n764 = call "ADwin Set_FPar.vi"("Value"=w1188, "Index"=T11."PaProMin" ("Enum"), "Device No."=w1184) -> ()  [unwired: 6 in, 3 out]
      }
      event "Go - Seitendruck": Value Change {
        n765 = event-data() -> ()  [unwired: 1 in, 6 out]
        n766 = flat-sequence {
          tunnel: w1195 -> [w1197]
          tunnel: [w1199] -> w1194
          tunnel: [w1196] -> w1193
          tunnel: w1194 -> [w1226]
          tunnel: w1193 -> [w1221]
          frame #0 {
            w1201 = u16 58 items=["NaN", "Kp_Position_Vibro", "Ki_Position_Vibro", "PAR_3", "Sinusfrequenz_preSh", "Zylinder_Move_Button", "PAR_6", "PAR_7", "PAR_8", "PAR_9", "PAR_10", "PAR_11", "PAR_12", "Amplitude_PreSh", "Compass_OFF", "PAR_15", "PAR_16", "SollMoog", "PAR_18", "PAR_19", "PAR_20", "Vibro_Test_Button", "PAR_22", "PAR_23", "PAR_24", "PAR_25", "PAR_26", "PAR_27", "PAR_28", "PAR_29", "PAR_30", "PAR_31", "PAR_32", "Start_Test_Button", "PAR_34", "Programm_counter", "PAR_36", "Circumference_ON_Flag", "PAR_38", "PAR_39", "Pore_Control_Button", "Side_Control_Button", "Axial_Control_Button", "PAR_43", "PAR_44", "PAR_45", "Einfahren_Piston", "PAR_47", "PAR_48", "PAR_49", "PAR_50", "PAR_51", "PAR_52", "PAR_53", "PAR_54", "PAR_55", "PAR_56", "PAR_57", "LinearUpDown_Button", "Linear_Pore_GO", "Linear_Axial_GO", "Linear_Side_GO", "PAR_62", "PAR_63", "PAR_64", "PAR_65", "PAR_66", "PAR_67", "PAR_68", "PAR_69", "Pre_Shearing_Button", "PAR_71", "PAR_72", "PAR_73", "PAR_74", "Circumf_Control_On", "PAR_76", "PAR_77", "PAR_78", "PAR_79", "Modus", "", "", "", "", "", "", "", "", "", "", "", "", "", "", "", "", "", "", "", "", "", "", "", "", "", ""] ("par_enum")
            # "5000 Hz Programm"
            # "Pro Minute"
            n767 = local read "GO All Pressure"() -> (w1213:bool)
            n768 = local read "Delta Seiten"() -> (w1215:dbl)
            n769 = Or(x="Go - Seitendruck", y=w1213) -> (x .or. y?=w1217:bool)
            n770 = local read "Velocity Linear"() -> (w1205:dbl)
            n771 = Greater?(x=w1215, y=0.0) -> (0:w1214:bool)
            n772 = And(x=w1217, y=w1214) -> (x .and. y?=w1196:bool)
            n773 = local write "Go - Seitendruck"(w1196) -> ()
            n774 = case shown="True" w1196 {
              selector: w1196 -> [_ w1219]
              frame False {
              }
              frame True {
                n775 = local write "Regelung Akiv Sidepressure"(w1219) -> ()
              }
            }
            n776 = Multiply(x=5000.0 ("y"), y=60.0) -> (x*y=w1211:dbl)
            n777 = Divide(x=5.4613, y=w1211) -> (x/y=w1212:dbl)
            n778 = local read "Up_Lower"() -> (w1198:bool)
            n779 = Multiply(x=w1205, y=w1212) -> (x*y=w1208:dbl)
            n780 = Select(t=1 ("Value"), s=w1198, f=0 ("Value")) -> (s? t:f=w1202:i32)
            n781 = call "ADwin Set_Par.vi"("Value"=w1202, "Index"=w1201, "Device No."=w1197) -> ("Device No. out"=w1200:u16)  [unwired: 6 in, 2 out]
            n782 = call "ADwin Set_FPar.vi"("Value"=w1208, "Index"=T11."PaProMin" ("Enum"), "Device No."=w1200) -> ("Device No. out"=w1199:u16)  [unwired: 6 in, 2 out]
          }
          frame #1 {
            w1223 = u16 41 items=["NaN", "Kp_Position_Vibro", "Ki_Position_Vibro", "PAR_3", "Sinusfrequenz_preSh", "Zylinder_Move_Button", "PAR_6", "PAR_7", "PAR_8", "PAR_9", "PAR_10", "PAR_11", "PAR_12", "Amplitude_PreSh", "Compass_OFF", "PAR_15", "PAR_16", "SollMoog", "PAR_18", "PAR_19", "PAR_20", "Vibro_Test_Button", "PAR_22", "PAR_23", "PAR_24", "PAR_25", "PAR_26", "PAR_27", "PAR_28", "PAR_29", "PAR_30", "PAR_31", "PAR_32", "Start_Test_Button", "PAR_34", "Programm_counter", "PAR_36", "Circumference_ON_Flag", "PAR_38", "PAR_39", "Pore_Control_Button", "Side_Control_Button", "Axial_Control_Button", "PAR_43", "PAR_44", "PAR_45", "Einfahren_Piston", "PAR_47", "PAR_48", "PAR_49", "PAR_50", "PAR_51", "PAR_52", "PAR_53", "PAR_54", "PAR_55", "PAR_56", "PAR_57", "LinearUpDown_Button", "Linear_Pore_GO", "Linear_Axial_GO", "Linear_Side_GO", "PAR_62", "PAR_63", "PAR_64", "PAR_65", "PAR_66", "PAR_67", "PAR_68", "PAR_69", "Pre_Shearing_Button", "PAR_71", "PAR_72", "PAR_73", "PAR_74", "Circumf_Control_On", "PAR_76", "PAR_77", "PAR_78", "PAR_79", "Modus", "", "", "", "", "", "", "", "", "", "", "", "", "", "", "", "", "", "", "", "", "", "", "", "", "", ""] ("par_enum")
            w1230 = u16 61 items=["NaN", "Kp_Position_Vibro", "Ki_Position_Vibro", "PAR_3", "Sinusfrequenz_preSh", "Zylinder_Move_Button", "PAR_6", "PAR_7", "PAR_8", "PAR_9", "PAR_10", "PAR_11", "PAR_12", "Amplitude_PreSh", "Compass_OFF", "PAR_15", "PAR_16", "SollMoog", "PAR_18", "PAR_19", "PAR_20", "Vibro_Test_Button", "PAR_22", "PAR_23", "PAR_24", "PAR_25", "PAR_26", "PAR_27", "PAR_28", "PAR_29", "PAR_30", "PAR_31", "PAR_32", "Start_Test_Button", "PAR_34", "Programm_counter", "PAR_36", "Circumference_ON_Flag", "PAR_38", "PAR_39", "Pore_Control_Button", "Side_Control_Button", "Axial_Control_Button", "PAR_43", "PAR_44", "PAR_45", "Einfahren_Piston", "PAR_47", "PAR_48", "PAR_49", "PAR_50", "PAR_51", "PAR_52", "PAR_53", "PAR_54", "PAR_55", "PAR_56", "PAR_57", "LinearUpDown_Button", "Linear_Pore_GO", "Linear_Axial_GO", "Linear_Side_GO", "PAR_62", "PAR_63", "PAR_64", "PAR_65", "PAR_66", "PAR_67", "PAR_68", "PAR_69", "Pre_Shearing_Button", "PAR_71", "PAR_72", "PAR_73", "PAR_74", "Circumf_Control_On", "PAR_76", "PAR_77", "PAR_78", "PAR_79", "Modus", "", "", "", "", "", "", "", "", "", "", "", "", "", "", "", "", "", "", "", "", "", "", "", "", "", ""] ("par_enum")
            n783 = Select(t=1 ("Value"), s=w1221, f=0 ("Value")) -> (s? t:f=w1228:i32)
            n784 = Select(t=1 ("Value"), s=w1221, f=0 ("Value")) -> (s? t:f=w1225:i32)
            n785 = call "ADwin Set_Par.vi"("Value"=w1228, "Index"=w1230, "Device No."=w1226) -> ("Device No. out"=w1222:u16)  [unwired: 6 in, 2 out]
            n786 = call "ADwin Set_Par.vi"("Value"=w1225, "Index"=w1223, "Device No."=w1222) -> ()  [unwired: 6 in, 3 out]
          }
        }
      }
      event "Set auto file name": Value Change {
        n787 = event-data() -> ()  [unwired: 1 in, 6 out]
        n788 = local read "IS P-Value"() -> (w1263:i32)
        n789 = local read "IS I-Value"() -> (w1257:i32)
        n790 = local read "Feeding IS"() -> (w1254:dbl)
        n791 = local read "Amplitude IS"() -> (w1249:dbl)
        n792 = local read "Frequency IS"() -> (w1245:dbl)
        n793 = Number To Decimal String(number=w1249) -> (decimal integer string=w1251:string)  [unwired: 1 in]
        n794 = Number To Decimal String(number=w1245) -> (decimal integer string=w1247:string)  [unwired: 1 in]
        n795 = Number To Decimal String(number=w1254) -> (decimal integer string=w1255:string)  [unwired: 1 in]
        n796 = Number To Decimal String(number=w1257) -> (decimal integer string=w1259:string)  [unwired: 1 in]
        n797 = Number To Decimal String(number=w1263) -> (decimal integer string=w1262:string)  [unwired: 1 in]
        n798 = Concatenate Strings("_A" ("string"), w1251) -> (w1248:string)
        n799 = Concatenate Strings("_F" ("string"), w1247) -> (w1244:string)
        n800 = Concatenate Strings("_V" ("string"), w1255) -> (w1252:string)
        n801 = Concatenate Strings("_I" ("string"), w1259) -> (w1256:string)
        n802 = Concatenate Strings("P" ("string"), w1262) -> (w1260:string)
        n803 = Format Date/Time String(time format string (%c)="%d_%m_%y_%H_%M_") -> (date/time string=w1264:string)  [unwired: 2 in]
        n804 = Current VI's Path() -> (path=w1234:path)
        n805 = Strip Path(path=w1234) -> (stripped path=w1233:path)  [unwired: 1 out]
        n806 = Concatenate Strings(w1264, w1260, w1256, w1252, w1248, w1244, ".csv" ("String")) -> (w1240:string)
        n807 = Build Path(base path=w1233, name or relative path=w1231) -> (appended path=w1235:path)
        n808 = String To Path(string=w1240) -> (path=w1241:path)
        n809 = Build Path(base path=w1239, name or relative path=w1241) -> (appended path=w1238:path)
        n810 = call-poly <vilib>:"Read From Spreadsheet File.vi"("delimiter (\\t)"=";" ("delimiter (\\t)"), "file path (dialog if empty)"=w1235) -> ("first row"=w1232:string[])  [unwired: 5 in, 4 out]
        n811 = local write "Path Logging"(w1238) -> ()
        n812 = call-poly <vilib>:"Write To Spreadsheet File.vi"("delimiter (\\t)"=";" ("delimiter (\\t)"), "1D data"=w1232, "file path (dialog if empty)"=w1238) -> ()  [unwired: 5 in, 1 out]
      }
      event "SET P/I Value": Value Change {
        w1266 = u16 1 items=["NaN", "Kp_Position_Vibro", "Ki_Position_Vibro", "PAR_3", "Sinusfrequenz_preSh", "Zylinder_Move_Button", "PAR_6", "PAR_7", "PAR_8", "PAR_9", "PAR_10", "PAR_11", "PAR_12", "Amplitude_PreSh", "Compass_OFF", "PAR_15", "PAR_16", "SollMoog", "PAR_18", "PAR_19", "PAR_20", "Vibro_Test_Button", "PAR_22", "PAR_23", "PAR_24", "PAR_25", "PAR_26", "PAR_27", "PAR_28", "PAR_29", "PAR_30", "PAR_31", "PAR_32", "Start_Test_Button", "PAR_34", "Programm_counter", "PAR_36", "Circumference_ON_Flag", "PAR_38", "PAR_39", "Pore_Control_Button", "Side_Control_Button", "Axial_Control_Button", "PAR_43", "PAR_44", "PAR_45", "Einfahren_Piston", "PAR_47", "PAR_48", "PAR_49", "PAR_50", "PAR_51", "PAR_52", "PAR_53", "PAR_54", "PAR_55", "PAR_56", "PAR_57", "LinearUpDown_Button", "Linear_Pore_GO", "Linear_Axial_GO", "Linear_Side_GO", "PAR_62", "PAR_63", "PAR_64", "PAR_65", "PAR_66", "PAR_67", "PAR_68", "PAR_69", "Pre_Shearing_Button", "PAR_71", "PAR_72", "PAR_73", "PAR_74", "Circumf_Control_On", "PAR_76", "PAR_77", "PAR_78", "PAR_79", "Modus", "", "", "", "", "", "", "", "", "", "", "", "", "", "", "", "", "", "", "", "", "", "", "", "", "", ""] ("par_enum")
        w1265 = u16 2 items=["NaN", "Kp_Position_Vibro", "Ki_Position_Vibro", "PAR_3", "Sinusfrequenz_preSh", "Zylinder_Move_Button", "PAR_6", "PAR_7", "PAR_8", "PAR_9", "PAR_10", "PAR_11", "PAR_12", "Amplitude_PreSh", "Compass_OFF", "PAR_15", "PAR_16", "SollMoog", "PAR_18", "PAR_19", "PAR_20", "Vibro_Test_Button", "PAR_22", "PAR_23", "PAR_24", "PAR_25", "PAR_26", "PAR_27", "PAR_28", "PAR_29", "PAR_30", "PAR_31", "PAR_32", "Start_Test_Button", "PAR_34", "Programm_counter", "PAR_36", "Circumference_ON_Flag", "PAR_38", "PAR_39", "Pore_Control_Button", "Side_Control_Button", "Axial_Control_Button", "PAR_43", "PAR_44", "PAR_45", "Einfahren_Piston", "PAR_47", "PAR_48", "PAR_49", "PAR_50", "PAR_51", "PAR_52", "PAR_53", "PAR_54", "PAR_55", "PAR_56", "PAR_57", "LinearUpDown_Button", "Linear_Pore_GO", "Linear_Axial_GO", "Linear_Side_GO", "PAR_62", "PAR_63", "PAR_64", "PAR_65", "PAR_66", "PAR_67", "PAR_68", "PAR_69", "Pre_Shearing_Button", "PAR_71", "PAR_72", "PAR_73", "PAR_74", "Circumf_Control_On", "PAR_76", "PAR_77", "PAR_78", "PAR_79", "Modus", "", "", "", "", "", "", "", "", "", "", "", "", "", "", "", "", "", "", "", "", "", "", "", "", "", ""] ("par_enum")
        n813 = event-data() -> ()  [unwired: 1 in, 6 out]
        n814 = call "ADwin Set_Par.vi"("Value"="Soll P-Value", "Index"=w1266, "Device No."=w1269) -> ("Device No. out"=w1267:u16)  [unwired: 6 in, 2 out]
        n815 = call "ADwin Set_Par.vi"("Value"="Soll I-Value", "Index"=w1265, "Device No."=w1267) -> ()  [unwired: 6 in, 3 out]
      }
      event "Set New Path": Value Change {
        n816 = event-data() -> ("NewVal"=w1274:bool)  [unwired: 1 in, 5 out]
        n817 = String Length(string="New Path") -> (length=w1277:i32)
        n818 = Greater?(x=w1277, y=0) -> (0:w1275:bool)
        n819 = And(x=w1274, y=w1275) -> (x .and. y?=w1273:bool)
        n820 = case shown="True" w1273 {
          tunnel: w1278 -> [_ w1290]
          tunnel: "New Path" -> [_ w1289]
          tunnel: w1271 -> [_ w1281]
          frame False {
          }
          frame True {
            n821 = Current VI's Path() -> (path=w1286:path)
            n822 = Format Date/Time String(time format string (%c)="%d_%m_%y_%H_%M_") -> (date/time string=w1279:string)  [unwired: 2 in]
            n823 = Strip Path(path=w1286) -> (stripped path=w1285:path)  [unwired: 1 out]
            n824 = Build Path(base path=w1285, name or relative path=w1281) -> (appended path=w1287:path)
            n825 = Concatenate Strings(w1279, w1289, ".csv" ("String")) -> (w1291:string)
            n826 = Build Path(base path=w1290, name or relative path=w1291) -> (appended path=w1282:path)
            n827 = call-poly <vilib>:"Read From Spreadsheet File.vi"("delimiter (\\t)"=";" ("delimiter (\\t)"), "file path (dialog if empty)"=w1287) -> ("first row"=w1283:string[])  [unwired: 5 in, 4 out]
            n828 = call-poly <vilib>:"Write To Spreadsheet File.vi"("delimiter (\\t)"=";" ("delimiter (\\t)"), "1D data"=w1283, "file path (dialog if empty)"=w1282) -> ()  [unwired: 5 in, 1 out]
            n829 = local write "Path Logging"(w1282) -> ()
          }
        }
      }
      event "Activate Manuel Control": Value Change {
        n830 = event-data() -> ("NewVal"=w1293:bool)  [unwired: 1 in, 5 out]
        "Manuel Control" <- w1293
        n831 = case shown="False" w1293 {
          tunnel: w1296 -> [_ w1300]
          frame False {
          }
          frame True {
            w1297 = u16 80 items=["NaN", "Kp_Position_Vibro", "Ki_Position_Vibro", "PAR_3", "Sinusfrequenz_preSh", "Zylinder_Move_Button", "PAR_6", "PAR_7", "PAR_8", "PAR_9", "PAR_10", "PAR_11", "PAR_12", "Amplitude_PreSh", "Compass_OFF", "PAR_15", "PAR_16", "SollMoog", "PAR_18", "PAR_19", "PAR_20", "Vibro_Test_Button", "PAR_22", "PAR_23", "PAR_24", "PAR_25", "PAR_26", "PAR_27", "PAR_28", "PAR_29", "PAR_30", "PAR_31", "PAR_32", "Start_Test_Button", "PAR_34", "Programm_counter", "PAR_36", "Circumference_ON_Flag", "PAR_38", "PAR_39", "Pore_Control_Button", "Side_Control_Button", "Axial_Control_Button", "PAR_43", "PAR_44", "PAR_45", "Einfahren_Piston", "PAR_47", "PAR_48", "PAR_49", "PAR_50", "PAR_51", "PAR_52", "PAR_53", "PAR_54", "PAR_55", "PAR_56", "PAR_57", "LinearUpDown_Button", "Linear_Pore_GO", "Linear_Axial_GO", "Linear_Side_GO", "PAR_62", "PAR_63", "PAR_64", "PAR_65", "PAR_66", "PAR_67", "PAR_68", "PAR_69", "Pre_Shearing_Button", "PAR_71", "PAR_72", "PAR_73", "PAR_74", "Circumf_Control_On", "PAR_76", "PAR_77", "PAR_78", "PAR_79", "Modus", "", "", "", "", "", "", "", "", "", "", "", "", "", "", "", "", "", "", "", "", "", "", "", "", "", ""] ("par_enum")
            n832 = property on="Activate Pumps/Piston Controls" class="Bool (strict)"("DisabledEnum"=T7."Enabled" ("Disabled")) -> ()  [unwired: 2 in, 2 out]
            n833 = call "ADwin Set_Par.vi"("Value"=1, "Index"=w1297, "Device No."=w1300) -> ()  [unwired: 6 in, 3 out]
          }
        }
        n834 = local write "Activate Manuel Control"(TRUE ("Activate Manuel Control")) -> ()
        n835 = local write "Activate Pumps/Piston Controls"(FALSE ("Activate Controls")) -> ()
      }
      event "start penetration": Value Change {
        w1303 = u16 33 items=["NaN", "Kp_Position_Vibro", "Ki_Position_Vibro", "PAR_3", "Sinusfrequenz_preSh", "Zylinder_Move_Button", "PAR_6", "PAR_7", "PAR_8", "PAR_9", "PAR_10", "PAR_11", "PAR_12", "Amplitude_PreSh", "Compass_OFF", "PAR_15", "PAR_16", "SollMoog", "PAR_18", "PAR_19", "PAR_20", "Vibro_Test_Button", "PAR_22", "PAR_23", "PAR_24", "PAR_25", "PAR_26", "PAR_27", "PAR_28", "PAR_29", "PAR_30", "PAR_31", "PAR_32", "Start_Test_Button", "PAR_34", "Programm_counter", "PAR_36", "Circumference_ON_Flag", "PAR_38", "PAR_39", "Pore_Control_Button", "Side_Control_Button", "Axial_Control_Button", "PAR_43", "PAR_44", "PAR_45", "Einfahren_Piston", "PAR_47", "PAR_48", "PAR_49", "PAR_50", "PAR_51", "PAR_52", "PAR_53", "PAR_54", "PAR_55", "PAR_56", "PAR_57", "LinearUpDown_Button", "Linear_Pore_GO", "Linear_Axial_GO", "Linear_Side_GO", "PAR_62", "PAR_63", "PAR_64", "PAR_65", "PAR_66", "PAR_67", "PAR_68", "PAR_69", "Pre_Shearing_Button", "PAR_71", "PAR_72", "PAR_73", "PAR_74", "Circumf_Control_On", "PAR_76", "PAR_77", "PAR_78", "PAR_79", "Modus", "", "", "", "", "", "", "", "", "", "", "", "", "", "", "", "", "", "", "", "", "", "", "", "", "", ""] ("par_enum")
        n836 = event-data() -> ("NewVal"=w1302:bool)  [unwired: 1 in, 5 out]
        "Boolean" <- w1302
        "Penetration ongoing" <- w1302
        n837 = Wait (ms)(milliseconds to wait=u32 0) -> ()  [unwired: 1 out]
        n838 = case shown="True" w1302 {
          selector: w1302 -> [w1309 w1311]
          frame False {
            n839 = Not(x=w1309) -> (.not. x?=→"Test ended":bool)
          }
          frame True {
            n840 = property on="Pore Pressure okay:" class="Bool (strict)"("DisabledEnum"=T7."Enabled" ("Disabled")) -> ()  [unwired: 2 in, 2 out]
            n841 = property on="Side Pressure okay:" class="Bool (strict)"("DisabledEnum"=T7."Enabled" ("Disabled")) -> ()  [unwired: 2 in, 2 out]
            n842 = property on="Axial Pressure okay:" class="Bool (strict)"("DisabledEnum"=T7."Enabled" ("Disabled")) -> ()  [unwired: 2 in, 2 out]
            n843 = local write "Interner Kraftsensor [MPa]"(cluster{"Y":dbl[], "Y":dbl[]}[] [] ("Interner Kraftsensor [MPa]")) -> ()
            "Test Flag" <- w1311
            "Test Started" <- w1311
          }
        }
        n844 = local write "Record Data"(w1302) -> ()
        n845 = Select(t=1 ("Value"), s=w1302, f=0 ("Value")) -> (s? t:f=w1307:i32)
        n846 = call "ADwin Set_Par.vi"("Value"=w1307, "Index"=w1303, "Device No."=w1304) -> ()  [unwired: 6 in, 3 out]
      }
      event "SET Pre-Shearing": Value Change {
        w1315 = u16 4 items=["NaN", "Kp_Position_Vibro", "Ki_Position_Vibro", "PAR_3", "Sinusfrequenz_preSh", "Zylinder_Move_Button", "PAR_6", "PAR_7", "PAR_8", "PAR_9", "PAR_10", "PAR_11", "PAR_12", "Amplitude_PreSh", "Compass_OFF", "PAR_15", "PAR_16", "SollMoog", "PAR_18", "PAR_19", "PAR_20", "Vibro_Test_Button", "PAR_22", "PAR_23", "PAR_24", "PAR_25", "PAR_26", "PAR_27", "PAR_28", "PAR_29", "PAR_30", "PAR_31", "PAR_32", "Start_Test_Button", "PAR_34", "Programm_counter", "PAR_36", "Circumference_ON_Flag", "PAR_38", "PAR_39", "Pore_Control_Button", "Side_Control_Button", "Axial_Control_Button", "PAR_43", "PAR_44", "PAR_45", "Einfahren_Piston", "PAR_47", "PAR_48", "PAR_49", "PAR_50", "PAR_51", "PAR_52", "PAR_53", "PAR_54", "PAR_55", "PAR_56", "PAR_57", "LinearUpDown_Button", "Linear_Pore_GO", "Linear_Axial_GO", "Linear_Side_GO", "PAR_62", "PAR_63", "PAR_64", "PAR_65", "PAR_66", "PAR_67", "PAR_68", "PAR_69", "Pre_Shearing_Button", "PAR_71", "PAR_72", "PAR_73", "PAR_74", "Circumf_Control_On", "PAR_76", "PAR_77", "PAR_78", "PAR_79", "Modus", "", "", "", "", "", "", "", "", "", "", "", "", "", "", "", "", "", "", "", "", "", "", "", "", "", ""] ("par_enum")
        w1316 = u16 13 items=["NaN", "Kp_Position_Vibro", "Ki_Position_Vibro", "PAR_3", "Sinusfrequenz_preSh", "Zylinder_Move_Button", "PAR_6", "PAR_7", "PAR_8", "PAR_9", "PAR_10", "PAR_11", "PAR_12", "Amplitude_PreSh", "Compass_OFF", "PAR_15", "PAR_16", "SollMoog", "PAR_18", "PAR_19", "PAR_20", "Vibro_Test_Button", "PAR_22", "PAR_23", "PAR_24", "PAR_25", "PAR_26", "PAR_27", "PAR_28", "PAR_29", "PAR_30", "PAR_31", "PAR_32", "Start_Test_Button", "PAR_34", "Programm_counter", "PAR_36", "Circumference_ON_Flag", "PAR_38", "PAR_39", "Pore_Control_Button", "Side_Control_Button", "Axial_Control_Button", "PAR_43", "PAR_44", "PAR_45", "Einfahren_Piston", "PAR_47", "PAR_48", "PAR_49", "PAR_50", "PAR_51", "PAR_52", "PAR_53", "PAR_54", "PAR_55", "PAR_56", "PAR_57", "LinearUpDown_Button", "Linear_Pore_GO", "Linear_Axial_GO", "Linear_Side_GO", "PAR_62", "PAR_63", "PAR_64", "PAR_65", "PAR_66", "PAR_67", "PAR_68", "PAR_69", "Pre_Shearing_Button", "PAR_71", "PAR_72", "PAR_73", "PAR_74", "Circumf_Control_On", "PAR_76", "PAR_77", "PAR_78", "PAR_79", "Modus", "", "", "", "", "", "", "", "", "", "", "", "", "", "", "", "", "", "", "", "", "", "", "", "", "", ""] ("par_enum")
        n847 = event-data() -> ()  [unwired: 1 in, 6 out]
        n848 = expression code="65536/12000*x"("Amplitude Cycle SOLL") -> (w1320:i32)
        n849 = call "ADwin Set_Par.vi"("Value"=w1320, "Index"=w1316, "Device No."=w1318) -> ("Device No. out"=w1317:u16)  [unwired: 6 in, 2 out]
        n850 = call "ADwin Set_Par.vi"("Value"="Duration of Cycle SOLL", "Index"=w1315, "Device No."=w1317) -> ()  [unwired: 6 in, 3 out]
      }
      event "Start Pre-Shearing": Value Change {
        w1323 = u16 70 items=["NaN", "Kp_Position_Vibro", "Ki_Position_Vibro", "PAR_3", "Sinusfrequenz_preSh", "Zylinder_Move_Button", "PAR_6", "PAR_7", "PAR_8", "PAR_9", "PAR_10", "PAR_11", "PAR_12", "Amplitude_PreSh", "Compass_OFF", "PAR_15", "PAR_16", "SollMoog", "PAR_18", "PAR_19", "PAR_20", "Vibro_Test_Button", "PAR_22", "PAR_23", "PAR_24", "PAR_25", "PAR_26", "PAR_27", "PAR_28", "PAR_29", "PAR_30", "PAR_31", "PAR_32", "Start_Test_Button", "PAR_34", "Programm_counter", "PAR_36", "Circumference_ON_Flag", "PAR_38", "PAR_39", "Pore_Control_Button", "Side_Control_Button", "Axial_Control_Button", "PAR_43", "PAR_44", "PAR_45", "Einfahren_Piston", "PAR_47", "PAR_48", "PAR_49", "PAR_50", "PAR_51", "PAR_52", "PAR_53", "PAR_54", "PAR_55", "PAR_56", "PAR_57", "LinearUpDown_Button", "Linear_Pore_GO", "Linear_Axial_GO", "Linear_Side_GO", "PAR_62", "PAR_63", "PAR_64", "PAR_65", "PAR_66", "PAR_67", "PAR_68", "PAR_69", "Pre_Shearing_Button", "PAR_71", "PAR_72", "PAR_73", "PAR_74", "Circumf_Control_On", "PAR_76", "PAR_77", "PAR_78", "PAR_79", "Modus", "", "", "", "", "", "", "", "", "", "", "", "", "", "", "", "", "", "", "", "", "", "", "", "", "", ""] ("par_enum")
        n851 = event-data() -> ("NewVal"=w1324:bool)  [unwired: 1 in, 5 out]
        n852 = Select(t=1 ("Value"), s=w1324, f=0 ("Value")) -> (s? t:f=w1326:i32)
        n853 = call "ADwin Set_Par.vi"("Value"=w1326, "Index"=w1323, "Device No."=w1322) -> ()  [unwired: 6 in, 3 out]
      }
      event "Activate Pumps/Piston Controls": Value Change {
        n854 = event-data() -> ("NewVal"=w1329:bool)  [unwired: 1 in, 5 out]
        "Pump Control On" <- w1329
        n855 = case shown="True" w1329 {
          tunnel: w1332 -> [_ w1334]
          frame False {
          }
          frame True {
            w1333 = u16 80 items=["NaN", "Kp_Position_Vibro", "Ki_Position_Vibro", "PAR_3", "Sinusfrequenz_preSh", "Zylinder_Move_Button", "PAR_6", "PAR_7", "PAR_8", "PAR_9", "PAR_10", "PAR_11", "PAR_12", "Amplitude_PreSh", "Compass_OFF", "PAR_15", "PAR_16", "SollMoog", "PAR_18", "PAR_19", "PAR_20", "Vibro_Test_Button", "PAR_22", "PAR_23", "PAR_24", "PAR_25", "PAR_26", "PAR_27", "PAR_28", "PAR_29", "PAR_30", "PAR_31", "PAR_32", "Start_Test_Button", "PAR_34", "Programm_counter", "PAR_36", "Circumference_ON_Flag", "PAR_38", "PAR_39", "Pore_Control_Button", "Side_Control_Button", "Axial_Control_Button", "PAR_43", "PAR_44", "PAR_45", "Einfahren_Piston", "PAR_47", "PAR_48", "PAR_49", "PAR_50", "PAR_51", "PAR_52", "PAR_53", "PAR_54", "PAR_55", "PAR_56", "PAR_57", "LinearUpDown_Button", "Linear_Pore_GO", "Linear_Axial_GO", "Linear_Side_GO", "PAR_62", "PAR_63", "PAR_64", "PAR_65", "PAR_66", "PAR_67", "PAR_68", "PAR_69", "Pre_Shearing_Button", "PAR_71", "PAR_72", "PAR_73", "PAR_74", "Circumf_Control_On", "PAR_76", "PAR_77", "PAR_78", "PAR_79", "Modus", "", "", "", "", "", "", "", "", "", "", "", "", "", "", "", "", "", "", "", "", "", "", "", "", "", ""] ("par_enum")
            n856 = call "ADwin Set_Par.vi"("Value"=3, "Index"=w1333, "Device No."=w1334) -> ()  [unwired: 6 in, 3 out]
          }
        }
        n857 = local write "Manuel Control"(FALSE ("Manuel Control")) -> ()
        n858 = local write "Activate Manuel Control"(FALSE ("Activate Manuel Control")) -> ()
        n859 = local write "Activate Pumps/Piston Controls"(TRUE ("Activate Controls")) -> ()
      }
      event "Move": Value Change {
        w1336 = u16 17 items=["NaN", "Kp_Position_Vibro", "Ki_Position_Vibro", "PAR_3", "Sinusfrequenz_preSh", "Zylinder_Move_Button", "PAR_6", "PAR_7", "PAR_8", "PAR_9", "PAR_10", "PAR_11", "PAR_12", "Amplitude_PreSh", "Compass_OFF", "PAR_15", "PAR_16", "SollMoog", "PAR_18", "PAR_19", "PAR_20", "Vibro_Test_Button", "PAR_22", "PAR_23", "PAR_24", "PAR_25", "PAR_26", "PAR_27", "PAR_28", "PAR_29", "PAR_30", "PAR_31", "PAR_32", "Start_Test_Button", "PAR_34", "Programm_counter", "PAR_36", "Circumference_ON_Flag", "PAR_38", "PAR_39", "Pore_Control_Button", "Side_Control_Button", "Axial_Control_Button", "PAR_43", "PAR_44", "PAR_45", "Einfahren_Piston", "PAR_47", "PAR_48", "PAR_49", "PAR_50", "PAR_51", "PAR_52", "PAR_53", "PAR_54", "PAR_55", "PAR_56", "PAR_57", "LinearUpDown_Button", "Linear_Pore_GO", "Linear_Axial_GO", "Linear_Side_GO", "PAR_62", "PAR_63", "PAR_64", "PAR_65", "PAR_66", "PAR_67", "PAR_68", "PAR_69", "Pre_Shearing_Button", "PAR_71", "PAR_72", "PAR_73", "PAR_74", "Circumf_Control_On", "PAR_76", "PAR_77", "PAR_78", "PAR_79", "Modus", "", "", "", "", "", "", "", "", "", "", "", "", "", "", "", "", "", "", "", "", "", "", "", "", "", ""] ("par_enum")
        w1337 = u16 5 items=["NaN", "Kp_Position_Vibro", "Ki_Position_Vibro", "PAR_3", "Sinusfrequenz_preSh", "Zylinder_Move_Button", "PAR_6", "PAR_7", "PAR_8", "PAR_9", "PAR_10", "PAR_11", "PAR_12", "Amplitude_PreSh", "Compass_OFF", "PAR_15", "PAR_16", "SollMoog", "PAR_18", "PAR_19", "PAR_20", "Vibro_Test_Button", "PAR_22", "PAR_23", "PAR_24", "PAR_25", "PAR_26", "PAR_27", "PAR_28", "PAR_29", "PAR_30", "PAR_31", "PAR_32", "Start_Test_Button", "PAR_34", "Programm_counter", "PAR_36", "Circumference_ON_Flag", "PAR_38", "PAR_39", "Pore_Control_Button", "Side_Control_Button", "Axial_Control_Button", "PAR_43", "PAR_44", "PAR_45", "Einfahren_Piston", "PAR_47", "PAR_48", "PAR_49", "PAR_50", "PAR_51", "PAR_52", "PAR_53", "PAR_54", "PAR_55", "PAR_56", "PAR_57", "LinearUpDown_Button", "Linear_Pore_GO", "Linear_Axial_GO", "Linear_Side_GO", "PAR_62", "PAR_63", "PAR_64", "PAR_65", "PAR_66", "PAR_67", "PAR_68", "PAR_69", "Pre_Shearing_Button", "PAR_71", "PAR_72", "PAR_73", "PAR_74", "Circumf_Control_On", "PAR_76", "PAR_77", "PAR_78", "PAR_79", "Modus", "", "", "", "", "", "", "", "", "", "", "", "", "", "", "", "", "", "", "", "", "", "", "", "", "", ""] ("par_enum")
        n860 = event-data() -> ("NewVal"=w1346:bool)  [unwired: 1 in, 5 out]
        n861 = expression code="65336/10*x+32768"("Schieberegler") -> (w1339:dbl)
        n862 = Select(t=1 ("Value"), s=w1346, f=0 ("Value")) -> (s? t:f=w1343:i32)
        n863 = To Long Integer(number=w1339) -> (32bit integer=w1340:i32)
        n864 = call "ADwin Set_Par.vi"("Value"=w1343, "Index"=w1337, "Device No."=w1342) -> ("Device No. out"=w1341:u16)  [unwired: 6 in, 2 out]
        n865 = call "ADwin Set_Par.vi"("Value"=w1340, "Index"=w1336, "Device No."=w1341) -> ()  [unwired: 6 in, 3 out]
      }
      event "Regelung Akiv Porepress", "Regelung Akiv Sidepressure", "Regelung Akiv Axial": Value Change {
        w1349 = u16 42 items=["NaN", "Kp_Position_Vibro", "Ki_Position_Vibro", "PAR_3", "Sinusfrequenz_preSh", "Zylinder_Move_Button", "PAR_6", "PAR_7", "PAR_8", "PAR_9", "PAR_10", "PAR_11", "PAR_12", "Amplitude_PreSh", "Compass_OFF", "PAR_15", "PAR_16", "SollMoog", "PAR_18", "PAR_19", "PAR_20", "Vibro_Test_Button", "PAR_22", "PAR_23", "PAR_24", "PAR_25", "PAR_26", "PAR_27", "PAR_28", "PAR_29", "PAR_30", "PAR_31", "PAR_32", "Start_Test_Button", "PAR_34", "Programm_counter", "PAR_36", "Circumference_ON_Flag", "PAR_38", "PAR_39", "Pore_Control_Button", "Side_Control_Button", "Axial_Control_Button", "PAR_43", "PAR_44", "PAR_45", "Einfahren_Piston", "PAR_47", "PAR_48", "PAR_49", "PAR_50", "PAR_51", "PAR_52", "PAR_53", "PAR_54", "PAR_55", "PAR_56", "PAR_57", "LinearUpDown_Button", "Linear_Pore_GO", "Linear_Axial_GO", "Linear_Side_GO", "PAR_62", "PAR_63", "PAR_64", "PAR_65", "PAR_66", "PAR_67", "PAR_68", "PAR_69", "Pre_Shearing_Button", "PAR_71", "PAR_72", "PAR_73", "PAR_74", "Circumf_Control_On", "PAR_76", "PAR_77", "PAR_78", "PAR_79", "Modus", "", "", "", "", "", "", "", "", "", "", "", "", "", "", "", "", "", "", "", "", "", "", "", "", "", ""] ("par_enum")
        w1348 = u16 41 items=["NaN", "Kp_Position_Vibro", "Ki_Position_Vibro", "PAR_3", "Sinusfrequenz_preSh", "Zylinder_Move_Button", "PAR_6", "PAR_7", "PAR_8", "PAR_9", "PAR_10", "PAR_11", "PAR_12", "Amplitude_PreSh", "Compass_OFF", "PAR_15", "PAR_16", "SollMoog", "PAR_18", "PAR_19", "PAR_20", "Vibro_Test_Button", "PAR_22", "PAR_23", "PAR_24", "PAR_25", "PAR_26", "PAR_27", "PAR_28", "PAR_29", "PAR_30", "PAR_31", "PAR_32", "Start_Test_Button", "PAR_34", "Programm_counter", "PAR_36", "Circumference_ON_Flag", "PAR_38", "PAR_39", "Pore_Control_Button", "Side_Control_Button", "Axial_Control_Button", "PAR_43", "PAR_44", "PAR_45", "Einfahren_Piston", "PAR_47", "PAR_48", "PAR_49", "PAR_50", "PAR_51", "PAR_52", "PAR_53", "PAR_54", "PAR_55", "PAR_56", "PAR_57", "LinearUpDown_Button", "Linear_Pore_GO", "Linear_Axial_GO", "Linear_Side_GO", "PAR_62", "PAR_63", "PAR_64", "PAR_65", "PAR_66", "PAR_67", "PAR_68", "PAR_69", "Pre_Shearing_Button", "PAR_71", "PAR_72", "PAR_73", "PAR_74", "Circumf_Control_On", "PAR_76", "PAR_77", "PAR_78", "PAR_79", "Modus", "", "", "", "", "", "", "", "", "", "", "", "", "", "", "", "", "", "", "", "", "", "", "", "", "", ""] ("par_enum")
        w1347 = u16 40 items=["NaN", "Kp_Position_Vibro", "Ki_Position_Vibro", "PAR_3", "Sinusfrequenz_preSh", "Zylinder_Move_Button", "PAR_6", "PAR_7", "PAR_8", "PAR_9", "PAR_10", "PAR_11", "PAR_12", "Amplitude_PreSh", "Compass_OFF", "PAR_15", "PAR_16", "SollMoog", "PAR_18", "PAR_19", "PAR_20", "Vibro_Test_Button", "PAR_22", "PAR_23", "PAR_24", "PAR_25", "PAR_26", "PAR_27", "PAR_28", "PAR_29", "PAR_30", "PAR_31", "PAR_32", "Start_Test_Button", "PAR_34", "Programm_counter", "PAR_36", "Circumference_ON_Flag", "PAR_38", "PAR_39", "Pore_Control_Button", "Side_Control_Button", "Axial_Control_Button", "PAR_43", "PAR_44", "PAR_45", "Einfahren_Piston", "PAR_47", "PAR_48", "PAR_49", "PAR_50", "PAR_51", "PAR_52", "PAR_53", "PAR_54", "PAR_55", "PAR_56", "PAR_57", "LinearUpDown_Button", "Linear_Pore_GO", "Linear_Axial_GO", "Linear_Side_GO", "PAR_62", "PAR_63", "PAR_64", "PAR_65", "PAR_66", "PAR_67", "PAR_68", "PAR_69", "Pre_Shearing_Button", "PAR_71", "PAR_72", "PAR_73", "PAR_74", "Circumf_Control_On", "PAR_76", "PAR_77", "PAR_78", "PAR_79", "Modus", "", "", "", "", "", "", "", "", "", "", "", "", "", "", "", "", "", "", "", "", "", "", "", "", "", ""] ("par_enum")
        n866 = event-data() -> ()  [unwired: 1 in, 6 out]
        n867 = Select(t=1 ("Value"), s="Regelung Akiv Porepress", f=0 ("Value")) -> (s? t:f=w1352:i32)
        n868 = Select(t=1 ("Value"), s="Regelung Akiv Axial", f=0 ("Value")) -> (s? t:f=w1358:i32)
        n869 = Select(t=1 ("Value"), s="Regelung Akiv Sidepressure", f=0 ("Value")) -> (s? t:f=w1355:i32)
        n870 = call "ADwin Set_Par.vi"("Value"=w1352, "Index"=w1347, "Device No."=w1350) -> ("Device No. out"=w1363:u16)  [unwired: 6 in, 2 out]
        n871 = call "ADwin Set_Par.vi"("Value"=w1355, "Index"=w1348, "Device No."=w1363) -> ("Device No. out"=w1364:u16)  [unwired: 6 in, 2 out]
        n872 = call "ADwin Set_Par.vi"("Value"=w1358, "Index"=w1349, "Device No."=w1364) -> ()  [unwired: 6 in, 3 out]
      }
      event "SET Pump Pressures": Value Change {
        n873 = event-data() -> ()  [unwired: 1 in, 6 out]
        n874 = local read "Linear Control On"() -> (w1366:bool)
        n875 = Not(x=w1366) -> (.not. x?=w1365:bool)
        n876 = case shown="True" w1365 {
          tunnel: w1367 -> [_ w1379]
          frame False {
          }
          frame True {
            n877 = expression code="65536/12000*x+32768"("Soll Pore Pressure") -> (w1376:dbl)
            n878 = expression code="65536/12000*x+32768"("Soll Axial Pressure") -> (w1377:dbl)
            n879 = expression code="65536/12000*x+32768"("Soll Side Pressure") -> (w1378:dbl)
            n880 = To Single Precision Float(number=w1376) -> (single precision float=w1382:sgl)
            n881 = To Single Precision Float(number=w1377) -> (single precision float=w1381:sgl)
            n882 = To Single Precision Float(number=w1378) -> (single precision float=w1380:sgl)
            n883 = call "ADwin Set_FPar.vi"("Value"=w1382, "Index"=T11."Set_Soll_PorePressure" ("Enum"), "Device No."=w1379) -> ("Device No. out"=w1372:u16)  [unwired: 6 in, 2 out]
            n884 = call "ADwin Set_FPar.vi"("Value"=w1381, "Index"=T11."Set_Soll_AxialPressure" ("Enum"), "Device No."=w1372) -> ("Device No. out"=w1371:u16)  [unwired: 6 in, 2 out]
            n885 = call "ADwin Set_FPar.vi"("Value"=w1380, "Index"=T11."Set_Soll_SidePressure" ("Enum"), "Device No."=w1371) -> ()  [unwired: 6 in, 3 out]
          }
        }
      }
      event "SET Vibro Settings": Value Change {
        w1387 = u16 1 items=["NaN", "Kp_Position_Vibro", "Ki_Position_Vibro", "PAR_3", "Sinusfrequenz_preSh", "Zylinder_Move_Button", "PAR_6", "PAR_7", "PAR_8", "PAR_9", "PAR_10", "PAR_11", "PAR_12", "Amplitude_PreSh", "Compass_OFF", "PAR_15", "PAR_16", "SollMoog", "PAR_18", "PAR_19", "PAR_20", "Vibro_Test_Button", "PAR_22", "PAR_23", "PAR_24", "PAR_25", "PAR_26", "PAR_27", "PAR_28", "PAR_29", "PAR_30", "PAR_31", "PAR_32", "Start_Test_Button", "PAR_34", "Programm_counter", "PAR_36", "Circumference_ON_Flag", "PAR_38", "PAR_39", "Pore_Control_Button", "Side_Control_Button", "Axial_Control_Button", "PAR_43", "PAR_44", "PAR_45", "Einfahren_Piston", "PAR_47", "PAR_48", "PAR_49", "PAR_50", "PAR_51", "PAR_52", "PAR_53", "PAR_54", "PAR_55", "PAR_56", "PAR_57", "LinearUpDown_Button", "Linear_Pore_GO", "Linear_Axial_GO", "Linear_Side_GO", "PAR_62", "PAR_63", "PAR_64", "PAR_65", "PAR_66", "PAR_67", "PAR_68", "PAR_69", "Pre_Shearing_Button", "PAR_71", "PAR_72", "PAR_73", "PAR_74", "Circumf_Control_On", "PAR_76", "PAR_77", "PAR_78", "PAR_79", "Modus", "", "", "", "", "", "", "", "", "", "", "", "", "", "", "", "", "", "", "", "", "", "", "", "", "", ""] ("par_enum")
        w1388 = u16 2 items=["NaN", "Kp_Position_Vibro", "Ki_Position_Vibro", "PAR_3", "Sinusfrequenz_preSh", "Zylinder_Move_Button", "PAR_6", "PAR_7", "PAR_8", "PAR_9", "PAR_10", "PAR_11", "PAR_12", "Amplitude_PreSh", "Compass_OFF", "PAR_15", "PAR_16", "SollMoog", "PAR_18", "PAR_19", "PAR_20", "Vibro_Test_Button", "PAR_22", "PAR_23", "PAR_24", "PAR_25", "PAR_26", "PAR_27", "PAR_28", "PAR_29", "PAR_30", "PAR_31", "PAR_32", "Start_Test_Button", "PAR_34", "Programm_counter", "PAR_36", "Circumference_ON_Flag", "PAR_38", "PAR_39", "Pore_Control_Button", "Side_Control_Button", "Axial_Control_Button", "PAR_43", "PAR_44", "PAR_45", "Einfahren_Piston", "PAR_47", "PAR_48", "PAR_49", "PAR_50", "PAR_51", "PAR_52", "PAR_53", "PAR_54", "PAR_55", "PAR_56", "PAR_57", "LinearUpDown_Button", "Linear_Pore_GO", "Linear_Axial_GO", "Linear_Side_GO", "PAR_62", "PAR_63", "PAR_64", "PAR_65", "PAR_66", "PAR_67", "PAR_68", "PAR_69", "Pre_Shearing_Button", "PAR_71", "PAR_72", "PAR_73", "PAR_74", "Circumf_Control_On", "PAR_76", "PAR_77", "PAR_78", "PAR_79", "Modus", "", "", "", "", "", "", "", "", "", "", "", "", "", "", "", "", "", "", "", "", "", "", "", "", "", ""] ("par_enum")
        w1395 = u16 21 items=["NaN", "Kp_Position_Vibro", "Ki_Position_Vibro", "PAR_3", "Sinusfrequenz_preSh", "Zylinder_Move_Button", "PAR_6", "PAR_7", "PAR_8", "PAR_9", "PAR_10", "PAR_11", "PAR_12", "Amplitude_PreSh", "Compass_OFF", "PAR_15", "PAR_16", "SollMoog", "PAR_18", "PAR_19", "PAR_20", "Vibro_Test_Button", "PAR_22", "PAR_23", "PAR_24", "PAR_25", "PAR_26", "PAR_27", "PAR_28", "PAR_29", "PAR_30", "PAR_31", "PAR_32", "Start_Test_Button", "PAR_34", "Programm_counter", "PAR_36", "Circumference_ON_Flag", "PAR_38", "PAR_39", "Pore_Control_Button", "Side_Control_Button", "Axial_Control_Button", "PAR_43", "PAR_44", "PAR_45", "Einfahren_Piston", "PAR_47", "PAR_48", "PAR_49", "PAR_50", "PAR_51", "PAR_52", "PAR_53", "PAR_54", "PAR_55", "PAR_56", "PAR_57", "LinearUpDown_Button", "Linear_Pore_GO", "Linear_Axial_GO", "Linear_Side_GO", "PAR_62", "PAR_63", "PAR_64", "PAR_65", "PAR_66", "PAR_67", "PAR_68", "PAR_69", "Pre_Shearing_Button", "PAR_71", "PAR_72", "PAR_73", "PAR_74", "Circumf_Control_On", "PAR_76", "PAR_77", "PAR_78", "PAR_79", "Modus", "", "", "", "", "", "", "", "", "", "", "", "", "", "", "", "", "", "", "", "", "", "", "", "", "", ""] ("par_enum")
        # "Change Control Parameter to adjust to static and vibro control,\n for smoother control"
        n886 = event-data() -> ()  [unwired: 1 in, 6 out]
        n887 = Multiply(x="Vorschub SOLL", y=78.01) -> (x*y=w1393:dbl)
        n888 = Divide(x=w1393, y=5000.0) -> (x/y=w1392:dbl)
        n889 = expression code="1/x"("Frequency SOLL") -> (w1402:dbl)
        n890 = expression code="x*78"("Amplitude SOLL") -> (w1401:dbl)
        n891 = To Single Precision Float(number=w1392) -> (single precision float=w1406:sgl)
        n892 = To Single Precision Float(number=w1402) -> (single precision float=w1403:sgl)
        n893 = To Single Precision Float(number=w1401) -> (single precision float=w1400:sgl)
        n894 = Select(t=1 ("Value"), s="VibroTest", f=0 ("Value")) -> (s? t:f=w1410:i32)
        n895 = case shown="False" "VibroTest" {
          tunnel: [50 ("Value") 150 ("Value")] -> w1384
          tunnel: [0 ("Value") 10 ("Value")] -> w1383
          frame False {
          }
          frame True {
          }
        }
        n896 = call "ADwin Set_FPar.vi"("Value"=w1403, "Index"=T11."Sinusfrequenz_Vibro" ("Enum"), "Device No."=w1407) -> ("Device No. out"=w1405:u16)  [unwired: 6 in, 2 out]
        n897 = call "ADwin Set_FPar.vi"("Value"=w1406, "Index"=T11."Vorschub" ("Enum"), "Device No."=w1405) -> ("Device No. out"=w1404:u16)  [unwired: 6 in, 2 out]
        n898 = call "ADwin Set_FPar.vi"("Value"=w1400, "Index"=T11."Amplitude_Vibro" ("Enum"), "Device No."=w1404) -> ("Device No. out"=w1399:u16)  [unwired: 6 in, 2 out]
        n899 = call "ADwin Set_Par.vi"("Value"=w1410, "Index"=w1395, "Device No."=w1399) -> ("Device No. out"=w1385:u16)  [unwired: 6 in, 2 out]
        n900 = call "ADwin Set_Par.vi"("Value"=w1384, "Index"=w1387, "Device No."=w1385) -> ("Device No. out"=w1386:u16)  [unwired: 6 in, 2 out]
        n901 = call "ADwin Set_Par.vi"("Value"=w1383, "Index"=w1388, "Device No."=w1386) -> ()  [unwired: 6 in, 3 out]
      }
      event "SET Huang Su": Value Change {
        n902 = event-data() -> ()  [unwired: 1 in, 6 out]
        n903 = call "ADwin Set_FPar.vi"("Value"="SOLL Parameter 1", "Index"=T11."Huang_Su_par_1" ("Enum"), "Device No."=w1430) -> ("Device No. out"=w1417:u16)  [unwired: 6 in, 2 out]
        n904 = call "ADwin Set_FPar.vi"("Value"="SOLL Paramter 2", "Index"=T11."Huang_Su_par_2" ("Enum"), "Device No."=w1417) -> ("Device No. out"=w1429:u16)  [unwired: 6 in, 2 out]
        n905 = call "ADwin Set_FPar.vi"("Value"="SOLL Parameter 3", "Index"=T11."Huang_Su_par_3" ("Enum"), "Device No."=w1429) -> ("Device No. out"=w1428:u16)  [unwired: 6 in, 2 out]
        n906 = call "ADwin Set_FPar.vi"("Value"="SOLL Parameter 4", "Index"=T11."Huang_Su_par_4" ("Enum"), "Device No."=w1428) -> ("Device No. out"=w1427:u16)  [unwired: 6 in, 2 out]
        n907 = call "ADwin Set_FPar.vi"("Value"="SOLL Parameter 5", "Index"=T11."Huang_Su_par_5" ("Enum"), "Device No."=w1427) -> ("Device No. out"=w1426:u16)  [unwired: 6 in, 2 out]
        n908 = call "ADwin Set_FPar.vi"("Value"="SOLL Parameter 6", "Index"=T11."Huang_Su_par_6" ("Enum"), "Device No."=w1426) -> ("Device No. out"=w1425:u16)  [unwired: 6 in, 2 out]
        n909 = call "ADwin Set_FPar.vi"("Value"="SOLL Parameter 7", "Index"=T11."Huang_Su_par_7" ("Enum"), "Device No."=w1425) -> ()  [unwired: 6 in, 3 out]
      }
      event "Set button": Value Change {
        n910 = event-data() -> ()  [unwired: 1 in, 6 out]
        n911 = call "ADwin Get_FPar_Block.vi"("count"=i16 80, "startindex"=i16 1, "Device No."=w1440) -> ("Data"=w1438:sgl[], "Device No. out"=w1439:u16)  [unwired: 2 in, 2 out]
        n912 = case shown="True" "Set button" {
          tunnel: w1439 -> [_ w1444]
          tunnel: w1438 -> [_ w1446]
          frame False {
          }
          frame True {
            (unwired) "Standard value for Intercept"
            (unwired) "Standard value for slope"
            n913 = Decrement(x=T10."Slope_calibration" ("Enum")) -> (x-1=w1453:T10)
            n914 = Decrement(x=T10."Intercept_calibration" ("Enum")) -> (x-1=w1448:T10)
            n915 = Index Array(array=w1446, index=w1453) -> (element=w1449:sgl)
            n916 = Equal?(x=w1449, y="Soll Slope-Strain") -> (x = y?=w1450:bool)
            n917 = case shown="True" w1450 {
              tunnel: "Soll Slope-Strain" -> [w1462 _]
              tunnel: [w1462 w1463] -> w1457
              tunnel: w1449 -> [_ w1463]
              frame False {
              }
              frame True {
              }
            }
            n918 = Index Array(array=w1446, index=w1448) -> (element=w1445:sgl)
            n919 = Equal?(x="Soll Intercept-strain", y=w1445) -> (x = y?=w1456:bool)
            n920 = case shown="True" w1456 {
              tunnel: "Soll Intercept-strain" -> [w1460 _]
              tunnel: [w1460 w1461] -> w1454
              tunnel: w1445 -> [_ w1461]
              frame False {
              }
              frame True {
              }
            }
            n921 = call "ADwin Set_FPar.vi"("Value"=w1457, "Index"=T11."FPAR_18" ("Enum"), "Device No."=w1444) -> ()  [unwired: 6 in, 3 out]
            n922 = call "ADwin Set_FPar.vi"("Value"=w1454, "Index"=T11."FPAR_19" ("Enum"), "Device No."=w1444) -> ()  [unwired: 6 in, 3 out]
          }
        }
      }
      event "Huang Su Calibration File": Value Change {
        n923 = event-data() -> ("NewVal"=w1488:path)  [unwired: 1 in, 5 out]
        n924 = call-poly <vilib>:"Read Delimited Spreadsheet.vi"("file path (dialog if empty)"=w1488) -> ("all rows"=w1472:dbl[][])  [unwired: 9 in, 5 out]
        n925 = Index Array(array=w1472, index (row)=0, index (col)=0 ("disabled index (col)")) -> (element=w1471:dbl)
        n926 = Index Array(array=w1472, index (row)=1, index (col)=0 ("disabled index (col)")) -> (element=w1470:dbl)
        n927 = Index Array(array=w1472, index (row)=4, index (col)=0 ("disabled index (col)")) -> (element=w1467:dbl)
        n928 = Index Array(array=w1472, index (row)=3, index (col)=0 ("disabled index (col)")) -> (element=w1468:dbl)
        n929 = Index Array(array=w1472, index (row)=5, index (col)=0 ("disabled index (col)")) -> (element=w1466:dbl)
        n930 = Index Array(array=w1472, index (row)=2, index (col)=0 ("disabled index (col)")) -> (element=w1469:dbl)
        n931 = Index Array(array=w1472, index (row)=6, index (col)=0 ("disabled index (col)")) -> (element=w1465:dbl)
        n932 = local write "SOLL Parameter 4"(w1468) -> ()
        n933 = local write "SOLL Parameter 5"(w1467) -> ()
        n934 = local write "SOLL Parameter 6"(w1466) -> ()
        n935 = local write "SOLL Parameter 1"(w1471) -> ()
        n936 = local write "SOLL Parameter 3"(w1469) -> ()
        n937 = local write "SOLL Parameter 7"(w1465) -> ()
        n938 = local write "SOLL Paramter 2"(w1470) -> ()
        n939 = call "ADwin Set_FPar.vi"("Value"=w1471, "Index"=T11."Huang_Su_par_1" ("Enum"), "Device No."=w1485) -> ("Device No. out"=w1464:u16)  [unwired: 6 in, 2 out]
        n940 = call "ADwin Set_FPar.vi"("Value"=w1470, "Index"=T11."Huang_Su_par_2" ("Enum"), "Device No."=w1464) -> ("Device No. out"=w1500:u16)  [unwired: 6 in, 2 out]
        n941 = call "ADwin Set_FPar.vi"("Value"=w1469, "Index"=T11."Huang_Su_par_3" ("Enum"), "Device No."=w1500) -> ("Device No. out"=w1499:u16)  [unwired: 6 in, 2 out]
        n942 = call "ADwin Set_FPar.vi"("Value"=w1468, "Index"=T11."Huang_Su_par_4" ("Enum"), "Device No."=w1499) -> ("Device No. out"=w1498:u16)  [unwired: 6 in, 2 out]
        n943 = call "ADwin Set_FPar.vi"("Value"=w1467, "Index"=T11."Huang_Su_par_5" ("Enum"), "Device No."=w1498) -> ("Device No. out"=w1497:u16)  [unwired: 6 in, 2 out]
        n944 = call "ADwin Set_FPar.vi"("Value"=w1466, "Index"=T11."Huang_Su_par_6" ("Enum"), "Device No."=w1497) -> ("Device No. out"=w1496:u16)  [unwired: 6 in, 2 out]
        n945 = call "ADwin Set_FPar.vi"("Value"=w1465, "Index"=T11."Huang_Su_par_7" ("Enum"), "Device No."=w1496) -> ()  [unwired: 6 in, 3 out]
      }
    }
    n946 = Tick Count (ms)() -> (millisecond timer value=w45:u32)
    n947 = Subtract(x=w45, y=w47) -> (x-y=→"Time Loop":u32)
    n948 = property on="Strain curve based on side volume change" class="WFChart (strict)"("XScale.RngStart"=1.0 ("X Scale.Range:Start")) -> ()  [unwired: 2 in, 2 out]
  }
